vi "W7XBolo2021.vi"(1 "FPGA VI Reference In":refnum<k20>) -> (0 "FPGA VI Reference Out":refnum<k20>)   [LabVIEW 2014]
uses:
  W7XBolo_2021.ctl
  <vilib>/Platform/TimedLoop/XDataNode/timing_clust.ctl
  <vilib>/Platform/TimedLoop/XDataNode/nitl_modes.ctl
  <vilib>/Platform/TimedLoop/XDataNode/wakeup.ctl
  <vilib>/userdefined/High Color/nirio_resource_hc.ctl
  <vilib>/Utility/file.llb/Read From Spreadsheet File (I64).vi
  <vilib>/Utility/file.llb/Read From Spreadsheet File (DBL).vi
  <vilib>/FPGAPlugInAG/PCI-7813R/niLvFpga_Open_PCI-7813R.vi
  <vilib>/Utility/error.llb/Error Cluster From Error Code.vi
  <vilib>/rvi/errors/niLvFpgaAdjustHostInterfaceError.vi
  <vilib>/DAQmx/create/channels.llb/DAQmx Create Channel (AO-Voltage-Basic).vi
  <vilib>/DAQmx/write.llb/DAQmx Write (Analog 1D DBL NChan 1Samp).vi
  <vilib>/rvi/interface/common/niFpgaWaitOnOcc.vi
  <vilib>/httpClient/POSTBuffer.vi
  <vilib>/FPGAPlugInAG/PCI-7813R/niLvFpga_Close_PCI-7813R.vi
  <vilib>/Platform/TimedLoop/XDataNode/XDataNode.xnode
  <vilib>/rvi/interface/nirviOpenFPGA/nirviOpenFPGA.xnode
  FPGA Bitfiles/W7XBolo2017_FPGATarget_fmain2014_DACRangeVoltage.lvbitx
  f_main_2014.vi
  <vilib>/rvi/interface/nirviReadWriteControl/nirviReadWriteControl.xnode
  <vilib>/rvi/interface/nirviMethod/nirviMethod.xnode
  <vilib>/rvi/interface/nirviCloseFPGA/nirviCloseFPGA.xnode
  <vilib>/Platform/TimedLoop/XDataNode/XDNodeRunTimeDep.lvlib
  <vilib>/Analysis/NI_AALBase.lvlib
  <vilib>/httpClient/LabVIEWHTTPClient.lvlib
  NiFpgaLv.dll
  <vilib>/FPGAPlugInAG/PCI-7813R/niLvFpga_AcknowledgeIrq_PCI-7813R.vi
  <vilib>/FPGAPlugInAG/PCI-7813R/niLvFpga_ConfigureFifo_PCI-7813R.vi
  <vilib>/rvi/errors/niLvFpgaMergeErrorWithErrorCode.vi
  <resource>/objmgr/daqmx.rc
  <vilib>/DAQmx/configure/timing.llb/DAQmx Timing (Sample Clock).vi
panel:
  out "Time until Acqusition":dbl(slide)=60.0 scale=0.0..60.0
  out "DAQ Timer":dbl
  in  "Tab Control 7":T1(tab)
  out "sample time [s]":sgl=0.0016
  out "No. of Samples:":u32=26000
  out "Measured Time for DAQ [ms]":u32
  out "single channel voltage [V]":dbl format="%#_13g"
  out "experiment acqusition [s]":dbl=40.0
  out "predicted time [ms] to finalize DAQ":dbl
  out "real time P_rad [MW, V]":dbl format="%#_13g"
  in  "single channel signal factor":dbl=1.0
  in  "single channel number":i64
  in  "manual time of data acquisition for experiment [s]":dbl=10.0
  out "f_DAQ [kHz]":dbl=0.625
  in  "skip feedback":bool
  out "loop DAQ timing [ms]":dbl
  in  "local storage only":bool
  in  "Frequency Selection":u16(ring)=1 items=["0.8 ms", "1.0 ms", "1.6 ms", "3.2 ms", "6.4 ms"]
  out "current start time of VI":timestamp
  in  "Trigger Source":i32(slide)=3 scale=0.0..1.0
  out "number of nanoseconds with offset to 1904":i64
  out "start time POSIX [ns]":i64
  out "data acquisition wait\ntime [ms]":i32=-1
  out "Countdown Time [s]":dbl
  out "Calibration Time [s]":dbl
  out "Total wait time  [s]":dbl
  in  "time before experiment [s]":T2=5.0
  in  "time between VI start and points of interest [s]":dbl=60.0
  in  "time after experiment [s]":dbl=5.0
  out "Downtime after T0 until DAQ [ns]":i64
  out "DAQ start (POSIX) [ns]":i64
  out "final trigger time":i64
  out "Pre-samples (If -1, then no trigger) detected)":i32
  out "actual T_DAQ [ms]":dbl
  in  "DAC and AD Settings":i32(slide) scale=0.0..1.0
  in  "Global DAC Range [mV] Setting":u8(knob)=3 scale=0.0..3.0
  in  "DAC settings file location":path=path "C:/QSB_files/dac_settings.dat"
  out "input DAC settings":i64[](array[numeric])=[3, 3, 3, 3, 3, 3, 3, 3, 3, 3, 3, 3, 3, 3, 3, 3, 3, 3, 3, 3, 3, 3, 3, 3, 3, 3, 3, 3, 3, 3, 3, 3, 3, 3, 3, 3, 3, 3, 3, 3, 3, 3, 3, 3, 3, 3, 3, 3, 3, 3, 3, 3, 3, 3, 3, 3, 3, 3, 3, 3, 3, 3, 3, 3, 3, 3, 3, 3, 3, 3, 3, 3, 3, 3, 3, 3, 3, 3, 3, 3, 3, 3, 3, 3, 3, 3, 3, 3, 3, 3, 3, 3, 3, 3, 3, 3, 3, 3, 3, 3, 3, 3, 3, 3, 3, 3, 3, 3, 3, 3, 3, 3, 3, 3, 3, 3, 3, 3, 3, 3, 3, 3, 3, 3, 3, 3, 0, 0]
  out "kbolott_and_volume":dbl[][](array[numeric])=[[1e-05, 1e-05], [9.8364458e-05, 1.8160732], [0.00029863964, 770.25441], [0.00053910452, 1653.5432], [0.00071569496, 2554.7619], [0.00083348142, 3356.1809], [0.00092645429, 4021.9678], [0.00099241932, 4570.4466], [0.0010332482, 4989.6792], [0.0010552469, 5170.4882], [0.0010669981, 5192.5645], [0.001071534, 5152.6222], [0.0010766644, 5109.6704], [0.0010841289, 5094.9972], [0.0010884845, 5078.237], [0.0010888843, 5058.9416], [0.0010882289, 5056.581], [0.0010872861, 5078.1684], [0.0010832221, 5096.5196], [0.0010760805, 5113.7904], [0.0010685167, 5141.4566], [0.0010644166, 5189.7831], [0.0010539441, 5182.7365], [0.0010337779, 5034.6928], [0.00098716411, 4625.8518], [0.00091599422, 4090.3707], [0.00082376071, 3438.9665], [0.00070194108, 2659.5109], [0.00051785958, 1753.3355], [0.00030745544, 937.82125], [0.00014081292, 59.55205], [1e-05, 1e-05], [0.0, 0.0], [0.0, 0.0], [0.0, 0.0], [0.0, 0.0], [0.0, 0.0], [0.0, 0.0], [0.0, 0.0], [0.0, 0.0], [0.0, 0.0], [0.0, 0.0], [0.0, 0.0], [0.0, 0.0], [0.0, 0.0], [0.0, 0.0], [0.0, 0.0], [0.0, 0.0], [0.0019134875, 3474.3085], [0.0020594744, 3690.1455], [0.002175929, 3861.3028], [0.0022530617, 3956.5918], [0.0023492529, 4057.9903], [0.0024581424, 4205.0841], [0.0025383764, 4324.9746], [0.0025876415, 4417.9525], [0.0026676725, 4566.0612], [0.0027635964, 4770.6296], [0.0028188521, 4914.295], [0.0028263806, 4970.0105], [0.0028491244, 5014.7926], [0.0028762033, 5060.279], [0.0028430703, 4969.1072], [0.0027058578, 4592.2853], [0.0019047772, 4936.5706], [0.0023594746, 6388.5028], [0.0025094117, 6336.5413], [0.002569351, 6048.9284], [0.0026367277, 5794.3031], [0.002714522, 5668.1597], [0.0027530637, 5505.217], [0.0027520905, 5312.6378], [0.0027781484, 5183.8321], [0.0028283925, 5165.5044], [0.0028425709, 5118.655], [0.00281436, 5016.5122], [0.0027996491, 4909.784], [0.0027993913, 4845.125], [0.0027603692, 4728.4661], [0.0026886073, 4585.7454], [0.0026437627, 4495.4419], [0.0026242501, 4486.7206], [0.0025685332, 4434.986], [0.0024747416, 4324.8822], [0.0023915919, 4209.8149], [0.002319616, 4111.844], [0.0022042921, 3923.4955], [0.0020485146, 3644.5259], [0.0024033884, 3597.1969], [0.002066694, 2566.1598], [0.0017718795, 1878.4004], [0.0015136288, 1414.3006], [0.0013043692, 1094.5581], [0.0011378765, 882.65731], [0.00097324167, 712.97006], [0.00080739571, 571.52867], [0.0, 0.0], [0.0, 0.0], [0.0, 0.0], [0.0, 0.0], [0.0, 0.0], [0.0, 0.0], [0.0, 0.0], [0.0, 0.0], [0.0, 0.0], [0.0, 0.0], [0.0, 0.0], [0.0, 0.0], [0.0, 0.0], [0.0, 0.0], [0.0, 0.0], [0.0, 0.0], [0.0, 0.0], [0.0, 0.0], [0.0, 0.0], [0.0, 0.0], [0.0, 0.0], [0.0, 0.0], [0.0, 0.0], [0.0, 0.0], [0.0, 0.0], [0.0, 0.0], [0.0, 0.0], [0.0, 0.0], [0.0, 0.0], [0.0, 0.0], [0.0, 0.0], [0.0, 0.0]]
  in  "Path to kbolott and volume data file":path=path "C:/QSB_files/kbolott_and_volume_all_PV_new.dat"
  out "final channel\nselection size":i32
  out "final channel selection":i64[][](array[numeric])=[[0], [1], [2], [3], [4], [5], [6], [7], [8], [9], [10], [11], [12], [13], [14], [15], [16], [17], [18], [19], [20], [21], [22], [23], [24], [25], [26], [27], [28], [29], [30], [31]]
  in  "Read Channel Selection from file":bool
  in  "channel selection input":i32[][](array[numeric])=[[0]]
  out "file import":i64[][](array[numeric])
  in  "Path to channel selection file":path=path "C:/QSB_files/short.channel_selection.dat"
  out "taum [s]":dbl[](array[numeric])=[0.11537597448635277, 0.11755685958822219, 0.1164214694473907, 0.11697577239117866, 0.110451, 0.12010942076824872, 0.11766714993048435, 0.11910426529905502, 0.10999582403545866, 0.11118469600664964, 0.10580731993585431, 0.11217289808087993, 0.11223398365603839, 0.11204749607224823, 0.11263624992738425, 0.11091290284745299, 0.11721868902521211, 0.11737061531613151, 0.11788987597885038, 0.11600007869942867, 0.11334307549251021, 0.11228572042130423, 0.1129521332802642, 0.11724104097990388, 0.11740306056822605, 0.11529467898123245, 0.11828175507687082, 0.11829012392284373, 0.11773460668621359, 0.1155776803231521, 0.11650421728110884, 0.11571658330095998, 0.11068789319935994, 0.10986016888144867, 0.10999340462233435, 0.11095550249493497, 0.11143937038853975, 0.11095468517729823, 0.11130783288802211, 0.11084408945769118, 0.10830137260394793, 0.10662335345199567, 0.10535002662491703, 0.10738515206651872, 0.10772145508062766, 0.1053368317440755, 0.10408446186375701, 0.10449038510758271, 0.11178895597256559, 0.11021628063681403, 0.11220331344682449, 0.11111721341359461, 0.10889811436206044, 0.11638094730098773, 0.11290278568076087, 0.11205006536853761, 0.1094907553786962, 0.11634433136641531, 0.11037702264320227, 0.1104223688763365, 0.11352480237507033, 0.11341744936097128, 0.10916961452972393, 0.11332789199343518, 0.11107001747086552, 0.1083853978889723, 0.11029711206697901, 0.11063487469805744, 0.10926615257922916, 0.10988377001368325, 0.10782095764307568, 0.1073886205272185, 0.10829341805096283, 0.10953345610425252, 0.10953147401563214, 0.10933747673483066, 0.1093210854374169, 0.10892908051404164, 0.10841565534876087, 0.10934867623657209, 0.11431979794745441, 0.11469548527952493, 0.11256319960938391, 0.11004758193350624, 0.1086775698186096, 0.10860163257332957, 0.10972644811806966, 0.1244329993560779, 0.10848514148619942, 0.10753497988240919, 0.11378450261362759, 0.11397799701939393, 0.10865166632049855, 0.10955778865143037, 0.11184264538711042, 0.11080028199806266, 0.11230419705417591, 0.11150150302047147, 0.10940920103499238, 0.0, 0.11018788195565775, 0.1109851624674225, 0.10888498891279576, 0.10950524535111039, 0.11209787924272374, 0.11180887164622381, 0.1110290995583749, 0.11040609393156747, 0.1103438351320269, 0.1101975468642728, 0.10923728746964355, 0.0, 0.11021638606642407, 0.0, 0.0, 0.0, 0.0, 0.0, 0.0, 0.0, 0.5609466646481899, 0.0, 0.0, 0.0, 0.0, 0.0, 0.0, 0.4058686463981613, 0.11537597448635277]
  out "kappa [A²]":dbl[](array[numeric])=[0.0008396193201719739, 0.0008193409803026575, 0.0008327489337370494, 0.0008094925878469488, 0.00039367506543457065, 0.0008063058560714545, 0.0008451910365158945, 0.0007992358755606012, 0.0008323076933152601, 0.0008570762215527662, 0.0007628861690345087, 0.0008061906602308296, 0.0008540424353779365, 0.0008301118976821594, 0.0008577435335519969, 0.0008553747566925557, 0.000838644207815748, 0.0008273548270536888, 0.0008111923709406437, 0.0008317040544888235, 0.0002062919117538751, 0.0007971782754034694, 0.0007777938427968141, 0.0007983063012770449, 0.0007902138174646686, 0.0007777700527572154, 0.0008086241703327105, 0.0007894905085128677, 0.0008499052168857277, 0.0008231536154986703, 0.0008290108212352768, 0.0008015771948583539, 0.0004219784890145567, 0.0008028223447312654, 0.0007908997677950409, 0.0007688640721813007, 0.0007923143974006498, 0.0007943700234243013, 0.000794807683089336, 0.0007644407575630641, 0.0008256914284962689, 0.0008464663657085921, 0.0008525498714753285, 0.0008605939917038706, 0.0008075301142063146, 0.0008582080819176783, 0.0008833831995156997, 0.0008817750426330745, 0.0008736825873144331, 0.0008712555197947145, 0.0008599116319459445, 0.0008597288697454142, 0.0008850439198466119, 0.0008360600624626481, 0.0008729149198757765, 0.0008652970161905564, 0.000878176403644396, 0.000814669724061475, 0.0008492936703496222, 0.0008335090067364612, 0.0009020306039280142, 0.0009060889736233363, 0.000873120149823901, 0.0008865804075398461, 0.0008218319952538781, 0.0008647381541051004, 0.0008535415687509321, 0.000868609807906937, 0.0008544506047017487, 0.0008552184337763689, 0.0008772351584693919, 0.0008899531428744609, 0.0009049492537694576, 0.000908105157129488, 0.0009441675693280472, 0.0008666158415307141, 0.0008904383660716827, 0.00090533600441176, 0.0009193630525411423, 0.0009209094258700529, 0.0008671616817531277, 0.0008573033056411677, 0.0008894545060438134, 0.0008393076570230061, 0.0008809839906701387, 0.0008713273912310079, 0.0008529389904228485, 0.0008798583497112145, 0.0007606961064025662, 0.0007618681674480262, 0.0008830002472907413, 0.0008434447500347438, 0.0008157810403546725, 0.0008170412330426688, 0.000817539692314199, 0.0008060567476264818, 0.0007745714382802376, 0.0007738842512393123, 0.0007910139604008742, -1.9640688433259297e-10, 0.000780575223559956, 0.0007962779122750964, 0.000790630439080113, 0.0008189866992119251, 0.0008220353590981327, 0.0008259174124746273, 0.0008237041516630779, 0.0008128375228315313, 0.0008025139618430593, 0.0007891459070721132, 0.0007835394415130632, 1.4659311061625464e-11, 0.0007713911232202254, -1.136328152026204e-11, 7.33972615530204e-11, -5.807996136265078e-12, 1.50989391544806e-10, -2.091237015882531e-11, -2.2968171315336452e-11, 3.2003514158147334e-12, -1.18410213996469e-13, 3.9907860061368183e-13, 1.2900003061146403e-11, -7.996494711993759e-11, 1.2728268766879732e-10, -2.7124534936566837e-11, -1.0618681361847593e-11, 1.1300143559461795e-05]
  out "roh [Ohm]":dbl[](array[numeric])=[964.4665558152926, 984.0412138536651, 1001.0627256989599, 1012.7898525309201, 986.7279110070629, 993.5830261423998, 1133.718466702734, 1026.065541032409, 981.7525515631839, 976.6051330676225, 975.1369773387203, 983.6003740876943, 945.3052421117454, 944.0131212191011, 937.9865397688445, 924.775520494105, 1002.3909240348048, 1016.474188810108, 1008.3024841336951, 997.8517562562979, 1396.1357804303618, 1011.7052948010587, 1006.0858095523904, 1000.525119034801, 1016.071205963885, 1008.5531713944379, 1001.2101495655734, 1012.9539707105694, 909.9522463978296, 921.8611396886308, 930.8535575645451, 937.6736260749049, 1835.253905213153, 905.3151174073253, 915.4686408360067, 932.2842954450018, 878.6376527118448, 888.8892103361444, 896.5962281010978, 917.195767017641, 953.2009542047422, 949.8476734916919, 945.7180214798805, 934.1303098026676, 944.4309270141721, 922.393020385211, 908.2770101975661, 902.8479184676862, 997.7185120044248, 1004.633250147941, 1012.2992174178987, 1022.8972656361334, 988.1138139759116, 1012.5096483256309, 926.7526927543831, 940.6499588809413, 987.4981539235332, 1030.6093168535383, 996.69488158787, 998.6770565199763, 937.2653710614366, 942.0245103372197, 975.0990877775471, 954.8089604337308, 987.3564837474132, 941.2547128561528, 982.5095895382428, 979.0417371038707, 995.2373497220817, 994.8506309175264, 989.7979732647505, 986.9344569144992, 979.4724674608722, 951.8026661804106, 928.3096097998925, 980.4648125251251, 967.8736951300871, 960.399052288677, 950.3474867516031, 931.7877057694141, 925.6104123406642, 925.2905333073797, 925.2586242376997, 996.0089625341668, 969.8590336679081, 973.5395443351913, 978.7443359479869, 1329.6132687126426, 951.8837808548863, 946.7262849537287, 933.7058147126331, 940.8228530266879, 876.367589172054, 864.1420943242144, 855.6188139335973, 854.7591574173059, 955.1936774096923, 969.1826763753277, 970.8033011923455, 0.0, 935.2179320514933, 937.6581182076873, 940.1867678977421, 939.4080093580444, 850.4194498630884, 857.7406858104588, 867.3881837894808, 884.270800315495, 892.6618762043922, 899.3995556852765, 915.5186423922648, 0.0, 919.5685811076437, 0.0, 0.0, 0.0, 0.0, 0.0, 0.0, 0.0, 0.0, 0.0, 0.0, 0.0, 0.0, 0.0, 0.0, 0.0]
  in  "load calibration values from file?":bool
  in  "file location":path=path "C:/QSB_files/default_calibs.dat"
  in  "Clear all Values \nfrom Beginning":bool
  in  "Cancel Button":bool
  in  "Tab Control":T3(tab)=enum."offsets"
  out "real time P_rad array":dbl[](array[numeric])
  out "all plot":cluster{cluster{dbl, "element":dbl}[]}[](graph)
  out "full P_rad [MW] HBC":dbl[](array[numeric])
  out "single channel voltage array":dbl[](array[numeric])
  out "full P_rad [MW] VBC":dbl[](array[numeric])
  out "nsample array [s]":dbl[](array[numeric])
  in  "Tab Control 4":enum32{"1 to 64", "65 to 128"}(tab)
  out "Raw 33-64":T4={"Channels 33 - 40"={"tstart"=-1.0, "FPGSampleTime"=0.0007999999797903001, []}, "Channels 41 - 48"={"tstart"=-1.0, "FPGSampleTime"=0.0007999999797903001, []}, "Channels 49 - 56"={"tstart"=-1.0, "FPGSampleTime"=0.0007999999797903001, []}, "Channels 57 - 64"={"tstart"=-1.0, "FPGSampleTime"=0.0007999999797903001, []}}
  out "Raw 1-32":T5={"Channels 1- 8"={"tstart"=-1.0, "FPGSampleTime"=0.0007999999797903001, []}, "Channels 9 - 16"={"tstart"=-1.0, "FPGSampleTime"=0.0007999999797903001, []}, "Channels 17 - 24"={"tstart"=-1.0, "FPGSampleTime"=0.0007999999797903001, []}, "Channels 25 - 32"={"tstart"=-1.0, "FPGSampleTime"=0.0007999999797903001, []}}
  out "Raw 97 - 128":T6
  out "Raw 65 - 97":T7={"Channels 65 - 71"={"tstart"=-1.0, "FPGSampleTime"=0.0007999999797903001, []}, "Channels 73 - 80"={"tstart"=0.0, "FPGSampleTime"=0.0, []}, "Channels 81 - 88"={"tstart"=0.0, "FPGSampleTime"=0.0, []}, "Channels 89- 96"={"tstart"=0.0, "FPGSampleTime"=0.0, []}}
  in  "Tab Control 2":T8(tab)
  out "Offset 1-32":T5
  out "Offset 33-64":T4
  out "Offset 65 - 96":T7
  out "Offset 97 - 128":T6
  out "mean [µV]":dbl[](array[numeric])=[-1.0868261423893273, -7.990200226195156, -8.872255865484476, -10.064653429202735, 0.15312744089169428, -0.4802685623290017, 79.99756187200546, 3.8797607778105885, 7.466437983792275, -11.855529976077378, -14.755810303613544, 11.95750002656132, -8.815307591110468, 8.149265284650028, 8.269059924408793, -11.019621591083705, -12.155327236279845, 11.87860367167741, -6.231015749275684, -15.075639658607543, 0.0, 6.344313888344914, 3.639809527201578, 3.0874096516054124, 8.76988005079329, -7.264990275725722, -7.70126957911998, 7.049201687797904, -5.80584733793512, 7.595500641036779, 6.073078604415059, -7.225483466871083, 79.99756187200546, -6.537163232453167, -9.645444056019187, 12.285051323473454, 13.197480607777834, -16.88525196351111, 14.07000007852912, -16.506511248648167, 1.317087397328578, 1.08624508313369, 2.3623975100927055, -2.897617152426392, 15.83140585012734, -16.25518073886633, -15.617426818236709, 17.98624993674457, 3.7837353413924575, -9.388547336682677, 9.94124523550272, -6.121635691262782, -2.0081029990687966, 4.30479721352458, -4.133330153301358, -5.317026526667178, -11.655625252053142, -5.538921014405787, -8.435971749015152, 6.669389561749995, -1.8595410124398768, -2.53979729488492, -10.409289598464966, -6.292082520201802, 3.7355981967411935, -18.137234115973115, -4.700468767434359, 3.342731858836487, -12.631655607372522, 9.172075293958187, 6.846901873126626, -3.930554289836436, 1.7484496866818517, -16.44031921029091, -10.512590528465807, 12.021665379405022, -8.448259128257632, 13.529167225584388, 17.693245006725192, -4.355747113935649, -3.6723168953321874, 5.37680432992056, 10.893774300813675, -4.947795500513166, -8.853234618902206, -8.510966784320772, -8.374758321791887, -5.658979562111199, -2.2409302280284464, 2.758493692148477, 8.601340346038342, -7.293605968821794, 12.404243350028992, -12.006000837311149, -11.754489918239415, 9.409597270190716, -13.37633796967566, 12.256328152492642, 11.935139204375446, 0.7362792931962758, 5.519568009767681, -8.845417500473559, -12.099643769674003, 14.686545513570309, 3.346308583393693, -8.303696025162935, -8.65569824911654, 7.810756796039641, 1.5121240087319165, 0.011279296885732037, 1.614531259285286, -5.667829567566514, -3.9232958229258657, -6.169724114239216, -5.436516118235886, -6.255625001620501, -6.266003428958356, -4.911455085966736, -5.73839355725795, -4.92482177214697, -6.417814949993044, -5.6116870157420635, -5.524570322595537, -7.1842724503949285, -6.247446291614324, -5.192988283466548, -5.514289560727775, 0.007548827956270543] format="%10.6f"
  out "peak to peak [µV]":dbl[](array[numeric])=[7.324153557419777, 7.3248520493507385, 4.881992936134338, 7.3248520493507385, 7.32421176508069, 7.32421176508069, 0.0, 7.324153557419777, 7.324386388063431, 4.882924258708954, 4.882924258708954, 4.882924258708954, 7.323920726776123, 4.882924258708954, 4.882924258708954, 7.3248520493507385, 4.882924258708954, 7.323920726776123, 4.882924258708954, 7.323920726776123, 0.0, 12.207310646772385, 7.324153557419777, 7.324153557419777, 4.882924258708954, 7.324386388063431, 7.323920726776123, 7.323920726776123, 7.323920726776123, 7.323920726776123, 7.323920726776123, 7.324386388063431, 0.0, 7.324386388063431, 4.882924258708954, 4.882924258708954, 7.323920726776123, 7.323920726776123, 4.882924258708954, 24.413689970970154, 7.324153557419777, 4.882807843387127, 7.324153557419777, 7.324153557419777, 12.207776308059692, 9.765848517417908, 9.765848517417908, 9.765848517417908, 9.765848517417908, 7.3248520493507385, 9.765848517417908, 7.324386388063431, 7.324153557419777, 7.323920726776123, 7.324386388063431, 7.324386388063431, 4.882924258708954, 7.324386388063431, 9.765848517417908, 7.324386388063431, 7.324269972741604, 4.8826914280653, 9.765848517417908, 63.47661837935448, 4.882924258708954, 7.325783371925354, 7.324386388063431, 7.324153557419777, 4.882924258708954, 9.765848517417908, 7.323920726776123, 7.324386388063431, 7.324153557419777, 4.881992936134338, 4.882924258708954, 4.882924258708954, 7.323920726776123, 4.882924258708954, 4.883855581283569, 4.882924258708954, 7.324386388063431, 7.324386388063431, 7.323920726776123, 7.324386388063431, 7.323920726776123, 7.323920726776123, 4.882924258708954, 12.207310646772385, 4.8826914280653, 7.324386388063431, 4.882924258708954, 7.323920726776123, 4.882924258708954, 7.323920726776123, 7.323920726776123, 4.882924258708954, 4.882924258708954, 7.3248520493507385, 4.882924258708954, 7.32421176508069, 7.324386388063431, 4.882924258708954, 4.882924258708954, 7.323920726776123, 7.324386388063431, 7.323920726776123, 4.882924258708954, 4.882924258708954, 7.324269972741604, 7.324218586290954, 7.324269972741604, 78.12492549419403, 4.882924258708954, 124.51177462935448, 80.56638762354851, 107.42200538516045, 114.74592611193657, 119.62885037064552, 117.18738824129105, 75.68346336483955, 83.00784975290298, 61.03515625, 83.00784975290298, 80.56638762354851, 80.56638762354851, 75.68346336483955, 63.47661837935448, 4.882812390860636] format="%10.6f"
  out "standard deviation [µV]":dbl[](array[numeric])=[1.3036026797496636, 1.3420327341534157, 1.064632711189032, 1.3183644605739115, 1.370580330128604, 1.3863993208065881, 0.0, 1.3756086966919314, 1.3033635303128535, 1.3645315377351082, 1.0907459947011133, 1.2888566517284963, 1.3362613716194949, 1.1741803584062915, 1.2708577363467628, 1.3353586601127052, 1.1919876577257686, 1.3709838960885252, 1.2104925828693935, 1.133633608207629, 0.0, 3.0599605659652336, 1.381189113773974, 1.3710090729521511, 1.1825139240426916, 1.3291962023482355, 1.2972019555536811, 1.5752294600651209, 1.4348073556120489, 1.5350307313927734, 1.339050112533554, 1.4943583204888495, 0.0, 1.4508038195058017, 1.2325495603810572, 1.289912993666556, 1.3433062875107393, 1.3398822432734163, 1.534045727376026, 3.1309945215657233, 1.3451440535092256, 1.1094863880052617, 1.2848454782475338, 1.4392275103567735, 2.1646380895538133, 1.5764686908727295, 1.8587372491098588, 1.7701595206338636, 1.4747643858198207, 1.7496186198255672, 1.531828101370379, 1.3635429383539241, 1.3363276218458022, 1.510814829492694, 1.4399577231091554, 1.4124317371976478, 1.413580499133295, 1.3668612458750313, 1.6918175690194857, 1.1771696442371267, 1.666194415475469, 1.2881820616939266, 1.6825268941850453, 9.285962098288044, 1.2657962842879769, 1.5227901644120807, 1.2887960355191643, 1.3713397757888555, 0.9409861463314614, 1.5747829733155034, 1.4190235941294134, 1.2472383190291216, 1.295969883093782, 1.2892305818095295, 1.3174003964127896, 0.9534221803559357, 1.3315109646280372, 1.2489669475442673, 1.349904662109497, 1.4628494605003626, 1.1866585970205008, 1.3284762503162553, 1.3591765604379664, 1.440899156716539, 1.20561778948312, 1.4840990676246344, 1.377787118468021, 2.9371469283422225, 1.190473906695344, 1.5904378429312183, 1.2088317344047321, 1.3065369246410496, 1.2079090266634622, 1.4006134268721806, 1.256254801125801, 1.2249039770452999, 1.340159935658495, 1.4548630995535106, 1.390209079178451, 1.640652499453038, 1.2936869882511064, 1.2595058622741677, 1.2444275335713273, 1.460819197867702, 1.240339655773447, 1.236295738635732, 1.3148643594347451, 1.1965755092732067, 1.9037334286600238, 1.354045523248285, 1.343098779957647, 10.648064571198674, 1.085492843026454, 17.76111356002071, 15.186209919625934, 19.587547605945343, 21.06199734827501, 23.357782004272384, 18.34000258364854, 12.885928124829098, 18.63512720438761, 12.776721724893239, 13.06902962785174, 14.7813618767708, 14.660597879483435, 15.094471148412042, 10.816437200629686, 0.9119755118192763] format="%10.7f"
  out "offsets [V]":sgl[](array[numeric])=[-0.0010868261, -0.0079902, -0.008872256, -0.010064653, 0.00015312745, -0.00048026856, 0.07999756, 0.0038797609, 0.0074664378, -0.01185553, -0.014755811, 0.0119575, -0.008815307, 0.008149265, 0.0082690595, -0.011019622, -0.012155327, 0.011878604, -0.0062310155, -0.01507564, 0.0, 0.0063443137, 0.0036398096, 0.0030874095, 0.00876988, -0.0072649904, -0.0077012694, 0.0070492015, -0.0058058472, 0.0075955004, 0.0060730786, -0.0072254837, 0.07999756, -0.006537163, -0.009645444, 0.012285051, 0.013197481, -0.016885253, 0.0140700005, -0.016506512, 0.0013170874, 0.001086245, 0.0023623975, -0.0028976172, 0.015831405, -0.016255181, -0.0156174265, 0.01798625, 0.0037837354, -0.009388547, 0.009941245, -0.006121636, -0.002008103, 0.0043047974, -0.00413333, -0.0053170267, -0.011655625, -0.005538921, -0.008435972, 0.0066693895, -0.001859541, -0.0025397972, -0.01040929, -0.0062920824, 0.0037355982, -0.018137233, -0.004700469, 0.0033427319, -0.012631656, 0.009172075, 0.006846902, -0.0039305543, 0.0017484496, -0.016440319, -0.01051259, 0.012021665, -0.008448259, 0.0135291675, 0.017693246, -0.0043557473, -0.003672317, 0.005376804, 0.010893774, -0.0049477955, -0.008853234, -0.008510967, -0.008374758, -0.0056589795, -0.0022409302, 0.0027584936, 0.00860134, -0.007293606, 0.012404243, -0.012006001, -0.0117544895, 0.009409597, -0.013376338, 0.012256328, 0.011935139, 0.0007362793, 0.005519568, -0.008845418, -0.012099644, 0.014686545, 0.0033463086, -0.008303696, -0.008655698, 0.0078107566, 0.001512124, 1.1279297e-05, 0.0016145313, -0.0056678294, -0.003923296, -0.0061697243, -0.005436516, -0.006255625, -0.0062660035, -0.004911455, -0.0057383934, -0.0049248217, -0.006417815, -0.005611687, -0.00552457, -0.0071842726, -0.0062474464, -0.005192988, -0.0055142897, 7.548828e-06]
  in  "Tab Control 5":T9(tab)
  out "MessCal 17-32":T10
  out "MessCal 1-16":T11
  out "MessCal 49 - 64":T12
  out "MessCal 33 - 49":T13
  out "MessCal 81 - 96":T14
  out "MessCal 65 - 80":T15
  out "MessCal 113 - 128":T16
  out "MessCal 97 - 112":T17
  out "rohM [Ohm]":dbl[](array[numeric])=[955.9210569003584, 975.2225867678288, 992.437036560495, 1003.9150041232155, 964.6709267361214, 984.9572576185153, 1109.7902651791405, 1017.3971751835443, 973.4625288588265, 968.2502632137221, 966.3109252226336, 974.9039174556738, 937.1961165636667, 935.629152331029, 929.8777653560232, 916.6273213641874, 993.8600077425886, 1007.747220175482, 999.538757797739, 989.259326518511, 1376.2474702792624, 1002.9820261662712, 997.0827639584581, 991.8298513828715, 1007.3959263962993, 999.731688473045, 992.5694713810915, 1004.2278313387544, 901.7408614557748, 913.5263201644023, 922.6000347220167, 929.1324124673284, 1861.6154176027044, 1093.927196836436, 1007.9363359277321, 1036.4338892880046, 870.0841248686661, 1050.5167797933268, 835.6422839385561, 972.7302854337263, 859.3011786817983, 961.6092048210389, 1047.3928187757283, 988.832793437985, 1048.3205426549248, 914.332942804887, 900.3157849297525, 895.00814421823, 1071.5906890853698, 1240.680912945196, 1118.5865173282953, 1136.2368012115553, 979.6020495367086, 1184.5954182960481, 917.6449067403735, 1078.5806173219855, 979.3199545918619, 1128.0894920220258, 1107.186057046148, 1058.3166942556252, 1023.6083043326868, 933.59856277125, 966.8256448468209, 946.8606222101016, 979.3205494354647, 933.3840253846747, 974.5533501983803, 971.1794214902197, 987.0554817952572, 986.5749021706774, 981.6986292217362, 978.7347622591474, 971.5484218656636, 944.047973258107, 920.6032902860329, 972.4402748798641, 959.984233512531, 952.591197650364, 942.5919944057227, 924.0279269016532, 914.8529393815768, 917.1478717227278, 917.2337651779903, 987.7775960990439, 961.9031159853596, 965.4373993129607, 970.4632555320065, 1320.2877978597037, 943.1885046031139, 937.9468788829204, 925.7648958682478, 932.8248830697123, 867.8130427511578, 855.5281600301191, 847.1255690825355, 846.1703092127094, 946.4268675021895, 960.4551490506069, 962.1034228215849, 0.0, 926.3189738746476, 928.9034427126842, 931.5953365503219, 930.8922256947712, 841.8622295070686, 849.6900749449139, 858.8923632084177, 875.6587455837807, 884.1647613529192, 890.7709945330058, 906.8409537813054, 0.0, 910.8341169118078, 0.0, 0.0, 0.0, 0.0, 0.0, 0.0, 0.0, 0.0, 0.0, 0.0, 0.0, 0.0, 0.0, 0.0, 0.0]
  out "kappaM [A²]":dbl[](array[numeric])=[0.0009300671270220562, 0.0008996956373935807, 0.0009113297442037162, 0.0008867590824243674, 0.0009228130637662335, 0.000892376467301951, 0.0009770254811961566, 0.0008792308275001902, 0.0009310256041664582, 0.0009423185323272868, 0.0008572434937303331, 0.0008920046513574609, 0.0009420929356066393, 0.000917506962215698, 0.0009460997409387052, 0.0009375108227429941, 0.0009243758742815039, 0.0009114349813263648, 0.000900921530637464, 0.0009125939448337885, 0.00024194293733649212, 0.0008862811148346745, 0.000860786457985191, 0.0008899499474378734, 0.0008705292947452343, 0.0008562533252789487, 0.0008845638677383653, 0.0008733756860620295, 0.0009371291360660496, 0.0009161990069047479, 0.0009134962955644435, 0.000899493342343606, 0.00048738710715928865, 0.0009162872261249577, 0.0009180994946649499, 0.0008862330742697767, 0.0008788280646144513, 0.000923989577633034, 0.0007960035497604953, 0.0008432936364276662, 0.0008626191144435472, 0.0008753403360820782, 0.0009785187528356617, 0.0009920297175945603, 0.0009357728927457351, 0.0009432876940863556, 0.0009737159021657041, 0.0009829677334712832, 0.0009797149193563025, 0.0009656693192116038, 0.0009657204661571637, 0.0009613114786807839, 0.0009574110075363582, 0.0009381886977305131, 0.0009666490144497014, 0.0009794202295580398, 0.0009619800496901404, 0.0009109830431199077, 0.0009578361472746666, 0.0009379291618002864, 0.001016572914013983, 0.0009750425932505828, 0.0009435677239603997, 0.0009695879318732844, 0.0008913866589398846, 0.0009419361616918934, 0.0009250842516270034, 0.0009429046775538786, 0.0009248119474557008, 0.0009298684481160537, 0.000983883219096257, 0.0009529385496771803, 0.00097924891843905, 0.0009817402563716065, 0.0010247538574068172, 0.0009415670186613855, 0.0009827266209943746, 0.0009926770422248304, 0.0009977894534251687, 0.0010016701651269853, 0.0009429727126362719, 0.0009280049111574535, 0.0009664607320996164, 0.000917092855553135, 0.0009689593754395974, 0.0009492630365830234, 0.0009304943986612507, 0.0009838563142093555, 0.0008327174235962352, 0.0008401872142169503, 0.0009608982361607494, 0.0009139859734154169, 0.0008951925851238197, 0.0008976799685850949, 0.0008951491596994188, 0.0008807724921218027, 0.0008598244382888369, 0.0008631925259468964, 0.000869388233684094, -3.087356377393487e-10, 0.000862230960556987, 0.0008818386198612574, 0.000875693256825492, 0.0009093335647258491, 0.0009117694962109967, 0.000915854945030498, 0.0009176622004345077, 0.000899838713726951, 0.0008882426814116755, 0.0008802823610482786, 0.0008643029460286225, 4.560949191370883e-11, 0.0008497040644528844, -2.015502496075528e-12, -1.3937728135220623e-10, -5.142335332617439e-12, -2.4405360432876065e-10, -3.025693723352094e-11, 5.446823850795443e-11, -9.461258601384958e-13, -1.11152298414936e-16, -1.7779007167808036e-13, -1.247134363192558e-12, 9.029112608459833e-11, 2.859966433855044e-10, 4.025476559655337e-11, -6.6296064908001744e-12, 2.7789638144048405e-05] format="%10.4e"
  out "TauM":dbl[](array[numeric])=[0.10247326273143675, 0.10385139756960429, 0.10373232144795708, 0.10311875959492485, 0.1040387663981229, 0.1046650716638566, 0.10127197371489062, 0.10433939668939028, 0.09961240211936159, 0.10113688577012743, 0.09820100289764892, 0.10095901838579123, 0.10145991266213297, 0.10133898562095205, 0.10130127833216106, 0.09956334469474118, 0.10358378126227558, 0.1033444650149854, 0.10368122845865657, 0.1024629201687842, 0.10726822954303422, 0.10182022977214773, 0.10234341921814957, 0.10309722284273504, 0.1042952251760315, 0.10251907726247211, 0.10376892017069193, 0.10390613836510422, 0.10393962152806514, 0.10278682866750612, 0.1029066416867304, 0.102809145991027, 0.10885131092677319, 0.09862497604372066, 0.10044854636642224, 0.1011397796494332, 0.10002902352125999, 0.09964990042145319, 0.10015936689391987, 0.10006472096945454, 0.09839726301474191, 0.0989699304142558, 0.1002391552504395, 0.10013350870556857, 0.10080436633835735, 0.09779852218595043, 0.09742571115181148, 0.09710433370493086, 0.10444501045101653, 0.1003366401072974, 0.10437315691375147, 0.10384291417884778, 0.10124021541103015, 0.10550745222701648, 0.1035137865735804, 0.10352859881892808, 0.1012417667717822, 0.1059159267079176, 0.10317764912629153, 0.10345604684447908, 0.1049337703539443, 0.10334536377187596, 0.1011439242990685, 0.10281039287381427, 0.10222071286894058, 0.10128943771143158, 0.10126644136767568, 0.10213051552429299, 0.10166794227392674, 0.10164755793457868, 0.10028065773083647, 0.1039274155284877, 0.10062166309448936, 0.10100667896022858, 0.10122793031614634, 0.1020869722455638, 0.10086834901007827, 0.10107073060568635, 0.10100593381229647, 0.1013148799331511, 0.10336010473304796, 0.104020047148851, 0.10319519163947051, 0.1023647743297228, 0.10121262984849082, 0.10131571623308212, 0.10129251089534078, 0.10505043416568437, 0.10066202738446095, 0.10001990246198598, 0.10320829246582676, 0.10342094956544687, 0.10072458787609094, 0.10113661913958252, 0.10213104126735983, 0.10141193462449195, 0.10097352152629059, 0.1005352087055146, 0.09991412160243203, 0.0, 0.09971962753116924, 0.10038664478845472, 0.0996831725438015, 0.0987164166127979, 0.10070743969491262, 0.10083769719722958, 0.09991070137880578, 0.09976037466686079, 0.09975950391708734, 0.0997863315853558, 0.09952725945462769, 0.0, 0.09982037400508142, 0.0, 0.0, 0.0, 0.0, 0.0, 0.0, 0.0, 0.0, 0.0, 0.0, 0.0, 0.0, 0.0, 0.0, 0.0] caption="tauM [s]" format="%10.4f"
  out "AmplitudeMeas":dbl[](array[numeric])=[4.884814572518217e-05, 4.7976679783762886e-05, 4.524764340004093e-05, 4.5151806191065595e-05, 4.809080266257478e-05, 4.7145047982970675e-05, 3.146231756322816e-05, 4.3987625115634926e-05, 4.655055771375242e-05, 4.66273477175114e-05, 5.1615426947301555e-05, 4.843928946738043e-05, 5.074259168837904e-05, 5.235508979961122e-05, 5.155588261265355e-05, 5.399794598550638e-05, 4.443179014704798e-05, 4.3474037919468324e-05, 4.4937934344410205e-05, 4.556235086224266e-05, 7.358960331887751e-05, 4.528620525296725e-05, 4.7375341050864565e-05, 4.642857602638946e-05, 4.5595717685851076e-05, 4.7302741586246765e-05, 4.6625975104004555e-05, 4.581918862013139e-05, 5.634340629289198e-05, 5.576445138256422e-05, 5.452694873767264e-05, 5.4394617922290445e-05, 1.5640753900925838e-05, 3.4876244036040754e-05, 4.3131880431277286e-05, 4.157013788164736e-05, 6.594026050113745e-05, 3.846074258536254e-05, 8.092036434813877e-05, 5.15919193318786e-05, 6.938738199638531e-05, 5.117058828178776e-05, 3.656914680495611e-05, 4.190030926295942e-05, 3.8177482970664205e-05, 5.400781436437592e-05, 5.4404204763341695e-05, 5.470539183413758e-05, 3.440187451106315e-05, 2.3688059308740418e-05, 3.1179877554395444e-05, 3.0056387787071678e-05, 4.451276294761954e-05, 2.758635976953778e-05, 5.2189063074364834e-05, 3.382999969429794e-05, 4.433078241643989e-05, 3.2349556560738134e-05, 3.2300748490518005e-05, 3.7152975410132973e-05, 3.735580097349016e-05, 4.948433878422281e-05, 4.6742566329426626e-05, 4.79882648013434e-05, 4.790771836666737e-05, 5.1287893849813555e-05, 4.671903980322345e-05, 4.623427665213439e-05, 4.521107284722498e-05, 4.501779229445353e-05, 4.30551070148025e-05, 4.4828312823474215e-05, 4.44446374507222e-05, 4.774895836610016e-05, 4.8769768288348895e-05, 4.6145596903899056e-05, 4.567972066843394e-05, 4.612705469829869e-05, 4.7154624740959475e-05, 4.944003667941568e-05, 5.394723576121702e-05, 5.448269442335658e-05, 5.225966317746918e-05, 4.551186565071207e-05, 4.610146443391865e-05, 4.6630362792763434e-05, 4.69519837192857e-05, 1.9681004304892295e-05, 5.6612358154279806e-05, 5.691291067414257e-05, 5.132973551498099e-05, 5.296970989083297e-05, 6.514064070696284e-05, 6.736516743145396e-05, 6.92823951303374e-05, 7.06443959549654e-05, 5.430635287521875e-05, 5.2067117003992196e-05, 5.145931439129173e-05, -3.1793762011223885e-07, 5.7242295451644905e-05, 5.554183170240005e-05, 5.552348413500266e-05, 5.353198650115e-05, 6.907674687371533e-05, 6.715920529459659e-05, 6.520750725303529e-05, 6.332147469482486e-05, 6.259754438105115e-05, 6.198157003306498e-05, 6.0316992950063626e-05, 3.495440865528331e-07, 6.0686411438686236e-05, -7.284208164373995e-07, -3.0307954598728734e-07, -3.3162749704529687e-07, -3.250653244446207e-07, -3.4500887828612614e-07, 3.5391304443528806e-07, -5.696407161148624e-07, 3.827735480530181e-07, 4.345734938552804e-07, 1.1320226330949104e-06, 2.005101510462144e-06, 3.0673371184281807e-07, 1.2170619844306492e-06, -3.398933905177686e-07, 2.9714440268932945e-07]
  out "DampingMeas":dbl[](array[numeric])=[-9.758643116700723, -9.629143404928858, -9.640196864790152, -9.697556525391104, -9.61180177947633, -9.554285724005522, -9.874400224639485, -9.584107554090206, -10.038910604743169, -9.887589403067894, -10.183195389992717, -9.905009141221385, -9.856109410719231, -9.86787063115469, -9.871543740258218, -10.043857034594167, -9.654021004195494, -9.67637695792412, -9.644947449660622, -9.759628149897827, -9.322424768825114, -9.821231028821972, -9.771023947015639, -9.699582320712988, -9.58816665204165, -9.754282097562905, -9.636796820811824, -9.624070490293954, -9.620970187292688, -9.728872978801503, -9.717545763899397, -9.726761081035322, -9.186843883513017, -10.139419446415864, -9.955345658782756, -9.887306492718903, -9.997098489994375, -10.035132958193246, -9.984088668003597, -9.993532089149152, -10.16288430553378, -10.104079045163786, -9.976141533730807, -9.986666930251976, -9.920205208606001, -10.225103382427779, -10.26423095276946, -10.298201551319856, -9.574416199316559, -9.966448935609424, -9.581007507767039, -9.629930052595677, -9.87749775067201, -9.47800348593706, -9.660548928805468, -9.659166755931894, -9.87734639453879, -9.441450696623575, -9.692021561530053, -9.665940566076877, -9.529820539440967, -9.676292806007195, -9.88690133322432, -9.726643115033745, -9.782753142038072, -9.872697712558626, -9.874939678873723, -9.791392855175962, -9.835942162630502, -9.837914656480084, -9.972012775226327, -9.62210014474851, -9.938217767887062, -9.900335406470996, -9.87869649094757, -9.795569189715636, -9.913912637750073, -9.894061257965607, -9.900408443907281, -9.870218477876234, -9.674912797183572, -9.613531500990536, -9.690373980734156, -9.768985537729442, -9.8801898685662, -9.8701370051952, -9.872398177918972, -9.519237192516607, -9.93423265935898, -9.998010149830575, -9.68914392543709, -9.669220831966737, -9.928062463061918, -9.887615470118313, -9.791342451725214, -9.86077234107405, -9.903586453995555, -9.946764052872032, -10.008595221195026, -0.04313763282748088, -10.028116076621238, -9.961484439561707, -10.031783444297911, -10.130027348160011, -9.929752985771879, -9.916926187277847, -10.008937843490424, -10.02402009153829, -10.024107586091501, -10.0214125934133, -10.047498599676386, -0.6129351216480721, -10.017994923051424, 0.5637780520462315, 0.10978744631452035, 0.5025353454646939, 0.1910230592818031, 0.31086905931373493, 0.2701712879890733, 0.3997070190467916, -0.1402110488088746, -0.36927368560800944, -0.9431888525901574, -0.46217550051667494, -0.33808673480660545, -0.45825903308817845, 0.2851028761639094, -0.17618214991090886]
  in  "Tab Control 15":enum32{"kappaM [A²]", "rohM [Ohm]", "tauM [s]"}(tab)
  out "kappa_meas":cluster{cluster{dbl, dbl}[]}[](graph)
  out "Rmeas":cluster{cluster{dbl, dbl}[]}[](graph)
  out "tau_meas":cluster{cluster{dbl, dbl}[]}[](graph)
  in  "Tab Control 3":T9(tab)=enum."97 to 128"
  out "RefCal 17-32":T10
  out "RefCal 1-16":T11
  out "RefCal 49 - 64":T12
  out "RefCal 33 - 48":T13
  out "RefCal 65 - 80":T15
  out "RefCal 81 - 96":T14
  out "RefCal 113 - 128":T16
  out "RefCal 97 - 112":T17
  out "tauR [s]":dbl[](array[numeric])=[0.10292315835357112, 0.10199272403695953, 0.10475723294798765, 0.10414819613838391, 0.10387907456908113, 0.10420736881237311, 0.103706568442645, 0.10454999926363777, 0.10067406983111478, 0.10102975505384852, 0.09874353117086729, 0.10040584588306813, 0.10153735621262386, 0.10099019339023692, 0.10045519629639574, 0.1012778636584879, 0.10386355092876007, 0.10372072386082845, 0.10420809088364472, 0.10260629843982476, 0.1479397245408231, 0.10298761609630228, 0.10199112190395622, 0.10378008083073056, 0.10403768235155286, 0.10287961748698402, 0.10443967781666794, 0.10349133443663402, 0.10389037347180505, 0.10292103911369532, 0.10381016378004426, 0.10291167813587834, 0.10095931716806164, 0.09778559469706383, 0.10070172494088425, 0.10101362262178354, 0.10089590213958652, 0.10068417571048587, 0.10027342486802274, 0.1001580148556835, 0.09844078753380402, 0.09855035919543022, 0.10141076521650685, 0.09942661978605821, 0.100044898453749, 0.09843709497312675, 0.0981706617700702, 0.09739033951036816, 0.10579066150165929, 0.10003676894960246, 0.10330538590073358, 0.1043865432442743, 0.1018657436251196, 0.10506556777663303, 0.1039941797472394, 0.10383520947481932, 0.10231334831583622, 0.1061930390378222, 0.10374353015321205, 0.10333403635897148, 0.10431471177356995, 0.10320469195416845, 0.10192370966573754, 0.1032954320172502, 0.1023703130382756, 0.10130836278464572, 0.1020846673388746, 0.10178346111061455, 0.1018337998015322, 0.1018370724659081, 0.10192632813002919, 0.1001119276380221, 0.10098331608408057, 0.10123109259340747, 0.10129713566118832, 0.10216660844261771, 0.10117214382327544, 0.10081211888977323, 0.10198174919879018, 0.1017954675749366, 0.10512035510575353, 0.10258538460215058, 0.10201683357819019, 0.10238920479886968, 0.10211647468588146, 0.10136271634450558, 0.10197441111867332, 0.10437309491921805, 0.10013944794913852, 0.10096667914558943, 0.10278444976940188, 0.10443784509167334, 0.1014058881666478, 0.1018136137122912, 0.10197066776866164, 0.10287778507695343, 0.10113021738229896, 0.1006644626432808, 0.09960874275205062, 0.0, 0.10045362499432091, 0.09997878995335553, 0.09968196495402348, 0.09929009836131342, 0.10129697478598067, 0.10074502421507037, 0.09994878726727208, 0.10010044264701065, 0.09958730925413367, 0.10026435038467114, 0.10027859691998338, 0.0, 0.09991786391447231, 0.0, 0.0, 0.0, 0.0, 0.0, 0.0, 0.0, 0.0, 0.0, 0.0, 0.0, 0.0, 0.0, 0.0, 0.0] caption="TauM" format="%10.4f"
  out "kappaR [A²]":dbl[](array[numeric])=[0.0009394546099408418, 0.0009123589959054041, 0.0008944834435273222, 0.0008770375520480372, 0.0009239963605895957, 0.0008890166300778485, 0.000870129447553066, 0.0008803438703556952, 0.0009107267410723152, 0.0009482118897726593, 0.0008393896084479604, 0.0009035861563965376, 0.0009331871645677263, 0.0009165298742846952, 0.0009516053712712882, 0.0009263278749958205, 0.0009128662815217666, 0.0009141818400495597, 0.000909789371266667, 0.0009059436540468002, 0.0006415370912951529, 0.0008770271810778616, 0.0008565132360134204, 0.000876052272304057, 0.0008638409404951507, 0.0008565665929339299, 0.0008752621730157705, 0.0008723574002536088, 0.0009386669831268589, 0.0009024637518016725, 0.0009106667364475278, 0.0008776276917126037, 0.0009485343911843268, 0.0009151723308720066, 0.0009102916414683612, 0.0008907100933340703, 0.0008832933059746842, 0.0009116353873268474, 0.0007958923399951672, 0.0008390839738911967, 0.0008560973972353745, 0.0008799561494103719, 0.0009830927394652617, 0.0009984988903108173, 0.0009570093031431591, 0.0009303145524909112, 0.0009567590358007552, 0.0009837178264969402, 0.0009843129272350832, 0.0009650264028644321, 0.0009811549948605396, 0.0009642750489135812, 0.000950546683123411, 0.0009431266396382227, 0.0009370548549423619, 0.0009861255596051212, 0.000936829703479727, 0.0009133902647257256, 0.000940402507731474, 0.0009449250051295195, 0.001020427897586195, 0.0009849350172889812, 0.000930313608683439, 0.0009687273302019695, 0.0008970028098137427, 0.0009378049457091181, 0.0009124758988977847, 0.0009386195899888698, 0.0009190062218545321, 0.0009333611210404984, 0.0009621798885820149, 0.0009586958426847128, 0.0009811222363501687, 0.0009835686640004752, 0.0010203977936138304, 0.0009337778675467259, 0.0009650559425072165, 0.000973981534077398, 0.0009635053537147022, 0.0010018111126099767, 0.000933161139102181, 0.0009446919394286867, 0.0009889617815545281, 0.0009054358331810502, 0.000939122203155497, 0.0009357326744797564, 0.0009347689539899098, 0.0009859635267754768, 0.0008285938918540566, 0.0008263493838778397, 0.0009610579572422135, 0.0009149809143467651, 0.0008962067788812194, 0.0008856272930870661, 0.0008865350962852511, 0.0008786825089554866, 0.0008531311914735494, 0.0008533859891198841, 0.000872109802646621, 0.0, 0.0008760398523230332, 0.0008698446766384849, 0.0008609903717441008, 0.000917336684185368, 0.0009109179911288096, 0.0009047951430703002, 0.0009040380219105915, 0.000904172339632746, 0.0008882497394240699, 0.0008680572225687603, 0.0008687146922181975, 0.0, 0.0008532428573888429, 0.0, 0.0, 0.0, 0.0, 0.0, 0.0, 0.0, 0.0, 0.0, 0.0, 0.0, 0.0, 0.0, 0.0, 0.0] format="%10.4e"
  out "rohR [Ohm]":dbl[](array[numeric])=[956.2989572160357, 978.5138361759319, 995.9442187225984, 1008.0612479776369, 964.5336300299568, 985.0055115328407, 1004.8872607781536, 1015.6348863841632, 970.1222108210756, 972.8684444511352, 972.0803308285506, 969.9635452071706, 940.4965770667643, 932.2838721500672, 926.5761973455059, 920.756728380192, 998.751618187049, 1002.645484442407, 1002.1053527592385, 995.4297427495583, 1392.257972279243, 1000.0408343872241, 995.4529906568217, 990.3892250143565, 1003.5638240476669, 1002.755127561061, 995.6971596757855, 1001.1091797833428, 903.8420325055714, 910.3815361921353, 920.1088899075633, 931.7459469784179, 926.9075240023208, 1097.1836989420253, 1012.1223252323492, 1031.6051502195423, 865.2324519228997, 1057.9499680316503, 830.6654020548849, 979.3828138858556, 858.7479663219067, 961.53773070908, 1046.5061278621247, 990.1818658724626, 1041.8555133387686, 920.4757081714, 906.1159528601476, 888.1121509383381, 1071.2473928215386, 1245.318995975411, 1113.9727919488028, 1138.9397717522506, 979.7240200508488, 1182.6306291953856, 918.4536457413244, 1080.9233560093503, 983.3365096085471, 1130.6202259639726, 1110.4178701762908, 1055.259800570412, 1024.0859269214227, 933.9597358439946, 970.2526336349497, 948.688421711014, 977.030945115165, 939.7429827751671, 975.6234204561338, 969.0235139852646, 991.5720828131982, 982.0367763892792, 978.0405497108788, 979.6777686598148, 970.1725242379728, 949.966637895026, 923.9935019418235, 966.6891261032167, 962.6515819439619, 946.3793377124441, 934.8713576429398, 924.9716858464726, 928.4919275009711, 914.4598679734345, 912.3387254132956, 989.0534287066091, 964.630020750574, 968.107058502228, 973.1214347577088, 1322.3134987131093, 943.3174526896092, 936.0860474391636, 921.668159103662, 934.9229484511964, 862.561130391307, 859.1572250426, 850.5913397590812, 841.993390963776, 951.6785132163961, 955.3620398061908, 957.1846902791526, 0.0, 924.2040160146751, 932.2074075745045, 936.2132007459005, 925.1445913956145, 840.5542054379803, 852.5611786313709, 861.92116699029, 872.8124148817855, 883.4410079612458, 890.6206279927792, 906.1980264444114, 0.0, 911.9549549093531, 0.0, 0.0, 0.0, 0.0, 0.0, 0.0, 0.0, 0.0, 0.0, 0.0, 0.0, 0.0, 0.0, 0.0, 0.0]
  in  "Tab Control 16":enum32{"kappaR [A²]", "rohR [Ohm]", "tauR [s]"}(tab)
  out "kappa_ref":cluster{cluster{dbl, dbl}[]}[](graph)
  out "Rref":cluster{cluster{dbl, dbl}[]}[](graph)
  out "tau_ref":cluster{cluster{dbl, dbl}[]}[](graph)
  out "AmplitudeRef":dbl[](array[numeric])=[4.83014587536764e-05, 4.6886431105424204e-05, 4.5693921662628275e-05, 4.517336188419036e-05, 4.804578645848785e-05, 4.732052700919899e-05, 4.591462943673503e-05, 4.413030415869068e-05, 4.803400604811675e-05, 4.5764127555017504e-05, 5.1926839092191126e-05, 4.844133421698066e-05, 5.0773250468378564e-05, 5.2898883999341665e-05, 5.1723916149280746e-05, 5.4034050297686275e-05, 4.443055762286131e-05, 4.391815377009177e-05, 4.41959369950802e-05, 4.5166208362337964e-05, 2.628711953935288e-05, 4.612446065855897e-05, 4.781954999466934e-05, 4.73577474417948e-05, 4.641429262683351e-05, 4.691436453050651e-05, 4.674626195998729e-05, 4.6247085662862315e-05, 5.591386395664718e-05, 5.71360494619428e-05, 5.508233623570734e-05, 5.537540853138137e-05, 5.184686539494168e-05, 3.464714893108982e-05, 4.304066034843922e-05, 4.186592788449239e-05, 6.654390853603804e-05, 3.827642570591026e-05, 8.217344319552989e-05, 5.0945399304559355e-05, 7.00443785224149e-05, 5.090667782131817e-05, 3.647718767429366e-05, 4.1477186668356055e-05, 3.7926234807134086e-05, 5.384012806677711e-05, 5.4482177824064506e-05, 5.575719576332571e-05, 3.426765322518995e-05, 2.3469140674068706e-05, 3.101904807703416e-05, 2.9775225526311722e-05, 4.48253977632181e-05, 2.7561335436541732e-05, 5.374860766352849e-05, 3.340579086181422e-05, 4.5060685174598033e-05, 3.207264098912411e-05, 3.265621632092434e-05, 3.715427754438422e-05, 3.7167284327577756e-05, 4.892923984171913e-05, 4.69877213718141e-05, 4.7792882712276665e-05, 4.7892459709366624e-05, 5.062311324567015e-05, 4.72418138266528e-05, 4.671766101666083e-05, 4.4964820509280574e-05, 4.538680988286842e-05, 4.447204942236181e-05, 4.444314438676128e-05, 4.4521553353020214e-05, 4.689518527497801e-05, 4.852066998003178e-05, 4.725895157287671e-05, 4.619814121076748e-05, 4.7830609481071116e-05, 4.9912436159152e-05, 4.9303191216113085e-05, 5.248639863617162e-05, 5.390665512798289e-05, 5.1755140399867196e-05, 4.595398847286793e-05, 4.724546540554775e-05, 4.697955221093076e-05, 4.640292765818111e-05, 1.9557850098468774e-05, 5.6880091327731996e-05, 5.818509150594947e-05, 5.1910718940191176e-05, 5.260497806350283e-05, 6.60825738985255e-05, 6.757006053362133e-05, 6.924763793780627e-05, 7.171523683417315e-05, 5.3962547953454505e-05, 5.340882211661125e-05, 5.198165527945615e-05, 3.027720682637124e-07, 5.665392367532961e-05, 5.580997330836715e-05, 5.577479800735162e-05, 5.390989869183955e-05, 6.941708190788706e-05, 6.741760220225805e-05, 6.562096213228938e-05, 6.353826032916368e-05, 6.272859579521672e-05, 6.29018904503205e-05, 6.0113453361722795e-05, 3.5028168483663885e-07, 6.023790853414281e-05, 2.8927221930409144e-07, 2.486289955552982e-07, -2.439049094821873e-07, 7.23586744803015e-07, 2.843265647087974e-07, -2.943067221248818e-07, -1.3893047297828158e-07, 1.52036607637842e-06, -4.831843245690887e-07, 2.8401836255779593e-07, 5.212745134813822e-07, 2.936511341194766e-07, -3.1446729839724297e-07, -5.269124205051759e-07, -2.8657011109605934e-07]
  out "DampingRef":dbl[](array[numeric])=[-9.715986333850228, -9.804620961370007, -9.54588024004513, -9.60170254577697, -9.626577866122451, -9.596250355390074, -9.64259077334191, -9.56480159773466, -9.933044344760715, -9.898074081907883, -10.127245685285297, -9.959579456803663, -9.848592058138232, -9.901951530441108, -9.954686635119137, -9.873825966274635, -9.628016672431114, -9.641274788457812, -9.596183861736481, -9.745990404151138, -6.759509679390107, -9.70990530613811, -9.80477497778373, -9.635760465739468, -9.611901932041397, -9.720098348212819, -9.574905063910549, -9.662644756139297, -9.625530899370492, -9.7161863950413, -9.632968137097121, -9.717070191778047, -9.904979828016792, -10.226455165486932, -9.930316492463641, -9.89965485887198, -9.91120529966152, -9.932047344514872, -9.97273207049798, -9.984223443734265, -10.1583908972346, -10.147096450627346, -9.860886049573244, -10.057668682207598, -9.99551216959156, -10.158771957593824, -10.186342660520552, -10.267958865607406, -9.452630183093385, -9.996324456498492, -9.680037408319665, -9.579778857701095, -9.81684287978245, -9.517866044620602, -9.615922760586471, -9.630644605599858, -9.773895747337383, -9.41681308926318, -9.639155314294445, -9.677353515216478, -9.586375526499499, -9.689481951499685, -9.811259846011648, -9.68097020817921, -9.768456990320098, -9.87085342723118, -9.795790357825778, -9.824778889305371, -9.819922284633769, -9.819606708890507, -9.811007796967655, -9.988819749987554, -9.90262588690771, -9.878387898236747, -9.871947449182878, -9.787933799932823, -9.884143621062048, -9.919442335037001, -9.80567609259896, -9.823620086659078, -9.512905459594164, -9.747977295968886, -9.802303844625367, -9.766654619150236, -9.792739154735619, -9.865560396006549, -9.806381709194124, -9.581013198602312, -9.986074623737755, -9.90425760718588, -9.729098149024603, -9.575073088900112, -9.861360302437527, -9.821869232790796, -9.806741702120414, -9.720271477967685, -9.888241377151752, -9.933992331967696, -10.03927940832697, 0.14407521411619148, -9.954842346968906, -10.002121454625962, -10.031904973595093, -10.071497727407145, -9.871963127356873, -9.926048534815983, -10.005123897360653, -9.989965813901058, -10.04144009401973, -9.973634658414786, -9.972217708609776, -0.5310057319448518, -10.008220360435047, -0.017021375659971562, 0.21017647963836042, 0.4071453428214994, -0.8393246724893615, 0.40768462336107564, -0.33375657807565773, -0.6945284591593672, -0.3690780149016432, 0.7771858472497803, 0.1857421941408096, -0.07975159462366016, 0.4921816211993282, -0.23036123110343212, 0.179801318904817, -0.4810505364746216]
  in  "Tab Control 6":T18(tab)
  out "RefStatus 65-96":bool[](array[boolean])
  out "RefStatus 33-64":bool[](array[boolean])
  out "RefStatus 1-32":bool[](array[boolean])
  out "RefStatus 97-128":bool[](array[boolean])=[FALSE, FALSE, FALSE, TRUE, FALSE, FALSE, FALSE, FALSE, FALSE, FALSE, FALSE, FALSE, FALSE, FALSE, FALSE, TRUE, FALSE, TRUE, TRUE, TRUE, TRUE, TRUE, TRUE, TRUE, TRUE, TRUE, TRUE, TRUE, TRUE, TRUE, TRUE, TRUE]
  out "MessStatus 1-32":bool[](array[boolean])
  out "MessStatus 33-64":bool[](array[boolean])=[TRUE, FALSE, FALSE, FALSE, FALSE, FALSE, FALSE, FALSE, FALSE, FALSE, FALSE, FALSE, FALSE, FALSE, FALSE, FALSE, FALSE, FALSE, FALSE, FALSE, FALSE, FALSE, FALSE, FALSE, FALSE, FALSE, FALSE, FALSE, FALSE, FALSE, FALSE, FALSE]
  out "MessStatus 97-128":bool[](array[boolean])=[FALSE, FALSE, FALSE, TRUE, FALSE, FALSE, FALSE, FALSE, FALSE, FALSE, FALSE, FALSE, FALSE, FALSE, FALSE, TRUE, FALSE, TRUE, TRUE, TRUE, TRUE, TRUE, TRUE, TRUE, TRUE, TRUE, TRUE, TRUE, TRUE, TRUE, TRUE, TRUE]
  out "MessStatus 65-96":bool[](array[boolean])
  out "RT_P_rad status":bool
  out "CalibMeasFoilFit status":bool
  out "ChannelSelection status":bool
  out "SingleChannelFeedback status":bool
  out "QSBParms status":bool
  out "BoloSignal status":bool
  out "MRes status":bool
  out "CalibMeasFoilCurrent status":bool
  out "CalibRefFoilCurrent status":bool
  out "RKappa Status":bool
  out "MTau status":bool
  out "MKappa Status":bool
  out "RRes Status":bool
  out "RTau Status":bool
  out "Offset Status":bool
  out "BoloCalibRefFoilFit Satus":bool
  out "error out":errorcluster
  out "error out calibration":errorcluster
  out "AO output loop timing":dbl
  out "voltage out state":string
  out "SCVO current val":dbl
  out "RTPVO current val":dbl
  out "AO error":errorcluster
  out "voltage errorsource":string
  out "AO loop counter":i32
  in  "Tab Control 8":enum32{"A", "B", "C", "D"}(tab)
  out "BoloSignalErrorOut":errorcluster
  out "parms error out":errorcluster
  out "CalibMeasFoilFit 2":errorcluster
  out "BoloCalibRefFoilFitErrorOut":errorcluster
  out "MKappaErrorOut":errorcluster
  out "RResErrorOut":errorcluster
  out "MResErrorOut":errorcluster
  out "RKappaErrorOut":errorcluster
  out "SingleChannelFeedbackErrorOut":errorcluster
  out "RT_P_rad ErrorOut":errorcluster
  out "ChannelSelection ErrorOut":errorcluster
  out "OffsetErrorOut":errorcluster
  out "CalibMeasFoilCurrentErrorOut":errorcluster
  out "RTauErrorOut":errorcluster
  out "MTauErrorOut":errorcluster
  out "CalibRefFoilCurrentErrorOut":errorcluster
  out "voltage status":bool
  out "FilterTimeOut":bool
  out "Fehler READ U+P":bool
  out "Fehler":bool
  out "Timed Out":bool
  out "voltage output on":bool=TRUE
  out "voltage out loop status":bool
  out "MeasFoilStatus":bool
  out "RefFoilStatus":bool
  in  "stop":bool
  out "Acquired Samples:":u32(slide) scale=-1.0..3125.0
  out "state":string="Wait for Start"
  # "WENDELSTEIN - 7-X Bolometer DAQ System                 v2013"
  # "2021 @ pih"
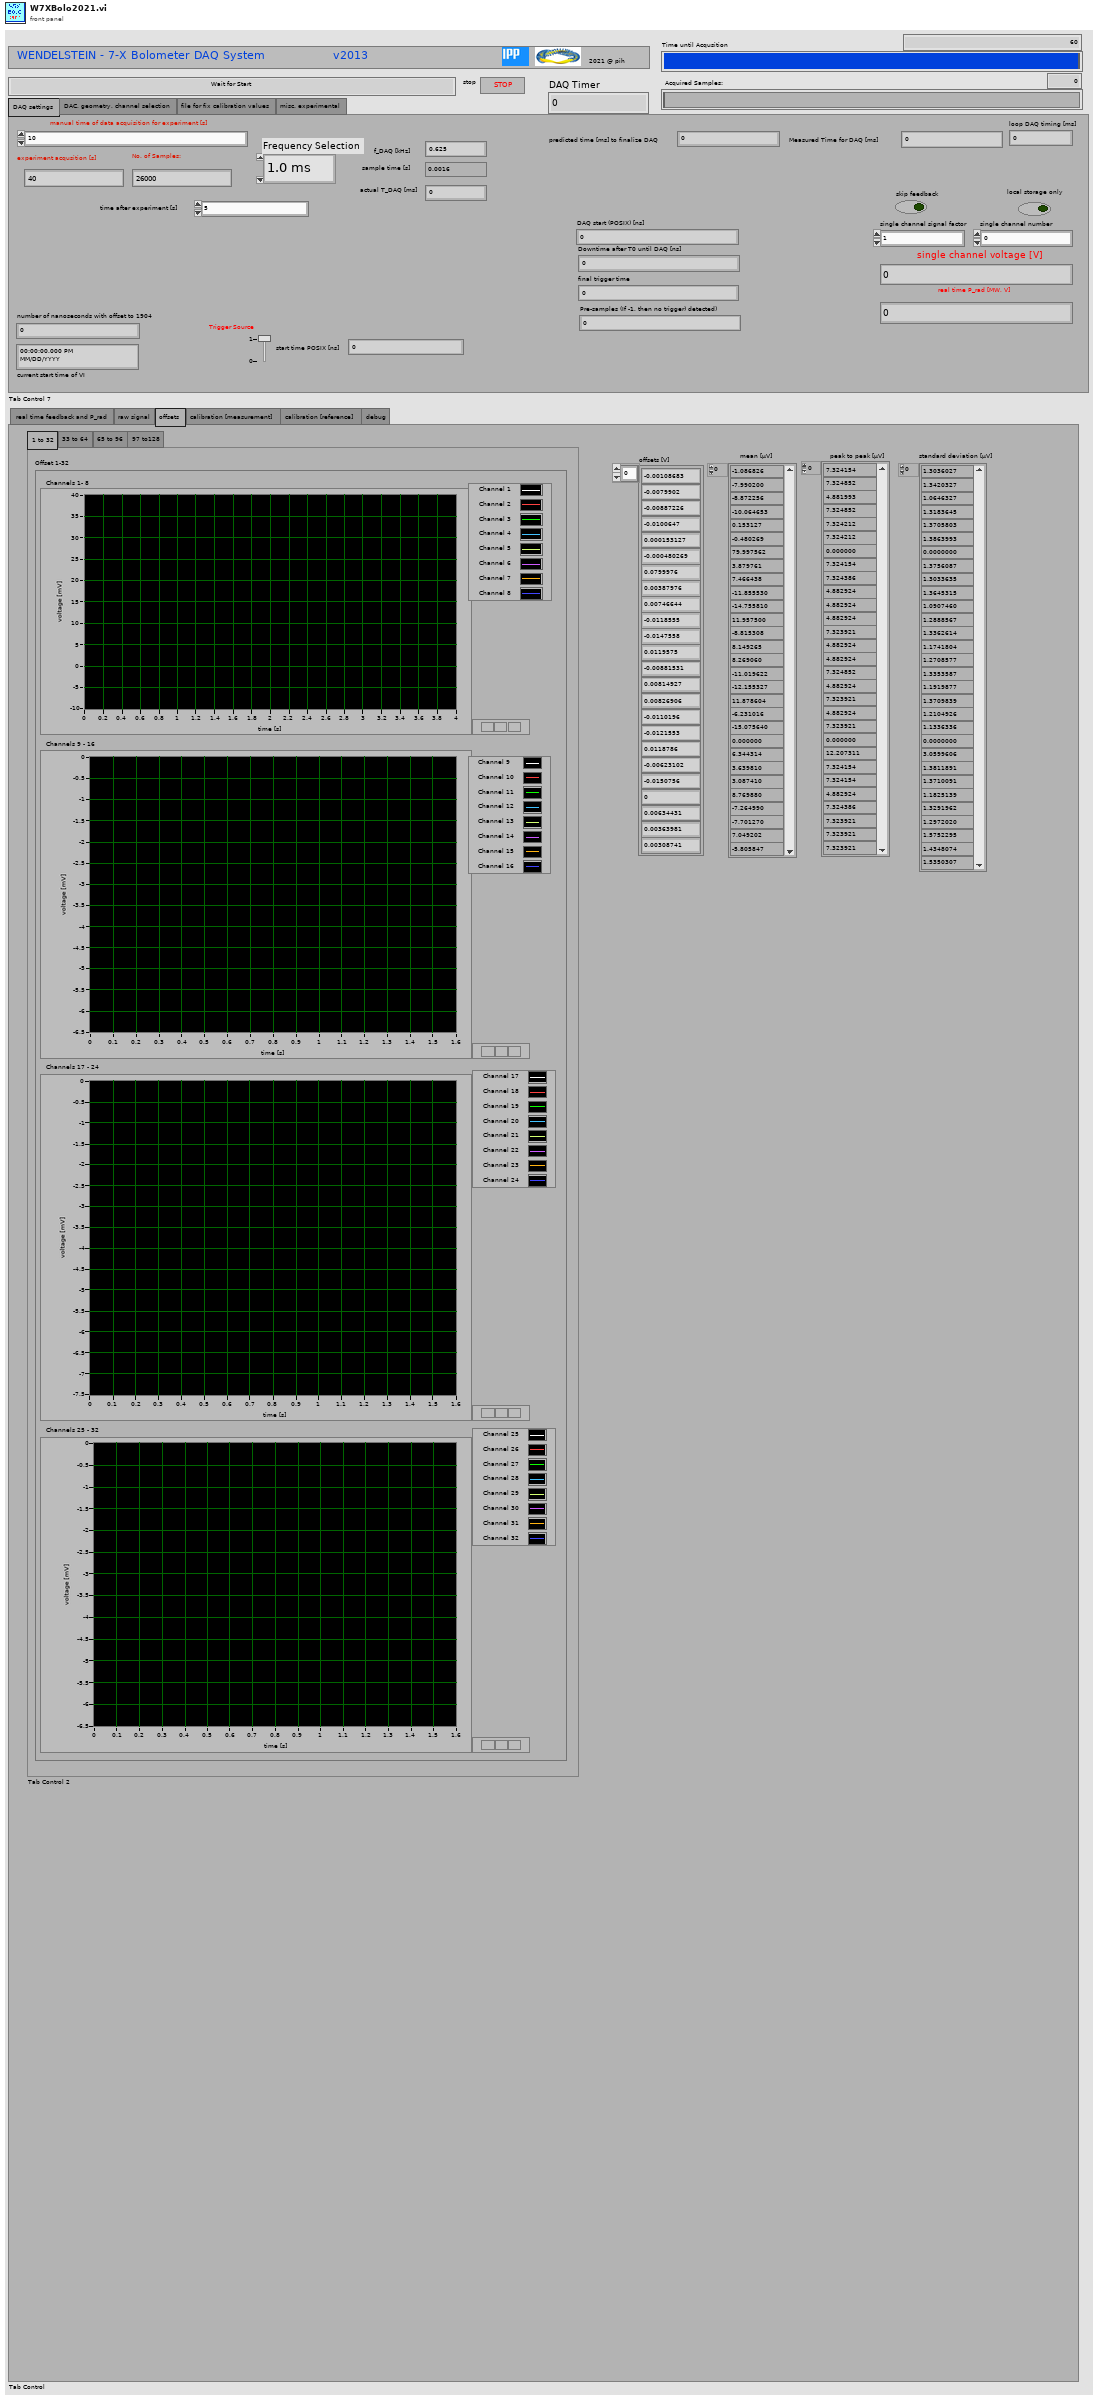
[diagram p1: front panel]
types:
  T1 = enum32{"DAQ settings", "DAC, geometry, channel selection", "file for fix calibration values", "misc. experimental"}
  T2 = typedef "W7XBolo_2021.ctl" = dbl
  T3 = enum32{"real time feedback and P_rad ", "raw signal", "offsets", "calibration [measurement]", "calibration [reference]", "debug"}
  T4 = cluster{"Channels 33 - 40":cluster{"tstart":dbl, "FPGSampleTime":dbl, dbl[][]}, "Channels 41 - 48":cluster{"tstart":dbl, "FPGSampleTime":dbl, dbl[][]}, "Channels 49 - 56":cluster{"tstart":dbl, "FPGSampleTime":dbl, dbl[][]}, "Channels 57 - 64":cluster{"tstart":dbl, "FPGSampleTime":dbl, dbl[][]}}
  T5 = cluster{"Channels 1- 8":cluster{"tstart":dbl, "FPGSampleTime":dbl, dbl[][]}, "Channels 9 - 16":cluster{"tstart":dbl, "FPGSampleTime":dbl, dbl[][]}, "Channels 17 - 24":cluster{"tstart":dbl, "FPGSampleTime":dbl, dbl[][]}, "Channels 25 - 32":cluster{"tstart":dbl, "FPGSampleTime":dbl, dbl[][]}}
  T6 = cluster{"Channels 97 - 104":cluster{"tstart":dbl, "FPGSampleTime":dbl, dbl[][]}, "Channels 105 - 112":cluster{"tstart":dbl, "FPGSampleTime":dbl, dbl[][]}, "Channels 113 - 120":cluster{"tstart":dbl, "FPGSampleTime":dbl, dbl[][]}, "Channels 121 - 128":cluster{"tstart":dbl, "FPGSampleTime":dbl, dbl[][]}}
  T7 = cluster{"Channels 65 - 71":cluster{"tstart":dbl, "FPGSampleTime":dbl, dbl[][]}, "Channels 73 - 80":cluster{"tstart":dbl, "FPGSampleTime":dbl, dbl[][]}, "Channels 81 - 88":cluster{"tstart":dbl, "FPGSampleTime":dbl, dbl[][]}, "Channels 89- 96":cluster{"tstart":dbl, "FPGSampleTime":dbl, dbl[][]}}
  T8 = enum32{"1 to 32", "33 to 64", "65 to 96", "97 to128"}
  T9 = enum32{"1 to 32", "33 to 64", "65 to 96", "97 to 128"}
  T10 = cluster{"Channels 17 - 20":cluster{"tstart":sgl, "dt":sgl, "OutArray":dbl[][]}, "Channels 21 - 24":cluster{"tstart":sgl, "dt":sgl, "OutArray":dbl[][]}, "Channels 25 - 28":cluster{"tstart":sgl, "dt":sgl, "OutArray":dbl[][]}, "Channels 29 - 32":cluster{"tstart":sgl, "dt":sgl, "OutArray":dbl[][]}}
  T11 = cluster{"Channels 1- 4":cluster{"tstart":sgl, "dt":sgl, "OutArray":dbl[][]}, "Channels 5 - 8":cluster{"tstart":sgl, "dt":sgl, "OutArray":dbl[][]}, "Channels 9 - 12":cluster{"tstart":sgl, "dt":sgl, "OutArray":dbl[][]}, "Channels 13 - 16":cluster{"tstart":sgl, "dt":sgl, "OutArray":dbl[][]}}
  T12 = cluster{"Channels 49 - 52":cluster{"tstart":sgl, "dt":sgl, "OutArray":dbl[][]}, "Channels 53 - 56":cluster{"tstart":sgl, "dt":sgl, "OutArray":dbl[][]}, "Channels 57 - 60":cluster{"tstart":sgl, "dt":sgl, "OutArray":dbl[][]}, "Channels 61 - 64":cluster{"tstart":sgl, "dt":sgl, "OutArray":dbl[][]}}
  T13 = cluster{"Channels 33 - 36":cluster{"tstart":sgl, "dt":sgl, "OutArray":dbl[][]}, "Channels 37 - 40":cluster{"tstart":sgl, "dt":sgl, "OutArray":dbl[][]}, "Channels 41 - 44":cluster{"tstart":sgl, "dt":sgl, "OutArray":dbl[][]}, "Channels 45 - 48":cluster{"tstart":sgl, "dt":sgl, "OutArray":dbl[][]}}
  T14 = cluster{"Channels 81 - 84":cluster{"tstart":sgl, "dt":sgl, "OutArray":dbl[][]}, "Channels 85 - 88":cluster{"tstart":sgl, "dt":sgl, "OutArray":dbl[][]}, "Channels 89 - 92":cluster{"tstart":sgl, "dt":sgl, "OutArray":dbl[][]}, "Channels 93 - 96":cluster{"tstart":sgl, "dt":sgl, "OutArray":dbl[][]}}
  T15 = cluster{"Channels 65 - 68":cluster{"tstart":sgl, "dt":sgl, "OutArray":dbl[][]}, "Channels 69 - 72":cluster{"tstart":sgl, "dt":sgl, "OutArray":dbl[][]}, "Channels 73 - 76":cluster{"tstart":sgl, "dt":sgl, "OutArray":dbl[][]}, "Channels 77 - 80":cluster{"tstart":sgl, "dt":sgl, "OutArray":dbl[][]}}
  T16 = cluster{"Channels 113 - 116":cluster{"tstart":sgl, "dt":sgl, "OutArray":dbl[][]}, "Channels 117 - 120":cluster{"tstart":sgl, "dt":sgl, "OutArray":dbl[][]}, "Channels 121 - 124":cluster{"tstart":sgl, "dt":sgl, "OutArray":dbl[][]}, "Channels 125 - 128":cluster{"tstart":sgl, "dt":sgl, "OutArray":dbl[][]}}
  T17 = cluster{"Channels 97 - 100":cluster{"tstart":sgl, "dt":sgl, "OutArray":dbl[][]}, "Channels 101 - 104":cluster{"tstart":sgl, "dt":sgl, "OutArray":dbl[][]}, "Channels 104 - 108":cluster{"tstart":sgl, "dt":sgl, "OutArray":dbl[][]}, "Channels 109 - 112":cluster{"tstart":sgl, "dt":sgl, "OutArray":dbl[][]}}
  T18 = enum32{"detector status", "local file storage status", "device reference and calibration status", "signal output", "archive output"}
  T19 = cluster{"tstart":sgl, "dt":sgl, "OutArray":dbl[][]}
  T20 = cluster{"Channels 9 - 12":cluster{"tstart":sgl, "dt":sgl, "OutArray":dbl[][]}, "Channels 9 - 12":cluster{"tstart":sgl, "dt":sgl, "OutArray":dbl[][]}, "Channels 9 - 12":cluster{"tstart":sgl, "dt":sgl, "OutArray":dbl[][]}, "Channels 9 - 12":cluster{"tstart":sgl, "dt":sgl, "OutArray":dbl[][]}}
  T21 = typedef "nirio_resource_hc.ctl" = tag
  T22 = typedef "XDNodeRunTimeDep.lvlib/timing_clust.ctl" = cluster{"Expected End [f-1]":u64, "Actual End [f-1]":u64, "Finished Late? [f-1]":bool, "Expected End [i-1]":u64, "Actual End [i-1]":u64, "Finished Late? [i-1]":bool, "Expected Start [i]":u64, "Actual Start [i]":u64, "Expected Start [f]":u64, "Actual Start [f]":u64, "Source Name":string, "Structure Name":string, "Period":i64, "Deadline":i64, "Offset":i64, "Start":i64, "Priority":i32, "Timeout":i32, "Mode":T23, "Wakeup Reason":T24, "Error":errorcluster, "Source Type":string, "Secondary Source Type":string, "Global End Time":u64, "Global Start Time":u64, "Frame Duration":u64, "Iteration Duration":u64, "Assigned CPU":i32, "I/O Scan Engine Mode":u32}
  T23 = typedef "XDNodeRunTimeDep.lvlib/nitl_modes.ctl" = enum32{"No Change", "Process missed periods, maintain original phase", "Discard missed periods, maintain original phase", "Process missed periods, ignore original phase", "Discard missed periods, ignore original phase"}
  T24 = typedef "XDNodeRunTimeDep.lvlib/wakeup.ctl" = enum32{"Normal", "Aborted", "Asynchronous wakeup", "Timing source error", "Timed loop error", "Timeout"}
  T25 = cluster{"Channels 33 - 40":cluster{"tstart":dbl, "FPGSampleTime":dbl, dbl[][]}, "Channels 41 - 48":cluster{"tstart":dbl, "FPGSampleTime":dbl, dbl[][]}, "Channels 49 - 56":cluster{"tstart":dbl, "FPGSampleTime":dbl, dbl[][]}, "Channels 57 - 58":cluster{"tstart":dbl, "FPGSampleTime":dbl, dbl[][]}}
  T26 = cluster{"real time P_rad [MW, V]":refnum<vi>, "real time P_rad array":refnum<vi>, "single channel voltage [V]":refnum<vi>, "single channel voltage array":refnum<vi>}
  T27 = cluster{"Array":dbl[], sgl[], "Array 2":dbl[], "all rows":dbl[], "F_ch":dbl[], "tau_fact":dbl[], "all rows":dbl[][], dbl, sgl[], "single channel signal factor":dbl, "set sample time [s]":sgl, dbl[], "ArrayOutput":dbl[], "all rows":i64[][], i32, "single channel number":i64}
  T28 = cluster{"Channels 1- 8":cluster{"tstart":sgl, "dt":sgl, "OutArray":dbl[][]}, "Channels 9 - 16":cluster{"tstart":sgl, "dt":sgl, "OutArray":dbl[][]}, "Channels 17 - 24":cluster{"tstart":sgl, "dt":sgl, "OutArray":dbl[][]}, "Channels 25 - 32":cluster{"tstart":sgl, "dt":sgl, "OutArray":dbl[][]}}
  T29 = cluster{"Channels 33 - 40":cluster{"tstart":sgl, "dt":sgl, "OutArray":dbl[][]}, "Channels 41 - 48":cluster{"tstart":sgl, "dt":sgl, "OutArray":dbl[][]}, "Channels 49 - 56":cluster{"tstart":sgl, "dt":sgl, "OutArray":dbl[][]}, "Channels 57 - 58":cluster{"tstart":sgl, "dt":sgl, "OutArray":dbl[][]}}
  T30 = cluster{"sample_period":dbl, "sample_rate":dbl, "pulse_length":dbl, "detector":string, "NChannels":i16, "ADCBits":i16, "BridgeVoltage (V)":sgl, "DAC Range Setting":u8, "AD 7730 Bit Settings":i32, "DAC and AD Settings":i32, "chanDescs":cluster{"name":string, "active":i32, "physicalQuantity":cluster{"type":string}}[], "start time":i64, "Pre-start time (ms) of DAQ Typically set to 1000 ms":i32, "Measured Time for DAQ [ms] ":u32, "single channel number":i64, "maximum voltage @ 10MW single channel":dbl, "ExptSampleFrequency (Hz)":sgl, "single channel voltage factor":dbl, "CalibSampleFrequency (Hz)":sgl, "predicted time [ms] to finalize DAQ":dbl, "CalStep1 (V)":string, "CalStep2 (V)":string, "data string":string, "loop DAQ timing [ms]":dbl}[]
  T31 = typedef "LabVIEWHTTPClient.lvlib/ClientHandle.ctl" = refnum<k1>
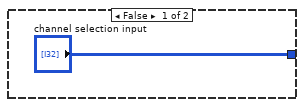
[diagram p2: hidden frame]
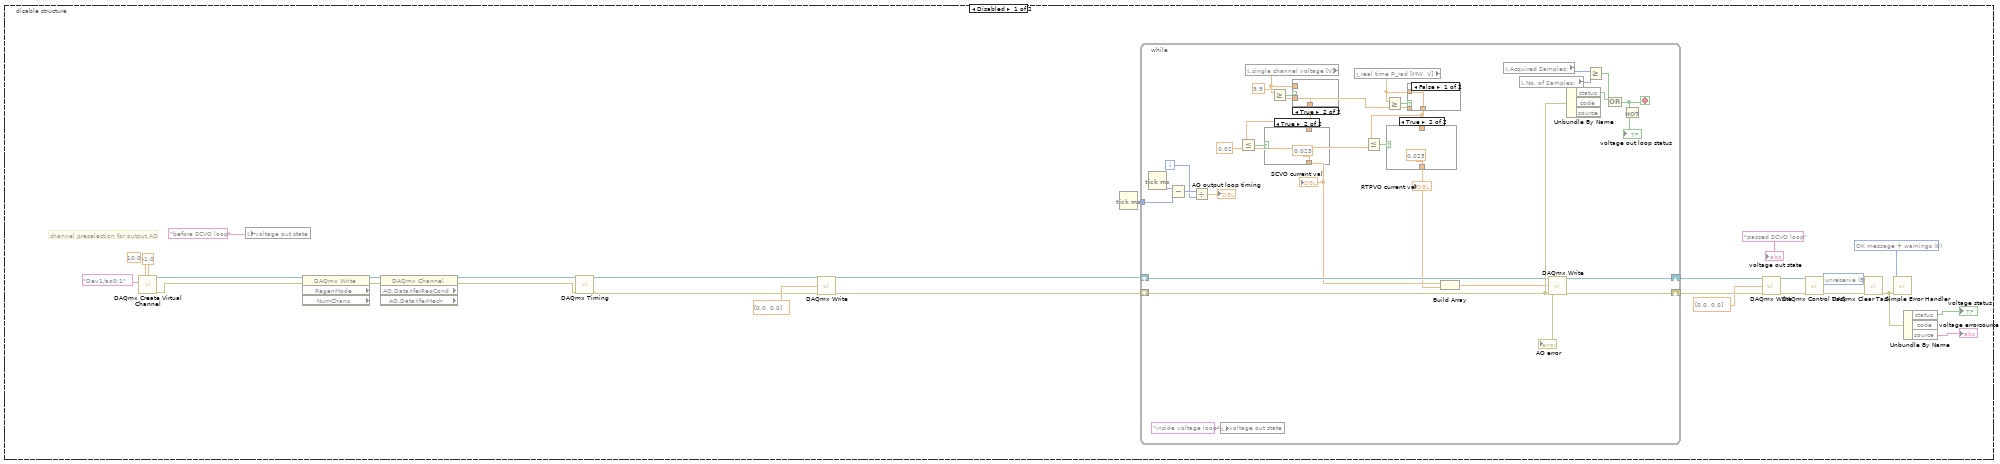
[diagram p6: hidden frame]
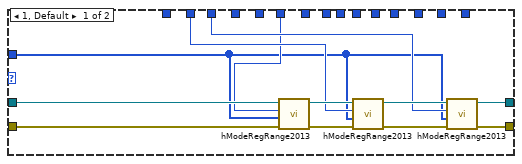
[diagram p16: hidden frame]
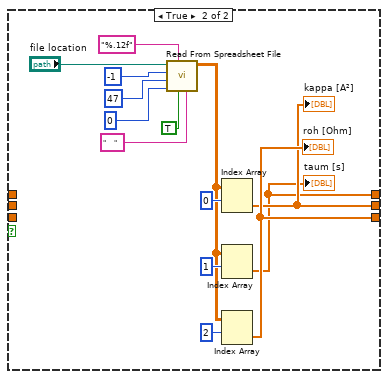
[diagram p17: hidden frame]
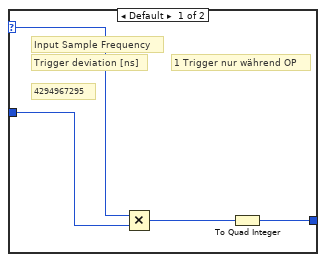
[diagram p19: hidden frame]
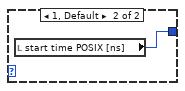
[diagram p20: hidden frame]
diagram:
  w161 = i64 -1000000000  # Ns per Sec
  # "#Timing \n\nAC measurements\n2.5 kHz\nwith SKIP=1 \n\n= 5MHz/16/(3*37+14)"
  # "#Timing \n\nAC measurements\n1.25 kHz\nwith SKIP=0 \n\n= 5MHz/16/250"
  # "#Timing \n\nAC measurements\n2.083 kHz\nwith SKIP=1 \n\n= 5MHz/16/(3*45+15)"
  # "back to synch state"
  # "A (IFS at 80mV) ++ 8 (IZS at input range) ++ C (SZS at input range) ++ 2 (CCM)"
  # "xEXXX (1110)    1 1 1        System Full-Scale Calibration\n====================================================================\nFull-Scale System Calibration Mode. This activates full-scale system calibration on the selected input\nchannel. Calibration is performed at the selected gain on the input voltage provided at the analog input\nduring this calibration sequence. This input voltage should remain stable for the duration of the calibra-\ntion. When this full-scale system calibration is complete, the part updates the contents of the appropriate\nGain Calibration Register and returns to Sync Mode with MD2, MD1 and MD0 returning to 0, 0, 0.\nThe RDY output and bit go high when calibration is initiated and return low when this full-scale calibra-\ntion is complete to indicate that the part is back in Sync Mode and ready for further operations.\n\nCalibration on externally-applied input voltage with PGA set for selected input range. The input applied is assumed\nto be the full-scale of the system. If ac = 1, the system continues to use ac excitation for the duration of the\ncalibration. This calibration should be preceded by a System Zero-Scale or Internal Zero-Scale calibration. The\nGain Calibration Register for the selected channel is updated at the end of this calibration sequence."
  # "xCXXX (1100)    1 1 0        System Zero-Scale Calibration\n=====================================================================\nZero-Scale System Calibration Mode. This activates zero scale system calibration on the channel selected\nby CH1 and CH0 of the Mode Register. Calibration is performed at the selected gain on the input volt-\nage provided at the analog input during this calibration sequence. This input voltage should remain\nstable for the duration of the calibration. When this zero-scale system calibration is complete, the part\nupdates the contents of the appropriate Offset Calibration Register and returns to Sync Mode with MD2,\nMD1 and MD0 returning to 0, 0, 0. The RDY output and bit go high when calibration is initiated and\nreturn low when this zero-scale calibration is complete to indicate that the part is back in Sync Mode and\nready for further operations.\n\nCalibration on externally applied input voltage with PGA set for selected input range. The input applied is assumed\nto be the zero scale of the system. If ac = 1, the system continues to use ac excitation for the duration of the\ncalibration. For full system calibration, this System Zero-Scale calibration should be performed first. For applications\nwhich require a System Zero-Scale and Internal Full-Scale calibration, this calibration should be preceded by the\nInternal Full-Scale calibration. The Offset Calibration Register for the selected channel is updated at the end of\nthis calibration sequence."
  # "xAXXX (1010)    1 0 1        Internal Full-Scale Calibration\n=====================================================================\nFull-Scale Self-Calibration Mode. This activates full-scale self-calibration on the channel selected by\nCH1 and CH0 of the Mode Register. This full-scale self-calibration is performed at the selected gain on\nan internally-generated full-scale signal. When this full-scale self-calibration is complete, the part updates\nthe contents of the appropriate Gain Calibration Register and Offset Calibration Register and returns to\nSync Mode with MD2, MD1 and MD0 returning to 0, 0, 0. The RDY output and bit go high when\ncalibration is initiated and return low when this full-scale self-calibration is complete to indicate that the\npart is back in Sync Mode and ready for further operations\n\nCalibration on internally-generated input full-scale with PGA set for selected input range. The ac bit is ignored for\nthis calibration sequence. The sequence is performed with dc excitation. The Gain Calibration Register for the\nselected channel is updated at the end of this calibration sequence. It is recommended that internal full-scale\ncalibrations are performed on the 80 mV range, regardless of the subsequent operating range, to optimize the post-\ncalibration gain error. This calibration should be followed by either an Internal Zero-Scale or System Zero-Scale\ncalibration. This zero-scale calibration should be performed at the operating input range."
  # "x8XXX (1000)    1 0 0       Internal Zero-Scale Calibration\n========================================================================\nZero-Scale Self-Calibration Mode. This activates zero-scale self-calibration on the channel selected by\nCH1 and CH0 of the Mode Register. This zero-scale self-calibration is performed at the selected gain on\ninternally shorted (zeroed) inputs. When this zero-scale self-calibration is complete, the part updates the\ncontents of the appropriate Offset Calibration Register and returns to Sync Mode with MD2, MD1 and\nMD0 returning to 0, 0, 0. The RDY output and bit go high when calibration is initiated and return low\nwhen this zero-scale self-calibration is complete to indicate that the part is back in Sync Mode and ready\nfor further operations.\n\nCalibration on internal shorted input with PGA set for selected input range. The ac bit is ignored for this calibra-\ntion sequence. The sequence is performed with dc excitation. The Offset Calibration Register for the selected channel is\nupdated at the end of this calibration sequence. For full selfcalibration, this calibration should be preceded by an Internal\nFull-Scale calibration. For applications which require an Internal Zero-Scale and System Full-Scale calibration, this\nInternal Zero-Scale calibration should be performed first."
  # "x6XXX (0110)    0 1 1        Power-Down (Standby) Mode\n============================================================\nPower-Down (Standby) Mode. In this mode, the AD7730 goes into its power-down or standby state.\nPlacing the part in this mode is equivalent to exerting the STANDBY input pin. However, exerting\nSTANDBY does not actually force these mode bits to 0, 1, 1."
  # "x4XXX (0100)    0 1 0        Single Conversion Mode\n===============================================================\nSingle Conversion Mode. In this mode, the AD7730 performs a single conversion, updates the Data\nRegister, returns to the Sync Mode and resets the mode bits to 0, 0, 0. The result of the single conversion\non the AD7730 in this mode will not be provided until the full settling time of the filter has elapsed."
  # "x2XXX (0010)    0 0 1        Continuous Conversion Mode\n==============================================================\nContinuous Conversion Mode. In this mode, the AD7730 is continuously processing data and providing\nconversion results to the Data Register at the programmed output update rate (as determined by the\nFilter Register). For most applications, this would be the normal operating mode of the AD7730"
  # "x0XXX (0000)    0 0 0        Sync (Idle) Mode Power-On/Reset Default\n=============================================================\nSync (Idle) Mode. In this mode, the modulator and filter are held in reset mode and the AD7730 is not\nprocessing any new samples or data. Placing the part in this mode is equivalent to exerting the SYNC\ninput pin. However, exerting the SYNC pin does not actually force these mode bits to 0, 0, 0. The part\nreturns to this mode after a calibration or after a conversion in Single Conversion Mode. This is the\ndefault condition of these bits after Power-On/Reset."
  # "HEX (BIN)          BINARY    STATUS\n=========================================\nx8XXX (1000)    1 0 0        Internal Zero-Scale Calibration\n\nx9XXX (1001)    1 0 0        Internal Zero-Scale Calibration\n\nxAXXX (1010)    1 0 1        Internal Full-Scale Calibration\n\nxBXXX (1011)    1 0 1        Internal Full-Scale Calibration\n\nxCXXX (1100)    1 1 0        System Zero-Scale Calibration\n\nxDXXX (1101)    1 1 0        System Zero-Scale Calibration\n\nxEXXX (1110)    1 1 1       System Full-Scale Calibration\n\nxFXXX (1111)    1 1 1        System Full-Scale Calibration\n\nx0XXX (0000)    0 0 0       Sync (Idle) Mode Power-On/Reset Default\n\nx1XXX (0001)    0 0 0       Sync (Idle) Mode Power-On/Reset Default\n\nx2XXX (0010)    0 0 1       Continuous Conversion Mode\n\nx3XXX (0011)    0 0 1       Continuous Conversion Mode\n\nx4XXX (0100)    0 1 0       Single Conversion Mode\n\nx5XXX (0101)    0 1 0       Single Conversion Mode\n\nx6XXX (0110)    0 1 1       Power-Down (Standby) Mode\n\nx7XXX (0111)    0 1 1       Power-Down (Standby) Mode"
  # "Negative Sample Time [ns]"
  # "Index von dem Sample\nals der Trigger empfangen wurde"
  # "T1 Trigger\nkommt hier"
  # "A=> Internal full scale calibration\n8=> Internal zero scale calibration\nC=> System Zero scale Calibration\n2=> Continuous conversion\n\n5V reference\n80 mV scale\nChannel 1 input (voltage at bridge)\nMaster clock disable\n\np.15 7730 manual"
  # "AC 1.25 kHz Frequenz\nSKIP=0"
  n1 = call <vilib>:"High Resolution Relative Seconds.vi"() -> ("relative seconds"=w166:dbl)
  n2 = flat-sequence {
    tunnel: [w227] -> w167
    tunnel: ["FPGA VI Reference In"] -> w187
    tunnel: [w228] -> w185
    tunnel: w167 -> [w228]
    frame #0 {
      n3 = Tick Count (ms)() -> (millisecond timer value=w227:u32)
    }
    frame #1 {
      n4 = case shown="True" "Clear all Values \nfrom Beginning" {
        frame False {
        }
        frame True {
          n5 = flat-sequence {
            frame #0 {
              w233 = bool[] [] ("MessStatus 1-32")
              w231 = dbl[] [] ("Kappa00")
              w232 = T19 {"tstart"=0.0, "dt"=0.0, "OutArray"=[]} ("Channels 9 - 12")
              # "Clear Graphs"
              n6 = local write "rohR [Ohm]"(w231) -> ()
              n7 = local write "rohM [Ohm]"(w231) -> ()
              n8 = local write "kappaM [A²]"(w231) -> ()
              n9 = local write "kappaR [A²]"(w231) -> ()
              n10 = local write "roh [Ohm]"(w231) -> ()
              n11 = local write "taum [s]"(w231) -> ()
              n12 = local write "kappa [A²]"(w231) -> ()
              n13 = local write "tauR [s]"(w231) -> ()
              n14 = local write "MessStatus 1-32"(w233) -> ()
              n15 = local write "MessStatus 65-96"(w233) -> ()
              n16 = local write "MessStatus 97-128"(w233) -> ()
              n17 = local write "MessStatus 33-64"(w233) -> ()
              n18 = local write "TauM"(w231) -> ()
              n19 = local write "RefStatus 97-128"(w233) -> ()
              n20 = local write "RefStatus 1-32"(w233) -> ()
              n21 = local write "RefStatus 33-64"(w233) -> ()
              n22 = local write "RefStatus 65-96"(w233) -> ()
              n23 = Bundle("Channels 9 - 12"=w232, "Channels 9 - 12"=w232, "Channels 9 - 12"=w232, "Channels 9 - 12"=w232) -> (w234:T20)  [unwired: 1 in]
              n24 = local write "Raw 1-32"(w234) -> ()
              n25 = local write "Raw 33-64"(w234) -> ()
              n26 = local write "standard deviation [µV]"(w231) -> ()
              n27 = local write "peak to peak [µV]"(w231) -> ()
              n28 = local write "mean [µV]"(w231) -> ()
              n29 = local write "MessCal 1-16"(w234) -> ()
              n30 = local write "MessCal 113 - 128"(w234) -> ()
              n31 = local write "MessCal 17-32"(w234) -> ()
              n32 = local write "MessCal 33 - 49"(w234) -> ()
              n33 = local write "MessCal 49 - 64"(w234) -> ()
              n34 = local write "MessCal 65 - 80"(w234) -> ()
              n35 = local write "MessCal 81 - 96"(w234) -> ()
              n36 = local write "MessCal 97 - 112"(w234) -> ()
              n37 = local write "RefCal 1-16"(w234) -> ()
              n38 = local write "RefCal 113 - 128"(w234) -> ()
              n39 = local write "RefCal 17-32"(w234) -> ()
              n40 = local write "RefCal 33 - 48"(w234) -> ()
              n41 = local write "RefCal 49 - 64"(w234) -> ()
              n42 = local write "RefCal 65 - 80"(w234) -> ()
              n43 = local write "RefCal 81 - 96"(w234) -> ()
              n44 = local write "RefCal 97 - 112"(w234) -> ()
              n45 = local write "Raw 65 - 97"(w234) -> ()
              n46 = local write "Raw 97 - 128"(w234) -> ()
              n47 = local write "Offset 1-32"(w234) -> ()
              n48 = local write "Offset 33-64"(w234) -> ()
              n49 = local write "Offset 65 - 96"(w234) -> ()
              n50 = local write "Offset 97 - 128"(w234) -> ()
            }
          }
        }
      }
    }
  }
  n51 = while {
    tunnel: w166 -> [w244]
    i -> [w237]
    stop <- w246 stop-if-true
    n52 = local read "time between VI start and points of interest [s]"() -> (w240:dbl)
    n53 = local read "time before experiment [s]"() -> (w239:T2)
    n54 = Subtract(x=w240, y=w239) -> (x-y=w238:T2)
    n55 = call <vilib>:"High Resolution Relative Seconds.vi"() -> ("relative seconds"=w242:dbl)
    n56 = Add(x=w244, y=w238) -> (x+y=w243:T2)
    n57 = Subtract(x=w243, y=w242) -> (x-y=→"Time until Acqusition":T2)
    n58 = Get Date/Time In Seconds() -> (seconds since 1Jan1904=w252:timestamp)
    "current start time of VI" <- w252
    n59 = To Quad Integer(1:w252) -> (0:w254:i64)
    n60 = Subtract(x=w254, y=2082844800) -> (x-y=w250:i64)
    n61 = Multiply(x=1000000000, y=w250) -> (x*y=w245:i64)
    "number of nanoseconds with offset to 1904" <- w245
    n62 = Wait Until Next ms Multiple(millisecond multiple=1) -> ()  [unwired: 1 out]
    n63 = local read "state"() -> (w247:string)
    n64 = Equal?(x="Acquiring Data...", y=w247) -> (x = y?=w246:bool)
    n65 = Equal?(x=0, y=w237) -> (x = y?=w236:bool)
    n66 = case shown="True" w236 {
      tunnel: w245 -> [_ w255]
      frame False {
      }
      frame True {
        n67 = local write "start time POSIX [ns]"(w255) -> ()
        "start time POSIX [ns]" <- w255
      }
    }
  }
  n68 = Not A Number/Path/Refnum?(number/path/refnum=w187) -> (NaN/Path/Refnum?=w186:bool)
  n69 = case shown="True" w186 {
    tunnel: [w256 w258] -> w190
    tunnel: [_ w257] -> w189
    tunnel: w187 -> [w256 _]
    frame False {
    }
    frame True {
      n70 = xnode "Open FPGA VI Reference"("resource name"=T21 "RIO0") -> ("FPGA VI Reference Out"=w258:refnum<k20>, "error out"=w257:errorcluster)  [unwired: 1 in]
    }
  }
  "error out" <- w189
  n71 = case shown="True" "Read Channel Selection from file" {
    tunnel: ["channel selection input" w261] -> w75
    frame False {
    }
    frame True {
      n72 = call-poly <vilib>:"Read From Spreadsheet File.vi"("delimiter (\\t)"="\t" ("delimiter (\\t)"), "format (%d)"="%d", "max characters/row  (no limit:0)"=0, "start of read offset (chars.:0)"=0, "number of rows (all:-1)"=-1, "file path (dialog if empty)"="Path to channel selection file") -> ("all rows"=w261:i64[][])  [unwired: 1 in, 4 out]
      "file import" <- w261
    }
  }
  "final channel selection" <- w75
  n73 = flat-sequence {
    tunnel: "Cancel" ("name (unnamed)") -> [w277]
    tunnel: "Transferred1" ("name (unnamed)") -> [w276]
    tunnel: u32 0 -> [w275]
    tunnel: FALSE -> [w274]
    tunnel: [w273] -> w217
    tunnel: [w272] -> w216
    tunnel: [w271] -> w215
    tunnel: [w270] -> w214
    tunnel: [u32 0] -> w188
    frame #0 {
      n74 = local write "stop"(FALSE ("stop")) -> ()
      n75 = RT FIFO Create(0:w276, 1:w275) -> (8:w270:refnum<k33>, 11:w271:errorcluster)  [unwired: 2 in, 5 out]
      n76 = RT FIFO Create(0:w277, 1:w274) -> (8:w273:refnum<k33>, 11:w272:errorcluster)  [unwired: 3 in, 4 out]
    }
  }
  n77 = xnode "Read/Write Control"("FPGA VI Reference In"=w190, "error in"=w189, "cancel"=TRUE ("clrFifo"), "Test"=FALSE) -> ("FPGA VI Reference Out"=w226:refnum<k20>, "error out"=w225:errorcluster)
  n78 = flat-sequence {
    tunnel: w226 -> [w284]
    tunnel: w225 -> [w283]
    tunnel: [w282] -> w224
    tunnel: [w281] -> w223
    frame #0 {
      n79 = xnode "Invoke Method"("FPGA VI Reference In"=w284, "error in"=w283, "IRQ Number(s)"=i32[] [0, 1, 2, 3]) -> ("FPGA VI Reference Out"=w282:refnum<k20>, "error out"=w281:errorcluster)
      n80 = Wait (ms)(milliseconds to wait=u32 100) -> ()  [unwired: 1 out]
      "state" <- "Start (100 ms)" ("state")
    }
  }
  n81 = node-c288() -> (w209:T22)  [unwired: 1 in, 4 out]
  n82 = timed-loop {
    tunnel: w217 -> [w295]
    tunnel: w216 -> [w294]
    tunnel: w215 -> [w293]
    tunnel: w214 -> [w292]
    shift-right: [w291] -> _
    shift-left: w188 -> [w285]
    tunnel: [w290] -> w211
    tunnel: [w289] -> w210
    tunnel: [w288] -> w213
    tunnel: [w287] -> w212
    timing: w209 -> [_]
    timing-out: [_] -> w208
    stop <- "stop" stop-if-true
    n83 = RT FIFO Read(0:w292, 1:w285, 3:w293) -> (8:w288:refnum<k33>, 9:w291:u32, 11:w287:errorcluster)  [unwired: 3 out]
    n84 = RT FIFO Write(0:w295, 1:"Cancel Button", 3:w294) -> (8:w290:refnum<k33>, 11:w289:errorcluster)  [unwired: 1 in, 3 out]
    "Acquired Samples:" <- w285
  }
  n85 = call-poly <vilib>:"Read From Spreadsheet File.vi"("delimiter (\\t)"="" ("delimiter (\\t)"), "format (%.3f)"="%.12f", "max characters/row  (no limit:0)"=0, "number of rows (all:-1)"=-1, "file path (dialog if empty)"="Path to kbolott and volume data file") -> ("all rows"=w73:dbl[][])  [unwired: 2 in, 4 out]
  "kbolott_and_volume" <- w73
  n86 = flat-sequence {
    tunnel: w223 -> [w300]
    tunnel: [w299] -> w205
    tunnel: w224 -> [w301]
    tunnel: [w302] -> w192
    frame #0 {
      n87 = local write "state"("Reset" ("state")) -> ()
      n88 = call "hReset2014.vi"("error in"=w300, "FPGA VI Reference In"=w301) -> ("error out"=w299:errorcluster, "FPGA VI Reference Out"=w302:refnum<k20>)  [unwired: 4 in]
    }
  }
  n89 = Array Size(array=w75) -> (size(s)=w14:i32[])
  n90 = local write "kbolott_and_volume"(w73) -> ()
  n91 = call-poly <vilib>:"Read From Spreadsheet File.vi"("format (%d)"="%d", "max characters/row  (no limit:0)"=58, "number of rows (all:-1)"=-1, "file path (dialog if empty)"="DAC settings file location") -> ("all rows"=w3:i64[][])  [unwired: 3 in, 4 out]
  n92 = local write "final channel selection"(w75) -> ()
  n93 = Index Array(array=w14, index=0) -> (element=w74:i32)
  "final channel\nselection size" <- w74
  n94 = Reshape Array(w3, 128 ("dimension size")) -> (w1:i64[])
  "input DAC settings" <- w1
  n95 = node-c288(w208) -> ()  [unwired: 1 out]
  n96 = call "hFilterReg2014.vi"("error in"=w205, "Filter Modus"=u16 61 ("t"), "Frequenz"=u8 79 ("AC 1kHz Frequenz\nSKIP=0"), "FPGA VI Reference In"=w192) -> ("error out"=w195:errorcluster, "Timed Out"=w201:bool, "FPGA VI Reference Out"=w194:refnum<k20>)  [unwired: 1 in]
  "FilterTimeOut" <- w201
  n97 = local write "input DAC settings"(w1) -> ()
  n98 = flat-sequence {
    tunnel: w213 -> [w308]
    tunnel: w212 -> [w307]
    tunnel: w211 -> [w306]
    tunnel: w210 -> [w305]
    frame #0 {
      n99 = RT FIFO Delete(0:w308, 3:w307) -> ()  [unwired: 1 in, 1 out]
      n100 = RT FIFO Delete(0:w306, 3:w305) -> ()  [unwired: 1 in, 1 out]
      n101 = local write "stop"(FALSE ("stop")) -> ()
    }
  }
  n102 = call "hModeReg2014.vi"("error in"=w195, "Mode"=u16 41144, "FPGA VI Reference In"=w194) -> ("error out"=w197:errorcluster, "Timeout"=w203:bool, "FPGA VI Reference Out"=w199:refnum<k20>)  [unwired: 2 in]
  n103 = Array Size(array=w1) -> ()  [unwired: 1 out]
  n104 = call "hModeReg2014.vi"("error in"=w197, "Mode"=u16 32952, "FPGA VI Reference In"=w199) -> ("error out"=w196:errorcluster, "Timeout"=w204:bool, "FPGA VI Reference Out"=w198:refnum<k20>)  [unwired: 2 in]
  n105 = call "hModeReg2014.vi"("error in"=w196, "Mode"=u16 8376, "FPGA VI Reference In"=w198) -> ("error out"=w168:errorcluster, "Timeout"=w202:bool, "FPGA VI Reference Out"=w169:refnum<k20>)  [unwired: 2 in]
  n106 = Compound Arithmetic op=OR(w203, w204, w202, w201) -> (w193:bool)
  n107 = case shown="False" w193 {
    tunnel: [w527 w1154] -> w183
    tunnel: [w526 w1153] -> w222
    tunnel: w169 -> [w639 w1154]
    tunnel: w168 -> [w638 w1153]
    tunnel: [w542 _] -> w129
    tunnel: [w482 _] -> w84
    tunnel: [w562 _] -> w132
    tunnel: [w558 _] -> w104
    tunnel: [w512 _] -> w108
    tunnel: [w394 _] -> w160
    tunnel: [w329 _] -> w157
    tunnel: [w327 _] -> w156
    tunnel: [w379 _] -> w158
    tunnel: [w377 _] -> w155
    tunnel: [w378 _] -> w159
    tunnel: [w330 _] -> w2
    tunnel: w185 -> [w317 _]
    tunnel: [w310 _] -> w162
    tunnel: w75 -> [w459 _]
    tunnel: w74 -> [w461 _]
    tunnel: w73 -> [w460 _]
    frame False {
      w341 = bool[] [FALSE, FALSE, FALSE, TRUE, FALSE, FALSE, FALSE, FALSE, FALSE, FALSE, FALSE, FALSE, FALSE, FALSE, FALSE, TRUE, FALSE, TRUE, TRUE, TRUE, TRUE, TRUE, TRUE, TRUE, TRUE, TRUE, TRUE, TRUE, TRUE, TRUE, TRUE, TRUE]  # RefStatus 97-128 Default
      w343 = bool[] [FALSE, FALSE, FALSE, FALSE, FALSE, FALSE, FALSE, FALSE, FALSE, FALSE, FALSE, FALSE, FALSE, FALSE, FALSE, FALSE, FALSE, FALSE, FALSE, FALSE, FALSE, FALSE, FALSE, FALSE, FALSE, FALSE, FALSE, FALSE, FALSE, FALSE, FALSE, FALSE]  # RefStatus 65-96 Default
      w345 = bool[] [FALSE, FALSE, FALSE, FALSE, FALSE, FALSE, FALSE, FALSE, FALSE, FALSE, FALSE, FALSE, FALSE, FALSE, FALSE, FALSE, FALSE, FALSE, FALSE, FALSE, FALSE, FALSE, FALSE, FALSE, FALSE, FALSE, FALSE, FALSE, FALSE, FALSE, FALSE, FALSE]  # RefStatus 33-64 Default
      w347 = bool[] [FALSE, FALSE, FALSE, FALSE, FALSE, FALSE, FALSE, FALSE, FALSE, FALSE, FALSE, FALSE, FALSE, FALSE, FALSE, FALSE, FALSE, FALSE, FALSE, FALSE, FALSE, FALSE, FALSE, FALSE, FALSE, FALSE, FALSE, FALSE, FALSE, FALSE, FALSE, FALSE]  # RefStatus 1-32 Default
      w354 = bool[] [FALSE, FALSE, FALSE, FALSE, FALSE, FALSE, FALSE, FALSE, FALSE, FALSE, FALSE, FALSE, FALSE, FALSE, FALSE, FALSE, FALSE, FALSE, FALSE, FALSE, FALSE, FALSE, FALSE, FALSE, FALSE, FALSE, FALSE, FALSE, FALSE, FALSE, FALSE, FALSE]  # MessStatus 1-32 Default
      w356 = bool[] [TRUE, FALSE, FALSE, FALSE, FALSE, FALSE, FALSE, FALSE, FALSE, FALSE, FALSE, FALSE, FALSE, FALSE, FALSE, FALSE, FALSE, FALSE, FALSE, FALSE, FALSE, FALSE, FALSE, FALSE, FALSE, FALSE, FALSE, FALSE, FALSE, FALSE, FALSE, FALSE]  # MessStatus 33-64 Default
      w358 = bool[] [FALSE, FALSE, FALSE, FALSE, FALSE, FALSE, FALSE, FALSE, FALSE, FALSE, FALSE, FALSE, FALSE, FALSE, FALSE, FALSE, FALSE, FALSE, FALSE, FALSE, FALSE, FALSE, FALSE, FALSE, FALSE, FALSE, FALSE, FALSE, FALSE, FALSE, FALSE, FALSE]  # MessStatus 65-96 Default
      w360 = bool[] [FALSE, FALSE, FALSE, TRUE, FALSE, FALSE, FALSE, FALSE, FALSE, FALSE, FALSE, FALSE, FALSE, FALSE, FALSE, TRUE, FALSE, TRUE, TRUE, TRUE, TRUE, TRUE, TRUE, TRUE, TRUE, TRUE, TRUE, TRUE, TRUE, TRUE, TRUE, TRUE]  # MessStatus 97-128 Default
      w388 = 128  # FitLength
      w398 = 128  # FitLength
      (unwired) u16 57
      w516 = 5000
      w579 = u8 125  # Frequenz
      w611 = 0.0008 ("FPGSampleTime")
      w606 = 0.0
      w522 = 40.0  # Rcable
      w634 = 10.0  # Rload
      w648 = sgl 0.0004  # dt
      w649 = sgl 0.0  # tstart
      w652 = sgl 0.0004  # dt
      w653 = sgl 0.0  # tstart
      w656 = sgl 80.0 ("Scale(mV)")
      # "7D => 2457.6 HZ => 0.0004 s"
      # "pre-allocation of the sample and signal arrays from the subroutine of measurement"
      # "F"
      # "7"
      # "E"
      # "6"
      # "D"
      # "5"
      # "C"
      # "B"
      # "4"
      # "9"
      # "A"
      # "3"
      # "2"
      # "8"
      # "1"
      # "C SZS (input range) ++ E SFS (input range) ++ A IFS (at input range) ++ 8 IZS (input range) ++ 2 CCM"
      # "back to sync state"
      # "A (IFS at 80mV) ++ 8 (IZS at input range) ++ C (SZS at input range) ++ 2 (CCM)"
      # "C (SZS at input range) ++ E (SFS at input range) ++ 8 (IZS at input range) ++ 2 (CCM)"
      # "A (IFS at 80mV) ++ 8 (IZS at input range) ++ C (SZS at input range) ++ 2 (CCM)"
      # "For full selfcalibration, the Internal Zero Scale calibration should be preceded by an Internal\nFull-Scale calibration. For applications which require an Internal Zero-Scale and System Full-Scale calibration, this\nInternal Zero-Scale calibration should be performed first."
      # "System Full-Scale calibration should be preceded by a System Zero-Scale or Internal Zero-Scale calibration. The\nGain Calibration Register for the selected channel is updated at the end of this calibration sequence."
      # "For full system calibration, this System Zero-Scale calibration should be performed first. For applications\nwhich require a System Zero-Scale and Internal Full-Scale calibration, this calibration should be preceded by the\nInternal Full-Scale calibration."
      # "Internal full-scale calibrations are performed on the 80 mV range, and should be followed by either an Internal Zero-Scale or System Zero-Scale\ncalibration. This zero-scale calibration should be performed at the operating input range."
      # "If the interal and system calibration procedures are used in the prior\nDAC range setup, do not subtract the previously measured offset.\n\nThis is ultimately different to the AD7730 acquired offset.\nFrom the manual, concerning the system zero scale calibration:\n\n[...] The input applied is assumed\nto be the zero scale of the system. If ac = 1, the system\ncontinues to use ac excitation for the duration of the\ncalibration. For full system calibration, this System Zero-\nScale calibration should be performed first. For applications\nwhich require a System Zero-Scale and Internal Full-Scale\ncalibration, this calibration should be preceded by the\nInternal Full-Scale calibration. [...]\n\nThough due to the wrong internal wiring, an absolute value\nhas to be taken off the raw signal."
      # "Offset Shift manually disabled because not need for low power discharges"
      # "Local TDMS Data Storage"
      # "Store raw data"
      # "#Offset measurement"
      # "#Range for measurements"
      # "A=> Internal full scale calibration\n8=> Internal zero scale calibration\nC=> System Zero scale Calibration\n2=> Continuous conversion\n\n2.5V reference\n80 mV scale\nChannel 2 input (voltage at shunt)\nMaster clock disable\n\np.15 7730 manual"
      n108 = flat-sequence {
        tunnel: [w863] -> w525
        tunnel: [w862] -> w524
        tunnel: w639 -> [w866]
        tunnel: w638 -> [w865]
        tunnel: w516 -> [w871]
        tunnel: [w870] -> w570
        tunnel: w525 -> [w873]
        tunnel: w524 -> [w872]
        tunnel: [w869] -> w569
        tunnel: [w879] -> w705
        tunnel: [w878] -> w704
        tunnel: [w877] -> w702
        tunnel: w516 -> [w875]
        tunnel: w570 -> [w881]
        tunnel: w569 -> [w880]
        frame #0 {
          n109 = call "hComRegStart2013.vi"("error in"=w865, "FPGA VI Reference In"=w866) -> ("error out"=w862:errorcluster, "Timed Out"=→"Timed Out":bool, "FPGA VI Reference Out"=w863:refnum<k20>)  [unwired: 3 in]
          n110 = call "Wait3"("Count(mSec)"=u32 3000) -> ()  [unwired: 1 out]
        }
        frame #1 {
          n111 = call "Wait6"("Count(mSec)"=u32 3000) -> ()  [unwired: 1 out]
          n112 = local write "state"("SyncRun (3000 ms)" ("state")) -> ()
          n113 = call "hSync&StartSampling2013.vi"("error in"=w872, "#Samples"=w871, "FPGA VI Reference In"=w873) -> ("error out"=w870:errorcluster, "FPGA VI Reference Out"=w869:refnum<k20>)  [unwired: 1 in]
        }
        frame #2 {
          n114 = call "hReadChannelsRTDMA2013.vi"("FPGA VI Reference In"=w880, "Nsamples"=w875, "error in"=w881) -> ("FPGA VI Reference Out"=w879:refnum<k20>, "Fehler"=→"Fehler":bool, "RawArray"=w877:i16[][], "error out"=w878:errorcluster)  [unwired: 2 in]
          n115 = local write "state"("ReadOffset" ("state")) -> ()
        }
      }
      n116 = property on="Acquired Samples:" class="Slide (strict)"("Scale.Range:Maximum"=w516) -> ()  [unwired: 2 in, 2 out]
      n117 = call "hSoftReset2013.vi"("error in"=w704, "FPGA VI Reference In"=w705) -> ("error out"=w577:errorcluster, "FPGA VI Reference Out"=w572:refnum<k20>)  [unwired: 4 in]
      n118 = call "Int2Volt2D.vi"("IntegerArray"=w702, "Scale(mV)"=sgl 80.0) -> ("RealArray"=w520:sgl[][])
      n119 = xnode "Read/Write Control"("FPGA VI Reference In"=w572, "error in"=w577, "HIREF"=TRUE) -> ("FPGA VI Reference Out"=w575:refnum<k20>, "error out"=w574:errorcluster)
      n120 = for {
        tunnel: w520 -> [w902] mode=indexing
        tunnel: [w901] -> w603 mode=indexing
        tunnel: [w900] -> w330 mode=indexing
        tunnel: [w899] -> w604 mode=indexing
        n121 = Array Subset(array=w902, index=500, length=1000) -> (w904:sgl[])
        n122 = Array Max & Min(array=w904) -> (max value=w907:sgl, min value=w908:sgl)  [unwired: 2 out]
        n123 = Subtract(x=w907, y=w908) -> (x-y=w901:sgl)
        n124 = call <vilib>:"Std Deviation and Variance.vi"("X"=w904, "Weighting (Sample)"=enum16{"Sample", "Population"}."Population") -> ("mean"=w900:dbl, "standard deviation"=w899:dbl)  [unwired: 1 out]
      }
      "offsets [V]" <- w330
      n125 = Array Subset(array=w520, index (row)=0, length (row)=64, index (col)=0) -> (w616:sgl[][])  [unwired: 1 in]
      n126 = Array Subset(array=w520, index (row)=64, length (row)=64, index (col)=0) -> (w612:sgl[][])  [unwired: 1 in]
      n127 = call "Visualize_Signals64.vi"("FPGSampleTime"=w611, "tstart"=w606, "Signals"=w616) -> ("plot(Signals) 33-64"=→"Offset 33-64":T25, "plot(Signals) 1-32"=→"Offset 1-32":T5)  [unwired: 7 in]
      n128 = call "Visualize_Signals64.vi"("FPGSampleTime"=w611, "tstart"=w606, "Signals"=w612) -> ("plot(Signals) 33-64"=→"Offset 97 - 128":T25, "plot(Signals) 1-32"=→"Offset 65 - 96":T5)  [unwired: 7 in]
      n129 = call "hFilterReg2014.vi"("error in"=w574, "Filter Modus"=u16 512 ("t"), "Frequenz"=w579, "FPGA VI Reference In"=w575) -> ("error out"=w573:errorcluster, "FPGA VI Reference Out"=w576:refnum<k20>)  [unwired: 1 in, 1 out]
      n130 = call "hModeReg2014.vi"("error in"=w573, "Mode"=u16 41017, "FPGA VI Reference In"=w576) -> ("error out"=w583:errorcluster, "FPGA VI Reference Out"=w582:refnum<k20>)  [unwired: 2 in, 1 out]
      n131 = call "hModeReg2014.vi"("error in"=w583, "Mode"=u16 32825, "FPGA VI Reference In"=w582) -> ("error out"=w580:errorcluster, "FPGA VI Reference Out"=w581:refnum<k20>)  [unwired: 2 in, 1 out]
      n132 = call "hModeReg2014.vi"("error in"=w580, "Mode"=u16 8249, "FPGA VI Reference In"=w581) -> ("error out"=w518:errorcluster, "FPGA VI Reference Out"=w517:refnum<k20>)  [unwired: 2 in, 1 out]
      n133 = Multiply(x=w604, y=1000000.0 ("Scale")) -> (x*y=→"standard deviation [µV]":dbl[])
      n134 = Multiply(x=w603, y=1000000.0 ("Scale")) -> (x*y=→"peak to peak [µV]":dbl[])
      n135 = Multiply(x=w330, y=1000000.0 ("Scale")) -> (x*y=→"mean [µV]":dbl[])
      n136 = control-ref of="Cancel Button"() -> (w701:refnum<vi>)
      n137 = control-ref of="state"() -> (w700:refnum<vi>)
      n138 = control-ref of="Acquired Samples:"() -> (w699:refnum<vi>)
      n139 = call "hCalRT2013.vi"("FPGA VI Reference In"=w517, "cancelbutton"=w701, "state"=w700, "Acquired Samples"=w699, "error in"=w518, "Numeric"=10000) -> ("FPGA VI Reference Out"=w636:refnum<k20>, "Ref"=w655:i16[][], "Meas"=w697:i16[][], "error out"=w635:errorcluster)  [unwired: 5 in, 1 out]
      "error out calibration" <- w635
      n140 = call "FreqSel.vi"("FreqSelRing"="Frequency Selection") -> ("set sample time [s]"=w310:sgl, "actual T_DAQ [ms]"=→"actual T_DAQ [ms]":dbl, "f_DAQ [kHz]"=→"f_DAQ [kHz]":dbl, "ModeHex"=w375:u16, "FreqHex"=w376:u16)
      "sample time [s]" <- w310
      n141 = call "Int2Volt2D.vi"("IntegerArray"=w655, "Scale(mV)"=w656) -> ("RealArray"=w657:sgl[][])
      n142 = call "Int2Volt2D.vi"("IntegerArray"=w697, "Scale(mV)"=w656) -> ("RealArray"=w698:sgl[][])
      n143 = flat-sequence {
        tunnel: w636 -> [w892]
        tunnel: w635 -> [w890]
        tunnel: [w891] -> w585
        tunnel: [w889] -> w584
        tunnel: [w896] -> w554
        tunnel: [w895] -> w605
        tunnel: w585 -> [w898]
        tunnel: w584 -> [w897]
        frame #0 {
          w886 = FALSE ("RESET")
          n144 = call "Wait"("Count(mSec)"=u16 3000 ("Count(uSec)")) -> ()  [unwired: 1 out]
          n145 = xnode "Read/Write Control"("FPGA VI Reference In"=w892, "error in"=w890, "RLY1"=w886, "RLY2"=w886, "HIREF"=w886, "Sprung0"=w886, "Sprung1"=w886, "ScanID"=u32 0, "Test"=FALSE, "RESET"=TRUE) -> ("FPGA VI Reference Out"=w891:refnum<k20>, "error out"=w889:errorcluster)
          n146 = local write "state"("SoftReset (3000 ms)" ("state")) -> ()
        }
        frame #1 {
          n147 = call "Wait5"("Count(mSec)"=u16 1000 ("Count(uSec)")) -> ()  [unwired: 1 out]
          n148 = xnode "Read/Write Control"("FPGA VI Reference In"=w898, "error in"=w897, "RESET"=FALSE) -> ("FPGA VI Reference Out"=w895:refnum<k20>, "error out"=w896:errorcluster)
        }
      }
      n149 = To Double Precision Float(number=i64 1000) -> (double precision float=w312:dbl)
      n150 = Add(x="manual time of data acquisition for experiment [s]", y="time before experiment [s]") -> (x+y=w334:T2)
      n151 = Multiply(x=w310, y=w312) -> (x*y=w309:dbl)
      n152 = Add(x="time after experiment [s]", y=w334) -> (x+y=w314:T2)
      n153 = Subtract(x=w314, y=w309) -> (x-y=→"experiment acqusition [s]":T2)
      n154 = xnode "Invoke Method"("FPGA VI Reference In"=w605, "error in"=w554, "Requested Depth"=u32 256) -> ("FPGA VI Reference Out"=w555:refnum<k20>, "error out"=w553:errorcluster)  [unwired: 1 out]
      n155 = local read "input DAC settings"() -> (w521:i64[])
      n156 = call "hFilterReg2014.vi"("error in"=w553, "Filter Modus"=w375, "Frequenz"=w376, "FPGA VI Reference In"=w555) -> ("error out"=w647:errorcluster, "FPGA VI Reference Out"=w646:refnum<k20>)  [unwired: 1 in, 1 out]
      n157 = To Unsigned Byte Integer(number=w521) -> (unsigned 8bit integer=w519:u8[])
      n158 = Divide(x=w314, y=w310) -> (x/y=w484:T2)
      n159 = case shown="0" "DAC and AD Settings" {
        tunnel: w647 -> [w1119 w1135]
        tunnel: w646 -> [w1121 w1134]
        tunnel: [w1116 w1133] -> w549
        tunnel: [w1120 w1128] -> w586
        tunnel: w519 -> [w1110 _]
        tunnel: u16 4280 -> [_ _]
        tunnel: u16 32952 -> [w1112 w1126]
        tunnel: u16 8376 -> [w1113 w1127]
        tunnel: u16 37048 -> [_ _]
        tunnel: u16 12472 -> [_ _]
        tunnel: u16 41144 -> [w1111 w1125]
        tunnel: u16 16568 -> [_ _]
        tunnel: u16 45240 -> [_ _]
        tunnel: u16 49336 -> [_ _]
        tunnel: u16 20664 -> [_ _]
        tunnel: u16 53432 -> [_ _]
        tunnel: u16 24760 -> [_ _]
        tunnel: u16 57528 -> [_ _]
        tunnel: u16 28856 -> [_ _]
        tunnel: u16 61624 -> [_ _]
        tunnel: "Global DAC Range [mV] Setting" -> [_ w1124]
        frame 1, Default {
          n160 = call "hModeRegRange2013.vi"("error in"=w1119, "RangeArray"=w1110, "Mode"=w1111, "FPGA VI Reference In"=w1121) -> ("error out"=w1114:errorcluster, "FPGA VI Reference Out"=w1118:refnum<k20>)  [unwired: 1 in, 1 out]
          n161 = call "hModeRegRange2013.vi"("error in"=w1114, "RangeArray"=w1110, "Mode"=w1112, "FPGA VI Reference In"=w1118) -> ("error out"=w1117:errorcluster, "FPGA VI Reference Out"=w1115:refnum<k20>)  [unwired: 1 in, 1 out]
          n162 = call "hModeRegRange2013.vi"("error in"=w1117, "RangeArray"=w1110, "Mode"=w1113, "FPGA VI Reference In"=w1115) -> ("error out"=w1116:errorcluster, "FPGA VI Reference Out"=w1120:refnum<k20>)  [unwired: 1 in, 1 out]
        }
        frame 0 {
          n163 = Initialize Array(w1124, 128 ("dimension size")) -> (w1122:u8[])
          n164 = local write "input DAC settings"(w1122) -> ()
          n165 = call "hModeReg2014.vi"("error in"=w1135, "Range"=w1124, "Mode"=w1125, "FPGA VI Reference In"=w1134) -> ("error out"=w1131:errorcluster, "FPGA VI Reference Out"=w1132:refnum<k20>)  [unwired: 1 in, 1 out]
          n166 = call "hModeReg2014.vi"("error in"=w1131, "Range"=w1124, "Mode"=w1126, "FPGA VI Reference In"=w1132) -> ("error out"=w1129:errorcluster, "FPGA VI Reference Out"=w1130:refnum<k20>)  [unwired: 1 in, 1 out]
          n167 = call "hModeReg2014.vi"("error in"=w1129, "Range"=w1124, "Mode"=w1127, "FPGA VI Reference In"=w1130) -> ("error out"=w1133:errorcluster, "FPGA VI Reference Out"=w1128:refnum<k20>)  [unwired: 1 in, 1 out]
        }
      }
      n168 = Round To Nearest(number=w484) -> (nearest integer value=w485:T2)
      n169 = To Unsigned Long Integer(number=w485) -> (unsigned 32bit integer=w315:u32)
      "No. of Samples:" <- w315
      n170 = To Double Precision Float(number=w315) -> (double precision float=w486:dbl)
      n171 = Multiply(x=w486, y=w310) -> (x*y=w487:dbl)
      n172 = Multiply(x=w487, y=1000.0) -> (x*y=→"predicted time [ms] to finalize DAQ":dbl)
      n173 = property on="Acquired Samples:" class="Slide (strict)"(error in=w549, "Scale.Range:Maximum"=w315) -> (error out=w548:errorcluster)  [unwired: 1 in, 1 out]
      n174 = Scale By Power Of 2(n=w519, x=sgl 10.0 ("Scale(mV)")) -> (x*2^n=w439:sgl[])
      n175 = disable-structure shown="Enabled" {
        frame Disabled {
          w740 = 5 items=["verify"=2, "reserve"=4, "commit"=3, "unreserve"=5, "abort"=6] ("ending task action")
          w739 = u16 0 items=["OK message + warnings"]
          # "channel preselection for output AO"
          n176 = call-poly <vilib>:"DAQmx Create Virtual Channel.vi"("maximum value"=10.0 ("maximum voltage @ 10MW single channel"), "minimum value"=-1.0, "physical channels"=tag "Dev1/ao0:1" ("Single Channel Output AO")) -> ("task out"=w757:refnum<k21>, "error out"=w754:errorcluster)  [unwired: 11 in]
          n177 = local write "voltage out state"("before SCVO loop") -> ()
          n178 = property class="DAQmx Write" props=["RegenMode", "NumChans"](reference=w757, error in=w754) -> (reference out=w755:refnum<k21>, error out=w732:errorcluster, "RegenMode"=w756:i32)  [unwired: 1 out]
          n179 = property class="DAQmx Channel"(reference=w755, error in=w732) -> (reference out=w733:refnum<k21>, error out=w731:errorcluster, "AO.DataXferReqCond"=w730:i32, "AO.DataXferMech"=w728:i32)
          n180 = call-poly <vilib>:"DAQmx Timing.vi"("task/channels in"=w733, "error in"=w731) -> ("sample mode"=w751:i32, "samples per channel"=w749:i32, "task out"=w723:refnum<k21>, "rate"=w729:dbl, "source"=w735:tag, "error out"=w722:errorcluster)  [unwired: 8 in]
          n181 = call-poly <vilib>:"DAQmx Write.vi"("task/channels in"=w723, "data"=dbl[] [0.0, 0.0], "error in"=w722) -> ("task out"=w725:refnum<k21>, "error out"=w724:errorcluster)  [unwired: 10 in, 1 out]
          n182 = Tick Count (ms)() -> (millisecond timer value=w734:u32)
          n183 = while {
            shift-right: [w786] -> w753
            shift-left: w725 -> [w762]
            shift-right: [w785] -> w752
            shift-left: w724 -> [w763]
            tunnel: w734 -> [w769]
            i -> [w765]
            stop <- w782 stop-if-true
            w781 = 9.9 ("AO Cutoff")
            w773 = 0.02 ("y")
            n184 = Tick Count (ms)() -> (millisecond timer value=w770:u32)
            n185 = Subtract(x=w770, y=w769) -> (x-y=w766:u32)
            n186 = Divide(x=w766, y=w765) -> (x/y=→"AO output loop timing":dbl)
            n187 = local write "voltage out state"("inside voltage loop") -> ()
            n188 = local read "single channel voltage [V]"() -> (w777:dbl)
            n189 = Greater Or Equal?(x=w777, y=w781) -> (x >= y?=w778:bool)
            n190 = case shown="True" w778 {
              tunnel: [w791 w792] -> w771
              tunnel: w777 -> [w791 _]
              tunnel: w781 -> [_ w792]
              frame False {
              }
              frame True {
              }
            }
            n191 = Less Or Equal?(x=w771, y=w773) -> (x <= y?=w775:bool)
            n192 = case shown="True" w775 {
              tunnel: [w789 0.025 ("AO Cutoff")] -> w761
              tunnel: w771 -> [w789 _]
              frame False {
              }
              frame True {
              }
            }
            "SCVO current val" <- w761
            n193 = local read "real time P_rad [MW, V]"() -> (w779:dbl)
            n194 = Greater Or Equal?(x=w779, y=w781) -> (x >= y?=w780:bool)
            n195 = case shown="False" w780 {
              tunnel: [w793 w794] -> w772
              tunnel: w779 -> [w793 _]
              tunnel: w781 -> [_ w794]
              frame False {
              }
              frame True {
              }
            }
            n196 = Less Or Equal?(x=w772, y=w773) -> (x <= y?=w774:bool)
            n197 = case shown="True" w774 {
              tunnel: [w787 0.025 ("AO Cutoff")] -> w760
              tunnel: w772 -> [w787 _]
              frame False {
              }
              frame True {
              }
            }
            "RTPVO current val" <- w760
            n198 = Build Array(w761, w760) -> (w759:dbl[])
            n199 = local read "Acquired Samples:"() -> (w768:u32)
            n200 = local read "No. of Samples:"() -> (w767:u32)
            n201 = call-poly <vilib>:"DAQmx Write.vi"("task/channels in"=w762, "data"=w759, "error in"=w763) -> ("task out"=w786:refnum<k21>, "error out"=w785:errorcluster)  [unwired: 10 in, 1 out]
            n202 = Unbundle By Name(w763) -> ("status"=w783:bool)  [unwired: 2 out]
            n203 = Greater Or Equal?(x=w768, y=w767) -> (x >= y?=w776:bool)
            n204 = Or(x=w783, y=w776) -> (x .or. y?=w782:bool)
            n205 = Not(x=w782) -> (.not. x?=→"voltage out loop status":bool)
            "AO error" <- w763
          }
          n206 = call-poly <vilib>:"DAQmx Write.vi"("task/channels in"=w753, "data"=dbl[] [0.0, 0.0], "error in"=w752) -> ("task out"=w745:refnum<k21>, "error out"=w744:errorcluster)  [unwired: 10 in, 1 out]
          n207 = call <vilib>:"DAQmx Control Task.vi"("task/channels in"=w745, "action"=w740, "error in"=w744) -> ("task out"=w742:refnum<k21>, "error out"=w743:errorcluster)  [unwired: 11 in]
          n208 = call <vilib>:"DAQmx Clear Task.vi"("task in"=w742, "error in"=w743) -> ("error out"=w736:errorcluster)  [unwired: 13 in]
          n209 = call <vilib>:"Simple Error Handler.vi"("type of dialog (OK msg:1)"=w739, "error in (no error)"=w736) -> ()  [unwired: 3 in, 5 out]
          n210 = Unbundle By Name(w736) -> ("status"=→"voltage status":bool, "source"=→"voltage errorsource":string)  [unwired: 1 out]
          "voltage out state" <- "passed SCVO loop"
        }
        frame Enabled {
          w795 = 5 items=["verify"=2, "reserve"=4, "commit"=3, "unreserve"=5, "abort"=6] ("action")
          w807 = u16 0 items=["OK message + warnings"]
          # "channel preselection for output AO"
          n211 = call-poly <vilib>:"DAQmx Create Virtual Channel.vi"("maximum value"=10.0 ("maximum voltage @ 10MW single channel"), "minimum value"=-1.0, "physical channels"=tag "Dev1/ao0:1" ("Single Channel Output AO")) -> ("task out"=w804:refnum<k21>, "error out"=w803:errorcluster)  [unwired: 11 in]
          n212 = local write "voltage out state"("before SCVO loop") -> ()
          n213 = call <vilib>:"DAQmx Start Task.vi"("task/channels in"=w804, "error in"=w803) -> ("task out"=w802:refnum<k21>, "error out"=w801:errorcluster)  [unwired: 12 in]
          n214 = Tick Count (ms)() -> (millisecond timer value=w805:u32)
          n215 = while {
            shift-right: [w843] -> w800
            shift-left: w802 -> [w824]
            shift-right: [w842] -> w799
            shift-left: w801 -> [w819]
            tunnel: w805 -> [w828]
            i -> [w820]
            stop <- w840 stop-if-true
            w839 = 9.9 ("AO Cutoff")
            w832 = 0.02 ("y")
            n216 = Tick Count (ms)() -> (millisecond timer value=w829:u32)
            n217 = Subtract(x=w829, y=w828) -> (x-y=w825:u32)
            n218 = control-ref of="single channel voltage [V]"() -> (w815:refnum<vi>)
            n219 = local write "AO loop counter"(w820) -> ()
            n220 = Divide(x=w825, y=w820) -> (x/y=w821:dbl)
            n221 = local write "AO output loop timing"(w821) -> ()
            n222 = local write "voltage out state"("inside voltage loop") -> ()
            n223 = property class="DigNum (strict)"(reference=w815) -> ("Value"=w814:dbl)  [unwired: 1 in, 2 out]
            n224 = Greater Or Equal?(x=w814, y=w839) -> (x >= y?=w836:bool)
            n225 = case shown="False" w836 {
              tunnel: [w848 w849] -> w830
              tunnel: w814 -> [w848 _]
              tunnel: w839 -> [_ w849]
              frame False {
              }
              frame True {
              }
            }
            n226 = Less Or Equal?(x=w830, y=w832) -> (x <= y?=w834:bool)
            n227 = case shown="True" w834 {
              tunnel: [w846 0.025 ("AO Cutoff")] -> w817
              tunnel: w830 -> [w846 _]
              frame False {
              }
              frame True {
              }
            }
            n228 = local write "SCVO current val"(w817) -> ()
            n229 = local read "real time P_rad [MW, V]"() -> (w837:dbl)
            n230 = Greater Or Equal?(x=w837, y=w839) -> (x >= y?=w838:bool)
            n231 = case shown="False" w838 {
              tunnel: [w850 w851] -> w831
              tunnel: w837 -> [w850 _]
              tunnel: w839 -> [_ w851]
              frame False {
              }
              frame True {
              }
            }
            n232 = Less Or Equal?(x=w831, y=w832) -> (x <= y?=w833:bool)
            n233 = case shown="True" w833 {
              tunnel: [w844 0.025 ("AO Cutoff")] -> w816
              tunnel: w831 -> [w844 _]
              frame False {
              }
              frame True {
              }
            }
            n234 = Build Array(w817, w816) -> (w823:dbl[])
            n235 = local write "RTPVO current val"(w816) -> ()
            n236 = local read "Acquired Samples:"() -> (w827:u32)
            n237 = local read "No. of Samples:"() -> (w826:u32)
            n238 = local write "AO error"(w819) -> ()
            n239 = call-poly <vilib>:"DAQmx Write.vi"("task/channels in"=w824, "data"=w823, "error in"=w819) -> ("task out"=w843:refnum<k21>, "error out"=w842:errorcluster)  [unwired: 10 in, 1 out]
            n240 = Unbundle By Name(w819) -> ("status"=w841:bool)  [unwired: 2 out]
            n241 = Greater Or Equal?(x=w827, y=w826) -> (x >= y?=w835:bool)
            n242 = Or(x=w841, y=w835) -> (x .or. y?=w840:bool)
            n243 = Not(x=w840) -> (.not. x?=w818:bool)
            n244 = local write "voltage out loop status"(w818) -> ()
          }
          n245 = local write "voltage out state"("passed SCVO loop") -> ()
          n246 = call <vilib>:"DAQmx Control Task.vi"("task/channels in"=w800, "action"=w795, "error in"=w799) -> ("task out"=w808:refnum<k21>, "error out"=w809:errorcluster)  [unwired: 11 in]
          n247 = call <vilib>:"DAQmx Clear Task.vi"("task in"=w808, "error in"=w809) -> ("error out"=w806:errorcluster)  [unwired: 13 in]
          n248 = call <vilib>:"Simple Error Handler.vi"("type of dialog (OK msg:1)"=w807, "error in (no error)"=w806) -> ()  [unwired: 3 in, 5 out]
          n249 = Unbundle By Name(w806) -> ("status"=w798:bool, "source"=w797:string)  [unwired: 1 out]
          n250 = local write "voltage errorsource"(w797) -> ()
          n251 = local write "voltage status"(w798) -> ()
        }
      }
      n252 = local read "time after experiment [s]"() -> (w411:dbl)
      n253 = Divide(x=w698, y=w634) -> (x/y=w559:dbl[][])
      n254 = local read "time before experiment [s]"() -> (w328:T2)
      n255 = local read "No. of Samples:"() -> (w408:u32)
      n256 = local read "sample time [s]"() -> (w412:sgl)
      n257 = flat-sequence {
        tunnel: w548 -> [w924]
        tunnel: w586 -> [w926]
        tunnel: [w925] -> w551
        tunnel: [w923] -> w550
        tunnel: [w922] -> w462
        tunnel: w461 -> [w920]
        tunnel: w460 -> [w921]
        tunnel: w459 -> [w919]
        tunnel: [w921] -> w454
        tunnel: [w920] -> w453
        tunnel: [w919] -> w452
        tunnel: w439 -> [w914]
        tunnel: [w913] -> w438
        tunnel: [w912] -> w433
        tunnel: w310 -> [w912]
        tunnel: [w911] -> w432
        tunnel: w330 -> [w911]
        tunnel: w551 -> [w968]
        tunnel: [w968] -> w547
        tunnel: w550 -> [w967]
        tunnel: [w967] -> w545
        tunnel: w317 -> [w960]
        tunnel: w394 -> [w958]
        tunnel: w471 -> [w959]
        tunnel: w405 -> [w947]
        tunnel: [w957] -> w467
        tunnel: [w956] -> w463
        tunnel: w462 -> [w955]
        tunnel: [w955] -> w455
        tunnel: w454 -> [w953]
        tunnel: w453 -> [w954]
        tunnel: w452 -> [w952]
        tunnel: [w954] -> w451
        tunnel: [w953] -> w450
        tunnel: [w952] -> w449
        tunnel: w438 -> [w951]
        tunnel: [w951] -> w434
        tunnel: w433 -> [w950]
        tunnel: w432 -> [w949]
        tunnel: [w950] -> w428
        tunnel: [w949] -> w426
        tunnel: [w947] -> w368
        tunnel: w547 -> [w987]
        tunnel: [w986] -> w546
        tunnel: w545 -> [w985]
        tunnel: [w984] -> w544
        tunnel: w315 -> [w983]
        tunnel: [w982] -> w468
        tunnel: w467 -> [w982]
        tunnel: [w981] -> w464
        tunnel: w463 -> [w981]
        tunnel: [w980] -> w456
        tunnel: w455 -> [w980]
        tunnel: w451 -> [w978]
        tunnel: w450 -> [w979]
        tunnel: w449 -> [w977]
        tunnel: [w979] -> w446
        tunnel: [w978] -> w443
        tunnel: [w977] -> w440
        tunnel: [w976] -> w435
        tunnel: w434 -> [w976]
        tunnel: [w975] -> w429
        tunnel: w428 -> [w975]
        tunnel: [w974] -> w427
        tunnel: w426 -> [w974]
        tunnel: [w973] -> w369
        tunnel: w368 -> [w973]
        tunnel: w546 -> [w998]
        tunnel: w544 -> [w999]
        tunnel: w317 -> [w1000]
        tunnel: [w998] -> w539
        tunnel: [w999] -> w538
        tunnel: [w989] -> w469
        tunnel: w468 -> [w989]
        tunnel: [w997] -> w465
        tunnel: w464 -> [w997]
        tunnel: [w996] -> w457
        tunnel: w456 -> [w996]
        tunnel: [w995] -> w447
        tunnel: w446 -> [w995]
        tunnel: [w994] -> w444
        tunnel: w443 -> [w994]
        tunnel: [w993] -> w441
        tunnel: w440 -> [w993]
        tunnel: [w992] -> w436
        tunnel: w435 -> [w992]
        tunnel: [w991] -> w430
        tunnel: w429 -> [w991]
        tunnel: w427 -> [w990]
        tunnel: [w990] -> w424
        tunnel: [w988] -> w370
        tunnel: w369 -> [w988]
        tunnel: w539 -> [w1016]
        tunnel: w538 -> [w1015]
        tunnel: [w1016] -> w537
        tunnel: [w1015] -> w536
        tunnel: [w1014] -> w535
        tunnel: [w1013] -> w470
        tunnel: w469 -> [w1013]
        tunnel: [w1012] -> w466
        tunnel: w465 -> [w1012]
        tunnel: [w1011] -> w458
        tunnel: w457 -> [w1011]
        tunnel: [w1010] -> w448
        tunnel: w447 -> [w1010]
        tunnel: [w1009] -> w445
        tunnel: w444 -> [w1009]
        tunnel: [w1008] -> w442
        tunnel: w441 -> [w1008]
        tunnel: [w1007] -> w437
        tunnel: w436 -> [w1007]
        tunnel: [w1006] -> w431
        tunnel: w430 -> [w1006]
        tunnel: [w1005] -> w425
        tunnel: w424 -> [w1005]
        tunnel: [w1004] -> w371
        tunnel: w370 -> [w1004]
        tunnel: w537 -> [w1054]
        tunnel: w536 -> [w1055]
        tunnel: w535 -> [w1047]
        tunnel: w315 -> [w1053]
        tunnel: w515 -> [w1018]
        tunnel: w534 -> [w1046]
        tunnel: w423 -> [w1019]
        tunnel: w439 -> [w1020]
        tunnel: [w1052] -> w533
        tunnel: [w1047] -> w532
        tunnel: [w1051] -> w531
        tunnel: [w1050] -> w530
        tunnel: [w1049] -> w529
        tunnel: [w1048] -> w528
        tunnel: w470 -> [w1017]
        tunnel: w466 -> [w1031]
        tunnel: w458 -> [w1044]
        tunnel: w448 -> [w1045]
        tunnel: w445 -> [w1042]
        tunnel: w442 -> [w1043]
        tunnel: w437 -> [w1041]
        tunnel: w431 -> [w1038]
        tunnel: w425 -> [w1037]
        tunnel: w405 -> [w1032]
        tunnel: [w1035] -> w420
        tunnel: [w1034] -> w417
        tunnel: [w1033] -> w414
        tunnel: [w1031] -> w374
        tunnel: [w1017] -> w373
        tunnel: [w1030] -> w372
        tunnel: w371 -> [w1030]
        tunnel: w532 -> [w1068]
        tunnel: w531 -> [w1067]
        tunnel: w530 -> [w1066]
        tunnel: w529 -> [w1065]
        tunnel: w528 -> [w1064]
        tunnel: [w1068] -> w481
        tunnel: [w1067] -> w480
        tunnel: [w1066] -> w479
        tunnel: [w1065] -> w478
        tunnel: [w1064] -> w477
        tunnel: [w1062] -> w476
        tunnel: [w1061] -> w421
        tunnel: w420 -> [w1061]
        tunnel: [w1060] -> w418
        tunnel: w417 -> [w1060]
        tunnel: [w1059] -> w415
        tunnel: w414 -> [w1059]
        tunnel: w374 -> [w1056]
        tunnel: w373 -> [w1057]
        tunnel: w372 -> [w1058]
        tunnel: [w1058] -> w367
        tunnel: [w1057] -> w366
        tunnel: [w1056] -> w365
        tunnel: w481 -> [w1076]
        tunnel: w480 -> [w1081]
        tunnel: w479 -> [w1080]
        tunnel: w478 -> [w1075]
        tunnel: w477 -> [w1079]
        tunnel: w476 -> [w1077]
        tunnel: [w1081] -> w475
        tunnel: [w1080] -> w474
        tunnel: [w1075] -> w473
        tunnel: [w1079] -> w472
        tunnel: [w1074] -> w422
        tunnel: w421 -> [w1074]
        tunnel: [w1073] -> w419
        tunnel: w418 -> [w1073]
        tunnel: [w1072] -> w416
        tunnel: w415 -> [w1072]
        tunnel: w367 -> [w1071]
        tunnel: w366 -> [w1070]
        tunnel: w365 -> [w1069]
        tunnel: [w1071] -> w364
        tunnel: [w1070] -> w363
        tunnel: [w1069] -> w362
        tunnel: [w1108] -> w526
        tunnel: [w1104] -> w318
        tunnel: [w1099] -> _
        tunnel: [w1109] -> w527
        tunnel: w475 -> [w1109]
        tunnel: w474 -> [_]
        tunnel: w473 -> [w1104]
        tunnel: w472 -> [w1108]
        tunnel: w422 -> [w1105]
        tunnel: w419 -> [w1106]
        tunnel: [w1100] -> _
        tunnel: w416 -> [_]
        tunnel: w364 -> [w1103]
        tunnel: w363 -> [w1102]
        tunnel: w362 -> [w1101]
        frame #0 {
          w915 = 0.002  # Range=2*RawScale (mV)
          n258 = Multiply(x=w915, y=w914) -> (x*y=w916:dbl[])
          n259 = Scale By Power Of 2 "Volts/bit"(n=i16 -16, x=w916) -> (x*2^n=w917:dbl[])
          n260 = To Single Precision Float(number=w917) -> (single precision float=w913:sgl[])
          n261 = for {
            N: w920 -> [_]
            tunnel: w921 -> [w936]
            tunnel: w919 -> [w934]
            shift-right: [w928] -> w922
            shift-left: 0.0 -> [w929]
            i -> [w935]
            n262 = Index Array(array=w934, index (row)=w935, index (col)=0 ("disabled index (col)")) -> (element=w931:i64)
            n263 = Index Array(array=w936, index (row)=w931, index (col)=1 ("disabled index (col)")) -> (element=w932:dbl)
            n264 = Add(x=w929, y=w932) -> (x+y=w928:dbl)
          }
          n265 = call "hComRegStart2013.vi"("error in"=w924, "FPGA VI Reference In"=w926) -> ("error out"=w923:errorcluster, "FPGA VI Reference Out"=w925:refnum<k20>)  [unwired: 3 in, 1 out]
          n266 = local write "state"("Calibration Done" ("state")) -> ()
          n267 = call "Wait4"("Count(mSec)"=u32 1000) -> ()  [unwired: 1 out]
        }
        frame #1 {
          n268 = local read "time before experiment [s]"() -> (w948:T2)
          n269 = Subtract(x="time between VI start and points of interest [s]", y=w948) -> (x-y=w946:T2)
          "Total wait time  [s]" <- w946
          n270 = Multiply(x=T2 1000.0, y=w946) -> (x*y=w944:T2)
          n271 = Tick Count (ms)() -> (millisecond timer value=w964:u32)
          n272 = To Unsigned Long Integer(number=w944) -> (unsigned 32bit integer=w943:u32)
          n273 = Add(x=w960, y=w943) -> (x+y=w962:u32)
          n274 = call "power_factors.vi"("TauM"=w947, "KappaM"=w958, "RMESS"=w959) -> ("F_ch"=w957:dbl[], "tau_fact"=w956:dbl[])  [unwired: 7 in]
          n275 = Subtract(x=w962, y=w964) -> (x-y=w942:u32)
          n276 = Divide(x=w942, y=u32 1000) -> (x/y=→"Calibration Time [s]":dbl)
          n277 = Subtract(x=w942, y=u32 50) -> (x-y=w938:u32)
          n278 = Add(x=w964, y=w938) -> (x+y=w965:u32)
          n279 = Divide(x=w938, y=u32 1000) -> (x/y=→"Countdown Time [s]":dbl)
          n280 = while {
            tunnel: w965 -> [w971]
            stop <- w972 continue-if-true
            n281 = Tick Count (ms)() -> (millisecond timer value=w970:u32)
            n282 = Subtract(x=w971, y=w970) -> (x-y=w969:u32)
            "DAQ Timer" <- w969
            n283 = Greater?(x=w971, y=w970) -> (0:w972:bool)
            n284 = local write "DAQ Timer"(w969) -> ()
          }
          n285 = local write "state"("Countdown Timer" ("state")) -> ()
        }
        frame #2 {
          # "takes 50 ms"
          n286 = call "hSync&StartSampling2013.vi"("error in"=w985, "#Samples"=w983, "FPGA VI Reference In"=w987) -> ("error out"=w984:errorcluster, "FPGA VI Reference Out"=w986:refnum<k20>)  [unwired: 1 in]
        }
        frame #3 {
          n287 = Tick Count (ms)() -> (millisecond timer value=w1001:u32)
          n288 = local write "state"("SyncRun" ("state")) -> ()
          n289 = Subtract(x=w1001, y=w1000) -> (x-y=→"data acquisition wait\ntime [ms]":u32)
        }
        frame #4 {
          n290 = call "Tick Count"() -> ("Tick Count(mSec)"=w1014:u32)
        }
        frame #5 {
          # "RTPr factor"
          n291 = local read "single channel signal factor"() -> (w1040:dbl)
          n292 = control-ref of="single channel voltage [V]"() -> (w1026:refnum<vi>)
          n293 = control-ref of="single channel voltage array"() -> (w1025:refnum<vi>)
          n294 = control-ref of="real time P_rad [MW, V]"() -> (w1028:refnum<vi>)
          n295 = control-ref of="real time P_rad array"() -> (w1027:refnum<vi>)
          n296 = local read "single channel number"() -> (w1039:i64)
          n297 = Bundle("real time P_rad [MW, V]"=w1028, "real time P_rad array"=w1027, "single channel voltage [V]"=w1026, "single channel voltage array"=w1025) -> (w1024:T26)  [unwired: 1 in]
          n298 = Bundle("Array"=w1046, w1020, "Array 2"=w1019, "all rows"=w1018, "F_ch"=w1017, "tau_fact"=w1031, "all rows"=w1045, w1044, w1041, "single channel signal factor"=w1040, "set sample time [s]"=w1038, w1037, "ArrayOutput"=w1032, "all rows"=w1043, w1042, "single channel number"=w1039) -> (w1036:T27)  [unwired: 1 in]
          n299 = call "hReadChannels-UandP.vi"("FPGA VI Reference In"=w1054, "Nsamples"=w1053, "error in"=w1055, "output cluster"=w1024, "No. Of Samples to average"=10, "variables cluster"=w1036, "skip feedback"="skip feedback") -> ("Fehler"=w1052:bool, "AdjustedArray"=w1033:sgl[][], "loop DAQ timing"=→"loop DAQ timing [ms]":dbl, "single channel voltage array"=w1034:dbl[], "real time P_rad array"=w1035:dbl[], "FPGA VI Reference Out"=w1051:refnum<k20>, "PowerArray"=w1050:sgl[][], "RawArray"=w1049:sgl[][], "error out"=w1048:errorcluster)  [unwired: 12 in]
          "single channel voltage array" <- w1034
          "real time P_rad array" <- w1035
          n300 = local write "state"("Acquiring Data..." ("state")) -> ()
        }
        frame #6 {
          n301 = call "Tick Count2"() -> ("Tick Count(mSec)"=w1062:u32)
          n302 = local write "state"("Acquisition done" ("state")) -> ()
        }
        frame #7 {
          n303 = Subtract(x=w1077, y=w1076) -> (x-y=→"Measured Time for DAQ [ms]":u32)
        }
        frame #8 {
          w1088 = 1000
          n304 = local read "time after experiment [s]"() -> (w1083:dbl)
          n305 = local read "No. of Samples:"() -> (w1089:u32)
          n306 = local read "time before experiment [s]"() -> (w1090:T2)
          n307 = local read "sample time [s]"() -> (w1091:sgl)
          n308 = local read "kbolott_and_volume"() -> (w1092:dbl[][])
          n309 = Subtract(x=w1089, y=w1088) -> (x-y=w1086:u32)
          n310 = call "rawpower2totalprad.vi"("SampleTime"=w1091, "width"=1 ("spike width"), "threshold"=1.0 ("spike threshold"), "Pre-start time (ms) of\nDAQ"=w1090, "AddOnTime"=w1083, "samples to exclude"=w1088, "kbolott_and_volume"=w1092, "No. of Samples\n[TOA / Sample Rate]"=w1086, "tau_fact"=w1101, "F_ch"=w1102, "TauM"=w1103, "RawArray"=w1104) -> ("corrected voltage array"=w1100:dbl[][], "AdjustedPower"=w1099:dbl[][], "P_rad HBC [MW]"=w1087:dbl[], "P_rad VBC [MW]"=w1082:dbl[])  [unwired: 12 in]
          "full P_rad [MW] HBC" <- w1087
          "full P_rad [MW] VBC" <- w1082
          n311 = local read "nsample array [s]"() -> (w1094:dbl[])
          n312 = Build Cluster Array(w1094, w1087) -> (w1095:cluster{dbl, "element":dbl}[])
          n313 = Build Cluster Array(w1094, w1106) -> (w1098:cluster{dbl, "element":dbl}[])
          n314 = Build Cluster Array(w1094, w1105) -> (w1097:cluster{dbl, "element":dbl}[])
          n315 = Build Cluster Array(w1094, w1082) -> (w1093:cluster{dbl, "element":dbl}[])
          n316 = Build Cluster Array(w1095, w1098, w1097, w1093) -> (→"all plot":cluster{cluster{dbl, "element":dbl}[]}[])
          n317 = local write "state"("Calculating full radiated power ..." ("state")) -> ()
        }
      }
      n318 = Initialize Array(0.0, w408) -> (w410:dbl[])
      n319 = Multiply(x=w412, y=w411) -> (x*y=w413:dbl)
      n320 = for {
        N: w408 -> [_]
        shift-right: [w721] -> w409
        shift-left: w410 -> [w720]
        tunnel: w412 -> [w719]
        tunnel: w413 -> [w713]
        tunnel: w328 -> [w715]
        i -> [w717]
        n321 = To Double Precision Float(number=w717) -> (double precision float=w718:dbl)
        n322 = Multiply(x=w719, y=w718) -> (x*y=w716:dbl)
        n323 = Subtract(x=w716, y=w715) -> (x-y=w714:T2)
        n324 = Add(x=w714, y=w713) -> (x+y=w712:T2)
        n325 = Replace Array Subset(array=w720, new element=w712, index=w717) -> (w721:dbl[])
      }
      n326 = call "CalFaktor-128.vi"("CalCurrent(t)"=w559, "Rload"=w634, "Rcable"=w522) -> ("Amplitude"=→"AmplitudeMeas":dbl[], "FitData"=w406:dbl[][], "Kappa"=w394:dbl[], "RB01"=w329:dbl[], "Tau"=w327:dbl[], "Damping"=→"DampingMeas":dbl[])  [unwired: 6 in, 1 out]
      "kappaM [A²]" <- w394
      n327 = local write "nsample array [s]"(w409) -> ()
      n328 = for {
        N: w398 -> [_]
        tunnel: [w711] -> w389 mode=indexing
        shift-right: [w711] -> _
        shift-left: 0.0 -> [w710]
        w709 = 1.0  # TimeStep
        n329 = Add(x=w710, y=w709) -> (x+y=w711:dbl)
      }
      n330 = call "Cal(SubVI).vi"("Array"=w559, "dt"=w652, "StartChan"=64 ("ChanStart"), "tstart"=w653, "FitData"=w406) -> ("plot(Signals) 1-32"=→"MessCal 65 - 80":T28, "plot(Signals) 33-64"=→"MessCal 81 - 96":T29)  [unwired: 9 in]
      n331 = call "Cal(SubVI).vi"("Array"=w559, "dt"=w652, "StartChan"=96 ("ChanStart"), "tstart"=w653, "FitData"=w406) -> ("plot(Signals) 1-32"=→"MessCal 97 - 112":T28, "plot(Signals) 33-64"=→"MessCal 113 - 128":T29)  [unwired: 9 in]
      n332 = call "Cal(SubVI).vi"("Array"=w559, "dt"=w652, "StartChan"=32 ("ChanStart"), "tstart"=w653, "FitData"=w406) -> ("plot(Signals) 1-32"=→"MessCal 33 - 49":T28, "plot(Signals) 33-64"=→"MessCal 49 - 64":T29)  [unwired: 9 in]
      n333 = call "Cal(SubVI).vi"("Array"=w559, "dt"=w652, "StartChan"=0 ("ChanStart"), "tstart"=w653, "FitData"=w406) -> ("plot(Signals) 1-32"=→"MessCal 1-16":T28, "plot(Signals) 33-64"=→"MessCal 17-32":T29)  [unwired: 9 in]
      n334 = Build Cluster Array(w389, w394) -> (w395:cluster{dbl, dbl}[])
      n335 = Build Cluster Array(w389, w327) -> (w390:cluster{dbl, dbl}[])
      n336 = Build Cluster Array(w389, w329) -> (w392:cluster{dbl, dbl}[])
      n337 = Build Cluster Array(w395) -> (→"kappa_meas":cluster{cluster{dbl, dbl}[]}[])
      n338 = Build Cluster Array(w390) -> (→"tau_meas":cluster{cluster{dbl, dbl}[]}[])
      n339 = Build Cluster Array(w392) -> (→"Rmeas":cluster{cluster{dbl, dbl}[]}[])
      n340 = Array Subset(array=w559, index (row)=0 ("index"), length (row)=128 ("length")) -> (w558:dbl[][])  [unwired: 2 in]
      n341 = case shown="False" "load calibration values from file?" {
        tunnel: [w1137 w1139] -> w404
        tunnel: [w1136 w1140] -> w630
        tunnel: [w1138 w1141] -> w515
        tunnel: w327 -> [w1138 _]
        tunnel: w329 -> [w1137 _]
        tunnel: w394 -> [w1136 _]
        frame False {
        }
        frame True {
          n342 = call-poly <vilib>:"Read From Spreadsheet File.vi"("delimiter (\\t)"="    " ("delimiter (\\t)"), "transpose (no:F)"=TRUE, "format (%.3f)"="%.12f" ("format (%d)"), "max characters/row  (no limit:0)"=0, "start of read offset (chars.:0)"=47, "number of rows (all:-1)"=-1, "file path (dialog if empty)"="file location") -> ("all rows"=w1142:dbl[][])  [unwired: 4 out]
          n343 = Index Array(array=w1142, index (row)=0 ("index")) -> (element=w1140:dbl[])  [unwired: 1 in]
          "kappa [A²]" <- w1140
          n344 = Index Array(array=w1142, index (row)=1 ("index")) -> (element=w1139:dbl[])  [unwired: 1 in]
          "taum [s]" <- w1139
          n345 = Index Array(array=w1142, index (row)=2 ("index")) -> (element=w1141:dbl[])  [unwired: 1 in]
          "roh [Ohm]" <- w1141
        }
      }
      n346 = call "Arraylimit128.vi"("LowerLimit"=400.0, "Array Input"=w329, "UpperLimit"=2000.0) -> ("BoolArray"=w689:bool[], "ArrayOutput"=w471:dbl[])
      "rohM [Ohm]" <- w471
      n347 = call "Arraylimit128.vi"("LowerLimit"=2e-05, "Array Input"=w394, "UpperLimit"=0.002) -> ("BoolArray"=w691:bool[])  [unwired: 1 out]
      n348 = call "Arraylimit128.vi"("LowerLimit"=0.001, "Array Input"=w327, "UpperLimit"=0.8) -> ("BoolArray"=w690:bool[], "ArrayOutput"=w405:dbl[])
      "TauM" <- w405
      n349 = Add(x=w522, y=w634) -> (x+y=w633:dbl)
      n350 = Multiply(x=w633, y=2.0) -> (x*y=w631:dbl)
      n351 = call "U2PCoeff.vi"("Numeric"=w631, "Kappa00"=w630, "RB000"=w404) -> ("Array"=w534:dbl[], "Array 2"=w423:dbl[])
      n352 = Compound Arithmetic op=OR(w691, w690, w689) -> (w678:bool[])
      n353 = Array Subset(array=w678, index=0, length=32) -> (w355:bool[])
      "MessStatus 1-32" <- w355
      n354 = Array Subset(array=w678, index=32, length=32) -> (w357:bool[])
      "MessStatus 33-64" <- w357
      n355 = Array Subset(array=w678, index=96, length=32) -> (w361:bool[])
      "MessStatus 97-128" <- w361
      n356 = Array Subset(array=w678, index=64, length=32) -> (w359:bool[])
      "MessStatus 65-96" <- w359
      n357 = Equal?(x=w355, y=w354) -> (x = y?=w353:bool)
      n358 = Equal?(x=w357, y=w356) -> (x = y?=w352:bool)
      n359 = Equal?(x=w359, y=w358) -> (x = y?=w351:bool)
      n360 = Equal?(x=w361, y=w360) -> (x = y?=w350:bool)
      n361 = Compound Arithmetic op=AND(w353, w352, w351, w350) -> (→"MeasFoilStatus":bool)
      n362 = Divide(x=w657, y=w634) -> (x/y=w403:dbl[][])
      n363 = call "CalFaktor-128.vi"("CalCurrent(t)"=w403, "Rload"=w634, "Rcable"=w522) -> ("Amplitude"=→"AmplitudeRef":dbl[], "FitData"=w523:dbl[][], "Kappa"=w378:dbl[], "RB01"=w379:dbl[], "Tau"=w377:dbl[], "Damping"=→"DampingRef":dbl[])  [unwired: 6 in, 1 out]
      n364 = for {
        N: w388 -> [_]
        tunnel: [w708] -> w380 mode=indexing
        shift-right: [w708] -> _
        shift-left: 0.0 -> [w707]
        w706 = 1.0  # TimeStep
        n365 = Add(x=w707, y=w706) -> (x+y=w708:dbl)
      }
      n366 = Build Cluster Array(w380, w378) -> (w386:cluster{dbl, dbl}[])
      n367 = Build Cluster Array(w380, w377) -> (w384:cluster{dbl, dbl}[])
      n368 = Build Cluster Array(w380, w379) -> (w385:cluster{dbl, dbl}[])
      n369 = Build Cluster Array(w386) -> (→"kappa_ref":cluster{cluster{dbl, dbl}[]}[])
      n370 = Build Cluster Array(w384) -> (→"tau_ref":cluster{cluster{dbl, dbl}[]}[])
      n371 = Build Cluster Array(w385) -> (→"Rref":cluster{cluster{dbl, dbl}[]}[])
      n372 = Array Subset(array=w403, index (row)=0 ("index"), length (row)=128 ("length")) -> (w482:dbl[][])  [unwired: 2 in]
      n373 = local read "time before experiment [s]"() -> (w324:T2)
      n374 = call "Arraylimit128.vi"("LowerLimit"=2e-05, "Array Input"=w378, "UpperLimit"=0.002) -> ("BoolArray"=w664:bool[], "ArrayOutput"=→"kappaR [A²]":dbl[])
      n375 = call "Arraylimit128.vi"("LowerLimit"=0.001, "Array Input"=w377, "UpperLimit"=0.8) -> ("BoolArray"=w665:bool[], "ArrayOutput"=w511:dbl[])
      "tauR [s]" <- w511
      n376 = To Double Precision Float(number=1000) -> (double precision float=w320:dbl)
      n377 = Multiply(x=w310, y=w320) -> (x*y=w323:dbl)
      n378 = call "Cal(SubVI).vi"("Array"=w403, "dt"=w648, "StartChan"=0 ("ChanStart"), "tstart"=w649, "FitData"=w523) -> ("plot(Signals) 1-32"=→"RefCal 1-16":T28, "plot(Signals) 33-64"=→"RefCal 17-32":T29)  [unwired: 9 in]
      n379 = call "Cal(SubVI).vi"("Array"=w403, "dt"=w648, "StartChan"=32 ("ChanStart"), "tstart"=w649, "FitData"=w523) -> ("plot(Signals) 1-32"=→"RefCal 33 - 48":T28, "plot(Signals) 33-64"=→"RefCal 49 - 64":T29)  [unwired: 9 in]
      n380 = call "Cal(SubVI).vi"("Array"=w403, "dt"=w648, "StartChan"=64 ("ChanStart"), "tstart"=w649, "FitData"=w523) -> ("plot(Signals) 1-32"=→"RefCal 65 - 80":T28, "plot(Signals) 33-64"=→"RefCal 81 - 96":T29)  [unwired: 9 in]
      n381 = call "Cal(SubVI).vi"("Array"=w403, "dt"=w648, "StartChan"=96 ("ChanStart"), "tstart"=w649, "FitData"=w523) -> ("plot(Signals) 1-32"=→"RefCal 97 - 112":T28, "plot(Signals) 33-64"=→"RefCal 113 - 128":T29)  [unwired: 9 in]
      n382 = Array Subset(array=w523, index (row)=0 ("index"), length (row)=128 ("length")) -> (w562:dbl[][])  [unwired: 2 in]
      n383 = Subtract(x=w324, y=w323) -> (x-y=w322:T2)
      n384 = call "Arraylimit128.vi"("LowerLimit"=400.0, "Array Input"=w379, "UpperLimit"=2000.0) -> ("BoolArray"=w666:bool[], "ArrayOutput"=w541:dbl[])
      "rohR [Ohm]" <- w541
      n385 = Negate(x=w322) -> (-x=w321:T2)
      n386 = Array Subset(array=w318, index (row)=0 ("index"), length (row)=128 ("length")) -> (w542:sgl[][])  [unwired: 2 in]
      n387 = Array Subset(array=w318, index (row)=64, length (row)=64, index (col)=0) -> (w543:sgl[][])  [unwired: 1 in]
      n388 = Array Subset(array=w318, index (row)=0, length (row)=64, index (col)=0) -> (w540:sgl[][])  [unwired: 1 in]
      n389 = call "Visualize_Signals64.vi"("FPGSampleTime"=w310, "tstart"=w321, "Signals"=w543) -> ("plot(Signals) 33-64"=→"Raw 97 - 128":T25, "plot(Signals) 1-32"=→"Raw 65 - 97":T5)  [unwired: 7 in]
      n390 = call "Visualize_Signals64.vi"("FPGSampleTime"=w310, "tstart"=w321, "Signals"=w540) -> ("plot(Signals) 33-64"=→"Raw 33-64":T25, "plot(Signals) 1-32"=→"Raw 1-32":T5)  [unwired: 7 in]
      n391 = Compound Arithmetic op=OR(w664, w665, w666) -> (w677:bool[])
      n392 = Array Subset(array=w406, index (row)=0 ("index"), length (row)=128 ("length")) -> (w512:dbl[][])  [unwired: 2 in]
      n393 = Array Subset(array=w677, index=0, length=32) -> (w348:bool[])
      "RefStatus 1-32" <- w348
      n394 = Array Subset(array=w677, index=32, length=32) -> (w346:bool[])
      "RefStatus 33-64" <- w346
      n395 = Array Subset(array=w677, index=64, length=32) -> (w344:bool[])
      "RefStatus 65-96" <- w344
      n396 = Array Subset(array=w677, index=96, length=32) -> (w342:bool[])
      "RefStatus 97-128" <- w342
      n397 = Equal?(x=w348, y=w347) -> (x = y?=w340:bool)
      n398 = Equal?(x=w344, y=w343) -> (x = y?=w338:bool)
      n399 = Equal?(x=w346, y=w345) -> (x = y?=w339:bool)
      n400 = Equal?(x=w342, y=w341) -> (x = y?=w337:bool)
      n401 = Compound Arithmetic op=AND(w340, w339, w338, w337) -> (→"RefFoilStatus":bool)
      n402 = disable-structure shown="Disabled" {
        disable-tunnel: w318 -> [w861 _]
        disable-tunnel: w511 -> [w860 _]
        disable-tunnel: w378 -> [w859 _]
        disable-tunnel: w541 -> [w858 _]
        disable-tunnel: w540 -> [w857 _]
        disable-tunnel: w405 -> [w856 _]
        disable-tunnel: w394 -> [w855 _]
        disable-tunnel: w471 -> [w854 _]
        disable-tunnel: w321 -> [w853 _]
        disable-tunnel: w310 -> [w852 _]
        frame Disabled {
          n403 = call "W7-X-Bolo-TMDS-LOCAL.vi"("Kappa 2"=w859, "ArrayOutput 4"=w860, "ArrayOutput 3"=w858, "Array"=w857, "RawArray"=w861, "Numeric"=w853, "ArrayOutput"=w854, "Kappa"=w855, "ArrayOutput 2"=w856, "SampleTime"=w852) -> ()  [unwired: 5 in, 1 out]
        }
        frame Enabled {
        }
      }
      "Fehler READ U+P" <- w533
    }
    frame True {
      n404 = local write "state"("Error->NoRead" ("state")) -> ()
    }
  }
  n405 = Multiply(x=w162, y=w161) -> (x*y=w145:i64)
  n406 = xnode "Read/Write Control"("FPGA VI Reference In"=w183) -> ("FPGA VI Reference Out"=w182:refnum<k20>, "SampleTrigger2"=w184:u32)  [unwired: 1 in, 1 out]
  n407 = To Quad Integer(1:w184) -> (0:w178:i64)
  "Pre-samples (If -1, then no trigger) detected)" <- w178
  n408 = flat-sequence {
    tunnel: w186 -> [w1192]
    tunnel: w222 -> [w1193]
    tunnel: w182 -> [w1194]
    tunnel: [w1194] -> w181
    tunnel: [w1193] -> w180
    tunnel: [w1192] -> w179
    tunnel: w145 -> [w1191]
    tunnel: w178 -> [w1190]
    tunnel: w2 -> [w1170]
    tunnel: w160 -> [w1169]
    tunnel: w159 -> [w1168]
    tunnel: w158 -> [w1167]
    tunnel: w157 -> [w1166]
    tunnel: w156 -> [w1165]
    tunnel: w155 -> [w1156]
    tunnel: [w1187] -> w154
    tunnel: [w1186] -> w153
    tunnel: [w1185] -> w152
    tunnel: [w1184] -> w151
    tunnel: [w1183] -> w150
    tunnel: [w1182] -> w149
    tunnel: [w1181] -> w148
    tunnel: [w1180] -> w147
    tunnel: [w1179] -> w146
    tunnel: w145 -> [w1179]
    tunnel: [w1178] -> w141
    tunnel: [w1176] -> w136
    tunnel: w84 -> [w1176]
    tunnel: [w1177] -> w133
    tunnel: w132 -> [w1177]
    tunnel: [w1175] -> w130
    tunnel: w129 -> [w1175]
    tunnel: [w1174] -> w127
    tunnel: w108 -> [w1174]
    tunnel: [w1173] -> w107
    tunnel: w104 -> [w1173]
    tunnel: [w1172] -> w83
    tunnel: [w1171] -> w76
    tunnel: [w1164] -> w72
    tunnel: [w1163] -> w71
    tunnel: [w1162] -> w63
    tunnel: [w1161] -> w56
    tunnel: [w1157] -> w52
    tunnel: [w1229] -> w177
    tunnel: [w1228] -> w176
    tunnel: [w1227] -> w175
    tunnel: w181 -> [w1229]
    tunnel: w180 -> [w1228]
    tunnel: w179 -> [w1227]
    tunnel: w154 -> [w1217]
    tunnel: w153 -> [w1216]
    tunnel: w152 -> [w1215]
    tunnel: w151 -> [w1214]
    tunnel: w150 -> [w1213]
    tunnel: w149 -> [w1212]
    tunnel: w148 -> [w1211]
    tunnel: w147 -> [w1210]
    tunnel: w146 -> [w1222]
    tunnel: [w1223] -> w142
    tunnel: w141 -> [w1223]
    tunnel: [w1222] -> w140
    tunnel: [w1221] -> w137
    tunnel: w136 -> [w1221]
    tunnel: [w1220] -> w134
    tunnel: w133 -> [w1220]
    tunnel: [w1219] -> w131
    tunnel: w130 -> [w1219]
    tunnel: [w1218] -> w128
    tunnel: w127 -> [w1218]
    tunnel: [w1217] -> w123
    tunnel: [w1216] -> w121
    tunnel: [w1215] -> w119
    tunnel: [w1214] -> w117
    tunnel: [w1213] -> w115
    tunnel: [w1212] -> w113
    tunnel: [w1211] -> w111
    tunnel: [w1210] -> w109
    tunnel: w107 -> [w1209]
    tunnel: [w1209] -> w106
    tunnel: w83 -> [w1208]
    tunnel: [w1208] -> w80
    tunnel: [w1207] -> w77
    tunnel: w76 -> [w1207]
    tunnel: w72 -> [w1205]
    tunnel: w71 -> [w1206]
    tunnel: [w1206] -> w70
    tunnel: [w1205] -> w69
    tunnel: w63 -> [w1204]
    tunnel: [w1204] -> w62
    tunnel: [w1203] -> w57
    tunnel: w56 -> [w1203]
    tunnel: [w1202] -> w53
    tunnel: w52 -> [w1202]
    tunnel: w177 -> [w1257]
    tunnel: [w1257] -> w174
    tunnel: w176 -> [w1256]
    tunnel: [w1256] -> w173
    tunnel: w175 -> [w1255]
    tunnel: [w1255] -> w171
    tunnel: [w1252] -> w144
    tunnel: [w1251] -> w143
    tunnel: w142 -> [w1251]
    tunnel: w140 -> [w1250]
    tunnel: [w1250] -> w139
    tunnel: [w1249] -> w138
    tunnel: w137 -> [w1249]
    tunnel: [w1248] -> w135
    tunnel: w134 -> [w1248]
    tunnel: w131 -> [w1246]
    tunnel: w128 -> [w1247]
    tunnel: [w1247] -> w126
    tunnel: [w1246] -> w125
    tunnel: [w1245] -> w124
    tunnel: w123 -> [w1245]
    tunnel: [w1244] -> w122
    tunnel: w121 -> [w1244]
    tunnel: [w1243] -> w120
    tunnel: w119 -> [w1243]
    tunnel: [w1242] -> w118
    tunnel: w117 -> [w1242]
    tunnel: [w1241] -> w116
    tunnel: w115 -> [w1241]
    tunnel: [w1240] -> w114
    tunnel: w113 -> [w1240]
    tunnel: [w1230] -> w112
    tunnel: w111 -> [w1230]
    tunnel: [w1239] -> w110
    tunnel: w109 -> [w1239]
    tunnel: w106 -> [w1238]
    tunnel: [w1238] -> w105
    tunnel: [w1237] -> w81
    tunnel: w80 -> [w1237]
    tunnel: [w1236] -> w78
    tunnel: w77 -> [w1236]
    tunnel: w70 -> [w1234]
    tunnel: w69 -> [w1235]
    tunnel: [w1235] -> w67
    tunnel: [w1234] -> w65
    tunnel: w62 -> [w1233]
    tunnel: [w1233] -> w60
    tunnel: [w1232] -> w58
    tunnel: w57 -> [w1232]
    tunnel: [w1231] -> w54
    tunnel: w53 -> [w1231]
    tunnel: w174 -> [w1304]
    tunnel: w173 -> [w1303]
    tunnel: [w1303] -> w172
    tunnel: w171 -> [w1305]
    tunnel: [w1305] -> w170
    tunnel: w144 -> [w1271]
    tunnel: w143 -> [w1317]
    tunnel: w139 -> [w1268]
    tunnel: w138 -> [w1316]
    tunnel: w135 -> [w1315]
    tunnel: w126 -> [w1294]
    tunnel: w125 -> [w1293]
    tunnel: w124 -> [w1313]
    tunnel: w122 -> [w1312]
    tunnel: w120 -> [w1311]
    tunnel: w118 -> [w1310]
    tunnel: w116 -> [w1309]
    tunnel: w114 -> [w1308]
    tunnel: w112 -> [w1307]
    tunnel: w110 -> [w1306]
    tunnel: w105 -> [w1314]
    tunnel: [w1294] -> w103
    tunnel: [w1293] -> w102
    tunnel: [w1316] -> w101
    tunnel: [w1315] -> w100
    tunnel: [w1314] -> w99
    tunnel: [w1313] -> w98
    tunnel: [w1312] -> w97
    tunnel: [w1311] -> w96
    tunnel: [w1310] -> w95
    tunnel: [w1309] -> w94
    tunnel: [w1308] -> w93
    tunnel: [w1307] -> w92
    tunnel: [w1306] -> w91
    tunnel: [w1304] -> w90
    tunnel: [w1302] -> w89
    tunnel: [w1301] -> w88
    tunnel: [w1300] -> w87
    tunnel: [w1299] -> w86
    tunnel: [w1298] -> w85
    tunnel: [w1283] -> w82
    tunnel: w81 -> [w1283]
    tunnel: [w1282] -> w79
    tunnel: w78 -> [w1282]
    tunnel: [w1281] -> w68
    tunnel: w67 -> [w1281]
    tunnel: [w1280] -> w66
    tunnel: w65 -> [w1280]
    tunnel: [w1261] -> w64
    tunnel: [w1269] -> w61
    tunnel: w60 -> [w1269]
    tunnel: [w1267] -> w59
    tunnel: w58 -> [w1267]
    tunnel: [w1266] -> w55
    tunnel: w54 -> [w1266]
    tunnel: w172 -> [w1448]
    tunnel: w170 -> [w1450]
    tunnel: [w1450] -> w51
    tunnel: [w1449] -> w49
    tunnel: [w1448] -> w47
    tunnel: w103 -> [w1451]
    tunnel: w102 -> [w1440]
    tunnel: w101 -> [w1441]
    tunnel: w100 -> [w1447]
    tunnel: w99 -> [w1446]
    tunnel: w98 -> [w1443]
    tunnel: w97 -> [w1442]
    tunnel: w96 -> [w1456]
    tunnel: w95 -> [w1455]
    tunnel: w94 -> [w1454]
    tunnel: w93 -> [w1453]
    tunnel: w92 -> [w1452]
    tunnel: w91 -> [w1445]
    tunnel: w90 -> [w1449]
    tunnel: w89 -> [w1432]
    tunnel: w88 -> [w1438]
    tunnel: w87 -> [w1433]
    tunnel: w86 -> [w1430]
    tunnel: w85 -> [w1429]
    tunnel: w82 -> [_]
    tunnel: w79 -> [_]
    tunnel: w68 -> [_]
    tunnel: w66 -> [w1437]
    tunnel: w64 -> [w1431]
    tunnel: w61 -> [w1436]
    tunnel: w59 -> [_]
    tunnel: w55 -> [w1439]
    tunnel: [w1431] -> w45
    tunnel: [w1430] -> w44
    tunnel: [w1429] -> w43
    tunnel: [w1443] -> w42
    tunnel: [w1429] -> w41
    tunnel: [w1442] -> w40
    tunnel: [w1430] -> w39
    tunnel: [w1431] -> w38
    tunnel: [w1435] -> w37
    tunnel: [w1434] -> w36
    tunnel: [w1430] -> w35
    tunnel: [w1438] -> w34
    tunnel: [w1431] -> w33
    tunnel: [w1441] -> w32
    tunnel: [w1440] -> w31
    tunnel: [w1431] -> w30
    tunnel: [w1439] -> w29
    tunnel: [w1438] -> w28
    tunnel: [w1437] -> w27
    tunnel: [w1436] -> w26
    tunnel: [w1435] -> w25
    tunnel: [w1434] -> w24
    tunnel: [w1433] -> w23
    tunnel: [w1432] -> w22
    tunnel: [w1430] -> w21
    tunnel: [w1431] -> w20
    tunnel: [w1430] -> w19
    tunnel: [w1429] -> w18
    tunnel: ["local storage only"] -> w17
    tunnel: w51 -> [w1532]
    tunnel: [w1532] -> w50
    tunnel: w49 -> [w1531]
    tunnel: [w1531] -> w48
    tunnel: w47 -> [w1530]
    tunnel: [w1530] -> w46
    tunnel: w45 -> [w1527]
    tunnel: w44 -> [w1528]
    tunnel: w43 -> [w1529]
    tunnel: w42 -> [w1526]
    tunnel: w41 -> [w1525]
    tunnel: w40 -> [w1524]
    tunnel: w39 -> [w1523]
    tunnel: w38 -> [w1522]
    tunnel: w37 -> [w1517]
    tunnel: w36 -> [w1516]
    tunnel: w35 -> [w1521]
    tunnel: w34 -> [w1520]
    tunnel: w33 -> [w1519]
    tunnel: w32 -> [w1518]
    tunnel: w31 -> [w1515]
    tunnel: w30 -> [w1513]
    tunnel: w29 -> [w1514]
    tunnel: w28 -> [_]
    tunnel: w27 -> [_]
    tunnel: w26 -> [_]
    tunnel: w25 -> [_]
    tunnel: w24 -> [_]
    tunnel: w23 -> [w1512]
    tunnel: w22 -> [w1511]
    tunnel: w21 -> [w1510]
    tunnel: w20 -> [_]
    tunnel: w19 -> [_]
    tunnel: w18 -> [_]
    tunnel: w17 -> [w1509]
    tunnel: w50 -> [w1535]
    tunnel: w48 -> [w1534]
    tunnel: w46 -> [w1533]
    frame #0 {
      n409 = local read "single channel voltage array"() -> (w1164:dbl[])
      n410 = local read "No. of Samples:"() -> (w1189:u32)
      n411 = local read "real time P_rad array"() -> (w1158:dbl[])
      n412 = local read "full P_rad [MW] HBC"() -> (w1163:dbl[])
      n413 = local read "full P_rad [MW] VBC"() -> (w1162:dbl[])
      n414 = Subtract(x=w1189, y=1000) -> (x-y=w1160:u32)
      n415 = case "Correct timebase depending on if Trigger detected" shown="4294967295" w1190 {
        selector: w1190 -> [w1197 _]
        tunnel: [w1198 w1200] -> w1178
        tunnel: w1191 -> [w1196 _]
        frame Default {
          # "1 Trigger nur während OP"
          # "4294967295"
          # "Trigger deviation [ns]"
          # "Input Sample Frequency"
          n416 = Multiply(x=w1197, y=w1196) -> (x*y=w1195:i64)
          n417 = To Quad Integer(1:w1195) -> (0:w1198:i64)
        }
        frame 4294967295 {
          # "ms to ns conversion"
          # "4294967295\n=default if not Trigger"
          n418 = local read "data acquisition wait\ntime [ms]"() -> (w1199:i32)
          n419 = Multiply(x=i64 1000000, y=w1199) -> (x*y=w1200:i64)
        }
      }
      n420 = To Long Integer(number=w1160) -> (32bit integer=w1159:i32)
      n421 = call "Array_Trans.vi"("rohR [Ohm]"=w1167, "kappaR [A²]"=w1168, "Single Channel Voltage"=w1164, "rohM [Ohm]"=w1166, "tauR [s]"=w1156, "NSamples"=w1159, "offset [V]"=w1170, "kappaM [A²]"=w1169, "full P_rad VBC"=w1162, "full P_rad HBC"=w1163, "tauM [s]"=w1165, "real time P_rad"=w1158) -> ("full P_rad VBC"=w1161:dbl[][], "Mean [mV]"=w1181:dbl[][], "tauR [s]"=w1184:dbl[][], "rohR [Ohm]"=w1186:dbl[][], "real time P_rad"=w1157:dbl[][], "tauM [s]"=w1187:dbl[][], "kappa [A²]"=w1185:dbl[][], "full P_rad HBC"=w1172:dbl[][], "kappaR [A²]"=w1182:dbl[][], "rohM [Ohm]"=w1183:dbl[][], "Single Channel Voltage"=w1180:dbl[][])  [unwired: 5 in]
      n422 = local read "kbolott_and_volume"() -> (w1171:dbl[][])
    }
    frame #1 {
      n423 = control-ref of="DAQ Timer"() -> (w1224:refnum<vi>)
      n424 = call "W7X-Bolo-Timer.vi"("Wait-Time until Trigger\npublished on CODA\ntypically 10 s"=u32 1000 ("Wait-Time until Trigger; published on CODAC"), "Digital in"=w1224) -> ()  [unwired: 10 in]
      n425 = local write "state"("Wait for published Shot Time" ("state")) -> ()
    }
    frame #2 {
      n426 = case shown="0" "Trigger Source" {
        tunnel: [w1258 w1259] -> w1252
        frame 0 {
          n427 = call "GetTriggerTime.vi"() -> ("TriggerTime [ns]"=w1258:i64)  [unwired: 10 in, 1 out]
        }
        frame 1, Default {
          n428 = local read "start time POSIX [ns]"() -> (w1259:i64)
        }
      }
      "final trigger time" <- w1252
      n429 = local write "state"("Reading Trigger Time" ("state")) -> ()
    }
    frame #3 {
      w1277 = 1000
      w1323 = i64 -1  # Time Array needs to be positive!
      w1279 = 10000 ("dimension size")
      # "calibration sample time in ns  => 0.4 ms"
      # "DAQ start"
      # "10000"
      # "10000"
      # "offset the daq timing with\nthe excluded samples"
      # "time when DAQ started [ns]"
      # "TriggerT0"
      # "SampleRate in negative ns"
      # "Time array for Bolo Signal"
      # "Sample rate for Calibration Arrays\n should be hardwired to calirbation settings"
      # "Sample Rate in [ns]"
      # "NSample"
      # "Creating virtual Time Stamp\nfor Shot and for Calibration (Hardwired to 10000 samples)\nShot is depending on set sample rate"
      n430 = local read "predicted time [ms] to finalize DAQ"() -> (w1290:dbl)
      n431 = local read "Measured Time for DAQ [ms]"() -> (w1291:u32)
      n432 = local read "single channel signal factor"() -> (w1287:dbl)
      n433 = local read "single channel number"() -> (w1289:i64)
      n434 = local read "start time POSIX [ns]"() -> (w1288:i64)
      n435 = local read "loop DAQ timing [ms]"() -> (w1260:dbl)
      n436 = local read "sample time [s]"() -> (w1286:sgl)
      n437 = local read "Global DAC Range [mV] Setting"() -> (w1292:u8)
      n438 = local read "DAC and AD Settings"() -> (w1295:i32)
      n439 = local read "No. of Samples:"() -> (w1324:u32)
      n440 = Initialize Array(w1271, w1279) -> (w1321:i64[])
      n441 = Divide(x=sgl 1.0, y=w1286) -> (x/y=w1284:sgl)
      n442 = To Quad Integer(1:w1277) -> (0:w1276:i64)
      n443 = Multiply(x=w1276, y=w1268) -> (x*y=w1278:i64)
      n444 = Subtract(x=w1324, y=w1277) -> (x-y=w1302:u32)
      n445 = Multiply(x=w1278, y=i64 -1) -> (x*y=w1273:i64)
      n446 = Add(x=w1271, y=w1317) -> (x+y=w1274:i64)
      n447 = call "Parlog_creation.vi"("DAC Range Setting"=w1292, "DAC and AD Settings"=w1295, "loop DAQ timing [ms]"=w1260, "AD 7730 Bit Settings"=0, "predicted time [ms] to finalize DAQ"=w1290, "Measured Time for DAQ [ms]"=w1291, "start time"=w1288, "single channel voltage factor"=w1287, "Single Channel Voltage Output AO"=tag "Dev1/ao0:1" ("Single Channel Output AO"), "single channel number"=w1289, "maximum voltage @ 10MW single channel"=10.0, "sample_rate"=w1284, "pulse_length"=w1286, "sample_period"=w1286) -> ("cluster array"=w1261:T30)  [unwired: 7 in, 6 out]
      n448 = Multiply(x=w1268, y=w1323) -> (x*y=w1272:i64)
      n449 = Add(x=w1273, y=w1274) -> (x+y=w1262:i64)
      "DAQ start (POSIX) [ns]" <- w1262
      n450 = To Quad Integer(1:w1262) -> (0:w1319:i64)
      n451 = Replace Array Subset(array=i64[] [1399090569999999999, -1] ("dimensions"), new element=w1319, index=0) -> (w1299:i64[])
      n452 = local write "state"("Setting up time arrays and trigger" ("state")) -> ()
      n453 = Build Array(w1262) -> (w1298:i64[])
      n454 = Initialize Array(w1262, w1302) -> (w1320:i64[])
      n455 = Subtract(x=w1262, y=w1271) -> (x-y=→"Downtime after T0 until DAQ [ns]":i64)
      n456 = for {
        N: w1302 -> [_]
        shift-right: [w1335] -> w1300
        shift-left: w1320 -> [w1336]
        shift-right: [w1332] -> _
        shift-left: w1262 -> [w1333]
        tunnel: w1272 -> [w1331]
        i -> [w1334]
        n457 = Add(x=w1333, y=w1331) -> (x+y=w1332:i64)
        n458 = Replace Array Subset(array=w1336, new element=w1333, index=w1334) -> (w1335:i64[])
      }
      n459 = for {
        N: w1279 -> [_]
        shift-right: [w1329] -> w1301
        shift-left: w1321 -> [w1330]
        shift-right: [w1326] -> _
        shift-left: w1262 -> [w1327]
        tunnel: 400000 -> [w1325]
        i -> [w1328]
        n460 = Add(x=w1327, y=w1325) -> (x+y=w1326:i64)
        n461 = Replace Array Subset(array=w1330, new element=w1327, index=w1328) -> (w1329:i64[])
      }
    }
    frame #4 {
      w1346 = "Number"  # Unit
      w1355 = "Integer"  # datatype
      w1349 = "ChannelSelection"  # label
      w1362 = "V"  # Unit
      w1358 = "Float"  # datatype
      w1361 = "BoloSingleChannelFeedback"  # label
      w1365 = "A"  # Unit
      w1368 = 10000 ("sampleCount")
      w1370 = "Float"  # datatype
      w1367 = "BoloCalibMeasFoilFit"  # label
      w1375 = "A"  # Unit
      w1376 = 10000 ("sampleCount")
      w1378 = "Float"  # datatype
      w1374 = "BoloCalibRefFoilCurrent"  # label
      w1379 = 10000 ("sampleCount")
      w1386 = "Float"  # datatype
      w1383 = "A"  # Unit
      w1384 = "BoloCalibRefFoilFit"  # label
      w1391 = 1 ("sampleCount")
      w1394 = "Float"  # datatype
      w1392 = "W"  # Unit
      w1389 = "RKappa"  # label
      w1400 = 1 ("sampleCount")
      w1402 = "Float"  # datatype
      w1397 = "W"  # Unit
      w1399 = "MKappa"  # label
      w1408 = 1 ("sampleCount")
      w1410 = "Float"  # datatype
      w1405 = "Ohms"  # Unit
      w1407 = "RRes"  # label
      w1417 = 1 ("sampleCount")
      w1418 = "Float"  # datatype
      w1414 = "s"  # Unit
      w1416 = "RTau"  # label
      w1422 = 1 ("sampleCount")
      w1426 = "Float"  # datatype
      w1423 = "mV"  # Unit
      w1419 = "Offset"  # label
      # "DimensionB"
      # "DimensionC"
      # "DimensionC"
      # "DimensionC"
      # "DimensionC"
      # "DimensionC"
      # "DimensionC"
      # "BoloAdjusted"
      # "real time P_rad"
      # "full P_rad VBC"
      # "FullP_radVBC"
      # "A2"
      # "A"
      # "B"
      # "C"
      # "D"
      # "FullP_radHBCM"
      # "singleChannelVoltage"
      # "SampleFInt"
      # "samplePeriod"
      # "DimensionA: 10000 points at sampel time in nanoseconds and epoch time, for calibration etc.\n\nDimensionA2: Number of Samples\n\nDimensionB: [No. of Samples] points at sample time (epoch and nanoseconds) for measurement etc.\n\nDimensionC: Start time (epoch and nanoseconds) and -1 for until next entry\n\nDimensionD: Start time only"
      # "BoloPowerRaw"
      # "BoloSignal"
      # "BoloCalibRefFoilFit"
      # "kbolott&volume"
      # "HBCmPrad"
      # "SingleChannelFeedback"
      # "BoloCalibMeasFoilCurrent"
      # "BoloCalibRefFoilCurrent"
      # "BoloCalibMeasFoilFit"
      # "Offset"
      # "RKappa"
      # "RRes"
      # "RTau"
      # "MKappa"
      # "MRes"
      # "MTau"
      n462 = local read "sample time [s]"() -> (w1435:sgl)
      n463 = Reciprocal(x=w1435) -> (1/x=w1444:sgl)
      n464 = To Unsigned Word Integer(number=w1444) -> (unsigned 16bit integer=w1434:u16)
      n465 = local read "final channel selection"() -> (w1354:i64[][])
      n466 = Array Size(array=w1354) -> (size(s)=w1353:i32[])
      n467 = call "W7X2DJSON.vi"("values"=w1453, "label"=w1389, "dimensionSize"=w1391, "dimensions"=w1429, "dimensionCount"=128, "sampleCount"=w1391, "datatype"=w1394) -> ("JSON string"=w1390:string)  [unwired: 4 in]
      n468 = call "W7X2DJSON.vi"("values"=w1456, "label"=w1399, "dimensionSize"=w1400, "dimensions"=w1429, "dimensionCount"=128, "sampleCount"=w1400, "datatype"=w1402) -> ("JSON string"=w1398:string)  [unwired: 4 in]
      n469 = call "W7X2DJSON.vi"("values"=w1452, "label"=w1419, "dimensionSize"=w1422, "dimensions"=w1429, "dimensionCount"=128, "sampleCount"=w1422, "datatype"=w1426) -> ("JSON string"=w1424:string)  [unwired: 4 in]
      n470 = Index Array(array=w1353, index=0) -> (element=w1348:i32)
      n471 = Index Array(array=w1353, index=1) -> (element=w1350:i32)
      n472 = call "W7X2DJSON.vi"("values"=w1451, "label"=w1384, "dimensionSize"=w1379, "dimensions"=w1438, "dimensionCount"=128, "sampleCount"=w1379, "datatype"=w1386) -> ("JSON string"=w1382:string)  [unwired: 4 in]
      n473 = call "W7X2DJSON.vi"("values"=w1354, "label"=w1349, "dimensionSize"=w1348, "dimensions"=w1438, "dimensionCount"=w1350, "sampleCount"=w1348, "datatype"=w1355) -> ("JSON string"=w1347:string)  [unwired: 4 in]
      n474 = call "W7X1DPut.vi"("SigLabel"=w1389, "Unit"=w1392, "SigJSONbuffer"=w1390, "values"=w1431, "local storage only"="local storage only", "dimensions"=w1430) -> ("Parlog error out"=w1388:errorcluster)  [unwired: 4 in, 5 out]
      "RKappaErrorOut" <- w1388
      n475 = call "W7X1DPut.vi"("SigLabel"=w1419, "Unit"=w1423, "SigJSONbuffer"=w1424, "values"=w1431, "local storage only"="local storage only", "dimensions"=w1430) -> ("Parlog error out"=w1421:errorcluster)  [unwired: 4 in, 5 out]
      "OffsetErrorOut" <- w1421
      n476 = call "W7X1DPut.vi"("SigLabel"=w1399, "Unit"=w1397, "SigJSONbuffer"=w1398, "values"=w1431, "local storage only"="local storage only", "dimensions"=w1430) -> ("Parlog error out"=w1396:errorcluster)  [unwired: 4 in, 5 out]
      "MKappaErrorOut" <- w1396
      n477 = Unbundle(w1421) -> ("status"=→"Offset Status":bool)  [unwired: 2 out]
      n478 = Unbundle(w1388) -> ("status"=→"RKappa Status":bool)  [unwired: 2 out]
      n479 = Unbundle(w1396) -> ("status"=→"MKappa Status":bool)  [unwired: 2 out]
      n480 = call "W7X2DPut.vi"("SigLabel"=w1384, "SigJSONbuffer"=w1382, "values"=w1431, "sample rate"=w1434, "sample period"=w1435, "Unit"=w1383, "pulse_length"=w1435, "local storage only"="local storage only", "dimensions"=w1430) -> ("Parlog error out"=w1381:errorcluster)  [unwired: 5 in, 5 out]
      "BoloCalibRefFoilFitErrorOut" <- w1381
      n481 = call "W7X2DPut.vi"("SigLabel"=w1349, "SigJSONbuffer"=w1347, "values"=w1431, "Unit"=w1346, "local storage only"="local storage only", "dimensions"=w1430) -> ("Parlog error out"=w1344:errorcluster)  [unwired: 8 in, 5 out]
      "ChannelSelection ErrorOut" <- w1344
      n482 = Unbundle(w1381) -> ("status"=→"BoloCalibRefFoilFit Satus":bool)  [unwired: 2 out]
      n483 = Unbundle(w1344) -> ("status"=→"ChannelSelection status":bool)  [unwired: 2 out]
      n484 = call "W7X2DJSON.vi"("values"=w1455, "label"=w1416, "dimensionSize"=w1417, "dimensions"=w1429, "dimensionCount"=128, "sampleCount"=w1417, "datatype"=w1418) -> ("JSON string"=w1415:string)  [unwired: 4 in]
      n485 = call "W7X2DJSON.vi"("values"=w1454, "label"=w1407, "dimensionSize"=w1408, "dimensions"=w1429, "dimensionCount"=128, "sampleCount"=w1408, "datatype"=w1410) -> ("JSON string"=w1406:string)  [unwired: 4 in]
      n486 = call "W7X2DJSON.vi"("values"=w1445, "label"=w1361, "dimensionSize"=w1432, "dimensions"=w1433, "dimensionCount"=1, "sampleCount"=w1432, "datatype"=w1358) -> ("JSON string"=w1360:string)  [unwired: 4 in]
      n487 = call "W7X2DJSON.vi"("values"=w1447, "label"=w1367, "dimensionSize"=w1368, "dimensions"=w1438, "dimensionCount"=128, "sampleCount"=w1368, "datatype"=w1370) -> ("JSON string"=w1366:string)  [unwired: 4 in]
      n488 = call "W7X1DPut.vi"("SigLabel"=w1407, "Unit"=w1405, "SigJSONbuffer"=w1406, "values"=w1431, "local storage only"="local storage only", "dimensions"=w1430) -> ("Parlog error out"=w1404:errorcluster)  [unwired: 4 in, 5 out]
      "RResErrorOut" <- w1404
      n489 = call "W7X1DPut.vi"("SigLabel"=w1416, "Unit"=w1414, "SigJSONbuffer"=w1415, "values"=w1431, "local storage only"="local storage only", "dimensions"=w1430) -> ("Parlog error out"=w1412:errorcluster)  [unwired: 4 in, 5 out]
      "RTauErrorOut" <- w1412
      n490 = call "W7X2DJSON.vi"("values"=w1446, "label"=w1374, "dimensionSize"=w1376, "dimensions"=w1438, "dimensionCount"=128, "sampleCount"=w1376, "datatype"=w1378) -> ("JSON string"=w1373:string)  [unwired: 4 in]
      n491 = Unbundle(w1404) -> ("status"=→"RRes Status":bool)  [unwired: 2 out]
      n492 = Unbundle(w1412) -> ("status"=→"RTau Status":bool)  [unwired: 2 out]
      n493 = call "W7X2DPut.vi"("SigLabel"=w1367, "SigJSONbuffer"=w1366, "values"=w1431, "sample rate"=w1434, "sample period"=w1435, "Unit"=w1365, "pulse_length"=w1435, "local storage only"="local storage only", "dimensions"=w1430) -> ("Parlog error out"=w1364:errorcluster)  [unwired: 5 in, 5 out]
      "CalibMeasFoilFit 2" <- w1364
      n494 = Unbundle(w1364) -> ("status"=→"CalibMeasFoilFit status":bool)  [unwired: 2 out]
      n495 = call "W7X2DPut.vi"("SigLabel"=w1361, "SigJSONbuffer"=w1360, "values"=w1431, "sample rate"=w1434, "sample period"=w1435, "Unit"=w1362, "pulse_length"=w1435, "local storage only"="local storage only", "dimensions"=w1430) -> ("Parlog error out"=w1356:errorcluster)  [unwired: 5 in, 5 out]
      "SingleChannelFeedbackErrorOut" <- w1356
      n496 = call "parmsQSB.vi"("dimensions"=w1430, "values"=w1431, "label"="parms") -> ("JSON string"=w1338:string)
      n497 = case shown="False" "local storage only" {
        tunnel: [w1460 errorcluster {"status"=FALSE, "code"=0, "source"=""} ("error out")] -> w1342
        tunnel: w1338 -> [w1457 _]
        frame False {
          n498 = call <vilib>:"OpenHandle.vi"() -> ("client handle out"=w1467:T31, "error out"=w1466:errorcluster)  [unwired: 14 in]
          n499 = call <vilib>:"AddHeader.vi"("client handle"=w1467, "header"="Content-Type", "value"="application/json", "error in (no error)"=w1466) -> ("client handle out"=w1465:T31, "error out"=w1464:errorcluster)  [unwired: 10 in]
          n500 = call-poly <vilib>:"POST.vi"("client handle"=w1465, "url"="http://archive-webapi/Test/raw/W7X/QSB_Bolometry/File_PARLOG/", "buffer"=w1457, "error in (no error)"=w1464, "timeout (10000)"=400000 ("timeout for upload")) -> ("client handle out"=w1468:T31, "error out"=w1458:errorcluster)  [unwired: 7 in, 2 out]
          n501 = call <vilib>:"CloseHandle.vi"("client handle"=w1468, "error in (no error)"=w1458) -> ("error out"=w1460:errorcluster)  [unwired: 13 in]
        }
        frame True {
        }
      }
      n502 = call "W7X2DPut.vi"("SigLabel"=w1374, "SigJSONbuffer"=w1373, "values"=w1431, "sample rate"=w1434, "sample period"=w1435, "Unit"=w1375, "pulse_length"=w1435, "local storage only"="local storage only", "dimensions"=w1430) -> ("Parlog error out"=w1372:errorcluster)  [unwired: 5 in, 5 out]
      "CalibRefFoilCurrentErrorOut" <- w1372
      n503 = Unbundle(w1356) -> ("status"=→"SingleChannelFeedback status":bool)  [unwired: 2 out]
      n504 = Unbundle(w1372) -> ("status"=→"CalibRefFoilCurrent status":bool)  [unwired: 2 out]
      n505 = call "saveToFile.vi"("SigJSONbuffer"=w1338, "dimensions"=w1438, "String"="File_PARLOG" ("name or relative path")) -> ("error out"=w1339:errorcluster)  [unwired: 7 in, 1 out]
      n506 = Unbundle(w1339) -> ("status"=→"QSBParms status":bool)  [unwired: 2 out]
      n507 = local write "state"("Uploading to archive ...." ("state")) -> ()
      n508 = Merge Errors(w1342, w1339) -> (→"parms error out":errorcluster)
    }
    frame #5 {
      w1472 = 1 ("sampleCount")
      w1475 = "s"  # Unit
      w1477 = "Float"  # datatype
      w1474 = "MTau"  # label
      w1480 = 1 ("sampleCount")
      w1485 = "Float"  # datatype
      w1483 = "Ohms"  # Unit
      w1482 = "MRes"  # label
      w1490 = "A"  # Unit
      w1491 = 10000 ("sampleCount")
      w1493 = "Float"  # datatype
      w1489 = "BoloCalibMeasFoilCurrent"  # label
      w1500 = "V"  # Unit
      w1496 = "Float"  # datatype
      w1499 = "BoloRealTime_P_rad"  # label
      w1507 = "V"  # Unit
      w1503 = "Float"  # datatype
      w1506 = "BoloSignal"  # label
      # "DimensionC"
      # "DimensionC"
      # "DimensionC"
      # "DimensionB"
      n509 = call "W7X2DJSON.vi"("values"=w1518, "label"=w1489, "dimensionSize"=w1491, "dimensions"=w1520, "dimensionCount"=128, "sampleCount"=w1491, "datatype"=w1493) -> ("JSON string"=w1488:string)  [unwired: 4 in]
      n510 = call "W7X2DJSON.vi"("values"=w1524, "label"=w1482, "dimensionSize"=w1480, "dimensions"=w1525, "dimensionCount"=128, "sampleCount"=w1480, "datatype"=w1485) -> ("JSON string"=w1481:string)  [unwired: 4 in]
      n511 = call "W7X2DJSON.vi"("values"=w1515, "label"=w1506, "dimensionSize"=w1511, "dimensions"=w1512, "dimensionCount"=128, "sampleCount"=w1511, "datatype"=w1503) -> ("JSON string"=w1505:string)  [unwired: 4 in]
      n512 = call "W7X2DJSON.vi"("values"=w1526, "label"=w1474, "dimensionSize"=w1472, "dimensions"=w1529, "dimensionCount"=128, "sampleCount"=w1472, "datatype"=w1477) -> ("JSON string"=w1473:string)  [unwired: 4 in]
      n513 = call "W7X1DPut.vi"("SigLabel"=w1482, "Unit"=w1483, "SigJSONbuffer"=w1481, "values"=w1522, "local storage only"=w1509, "dimensions"=w1523) -> ("Parlog error out"=w1479:errorcluster)  [unwired: 4 in, 5 out]
      "MResErrorOut" <- w1479
      n514 = call "W7X2DPut.vi"("SigLabel"=w1506, "SigJSONbuffer"=w1505, "values"=w1513, "sample rate"=w1516, "sample period"=w1517, "Unit"=w1507, "pulse_length"=w1517, "local storage only"=w1509, "dimensions"=w1510) -> ("Parlog error out"=w1502:errorcluster)  [unwired: 5 in, 5 out]
      "BoloSignalErrorOut" <- w1502
      n515 = call "W7X2DPut.vi"("SigLabel"=w1489, "SigJSONbuffer"=w1488, "values"=w1519, "sample rate"=w1516, "sample period"=w1517, "Unit"=w1490, "pulse_length"=w1517, "local storage only"=w1509, "dimensions"=w1521) -> ("Parlog error out"=w1487:errorcluster)  [unwired: 5 in, 5 out]
      "CalibMeasFoilCurrentErrorOut" <- w1487
      n516 = call "W7X1DPut.vi"("SigLabel"=w1474, "Unit"=w1475, "SigJSONbuffer"=w1473, "values"=w1527, "local storage only"=w1509, "dimensions"=w1528) -> ("Parlog error out"=w1471:errorcluster)  [unwired: 4 in, 5 out]
      "MTauErrorOut" <- w1471
      n517 = Unbundle(w1479) -> ("status"=→"MRes status":bool)  [unwired: 2 out]
      n518 = local write "state"("Uploading to archive 2 ...." ("state")) -> ()
      n519 = Unbundle(w1502) -> ("status"=→"BoloSignal status":bool)  [unwired: 2 out]
      n520 = Unbundle(w1471) -> ("status"=→"MTau status":bool)  [unwired: 2 out]
      n521 = Unbundle(w1487) -> ("status"=→"CalibMeasFoilCurrent status":bool)  [unwired: 2 out]
      n522 = call "W7X2DJSON.vi"("values"=w1514, "label"=w1499, "dimensionSize"=w1511, "dimensions"=w1512, "dimensionCount"=1, "sampleCount"=w1511, "datatype"=w1496) -> ("JSON string"=w1498:string)  [unwired: 4 in]
      n523 = call "W7X2DPut.vi"("SigLabel"=w1499, "SigJSONbuffer"=w1498, "values"=w1513, "sample rate"=w1516, "sample period"=w1517, "Unit"=w1500, "pulse_length"=w1517, "local storage only"=w1509, "dimensions"=w1510) -> ("Parlog error out"=w1494:errorcluster)  [unwired: 5 in, 5 out]
      "RT_P_rad ErrorOut" <- w1494
      n524 = Unbundle(w1494) -> ("status"=→"RT_P_rad status":bool)  [unwired: 2 out]
    }
    frame #6 {
      n525 = local write "state"("Idle / Waiting for new Trigger" ("state")) -> ()
      n526 = case shown="True" w1535 {
        tunnel: w1534 -> [w1539 w1541]
        tunnel: w1533 -> [_ w1540]
        tunnel: [w1539 _] -> w1537
        frame False {
        }
        frame True {
          n527 = xnode "Close FPGA VI Reference"("FPGA VI Reference In"=w1541, "error in"=w1540) -> ()  [unwired: 1 out]
        }
      }
      "FPGA VI Reference Out" <- w1537
      n528 = property on="stop" class="Bool (strict)"("Val(Sgnl)"=TRUE) -> ()  [unwired: 2 in, 2 out]
    }
  }
